vi "Text control 2 v6.2_pump-specific.vi"() -> ()   [LabVIEW 2016]
panel:
  in  "Tab Control":enum32{"Main", "Other parameters"}(tab)
  out "Line running":i32
  out "Total lines":i32
  out "Path":path=path "C:/users/rlp38/09Apr2009LTtesting/test2.txt"
  out "I vs Vg":cluster{"Y data in":dbl[], "X data in":dbl[]}[](graph)
  out "Is max":dbl format="%.2e"
  out "Id max":dbl format="%.2e"
  out "Ig max":dbl format="%.2e"
  out "Imax vs time":cluster{"Y data in":dbl[], "X data in":dbl[]}[](graph)
  out "Imin vs time":cluster{"Y data in":dbl[], "X data in":dbl[]}[](graph)
  out "I vs Vd":cluster{"Y data in":dbl[], "X data in":dbl[]}[](graph)
  in  "Script":string="#-------------------------------------------------------\n# SPM pump cleaning script\n#\n# Version 0.5\n# Author: Dimitrios Simatos\n# Last updated: 2018-01-05\n#-------------------------------------------------------\n# Description\n#\n# This script is designed to run the cleaning sequence of the SPM OEM pump.\n# This script needs to be run 4 times!\n#-------------------------------------------------------\n# Changes\n#\n# Placed initialization and hard stop commands in the beginning.\n#-------------------------------------------------------\n# Important points\n#\n# Never leave any liquid in the pump to dry after the experiments. If they dry, the residue may block the valve.\n# Always run the cleaning cycle after the experiments.\n# Use clockwise rotation when going up in valve port numbers and vice versa.\n#-------------------------------------------------------\n# Things to do before running the script\n#\n# Set time units to minutes.\n# Set filenames.\n# Replace the tubing, if necessary.\n#-------------------------------------------------------\n# Port connections\n#\n# Port 1: Waste\n# Port 2: Waste\n# Port 3: Various cleaning liquids\n# Port 4: Waste\n# Port 5: Waste\n# Port 6: Waste\n#\n# Between each of the 4 runs, the settings of Port 3 will change, according to the cleaning protocol.\n# The settings for Port 3 are:\n# 1st run: 1% v/v solution of sodium hypochlorite in ultrapure water\n# 2nd run: 0.1% w/v solution of sodium dodecyl sulfate in ultrapure water\n# 3rd run: Ultrapure water\n# 4th run: Waste (in air, not immersed in liquid)\n#-------------------------------------------------------\n# Cleaning protocol for the SPM OEM pump (from the manual)\n#\n# A cleaning procedure should be performed at the end of each day or in between two different experiments.\n# An effective cleaning can be performed in the following manner:\n# • Bleach solution to kill microorganisms\n# 1. Prepare a solution of 1% chlorine bleach and deionized water\n#    NOTE: Prepare a 1% v/v solution of sodium hypochlorite in deionized water\n# 2. Prepare a reservoir and place 1 tubing in the bleach solution and 5 tubings in a waste recipient\n# 3. Pick up the bleach solution through 1 port to entirely fill the syringe\n# 4. Sequentially output the syringe content through the remaining ports and throw it to the waste\n# 5. Repeat operation at least 2 times\n# • Detergent solution to remove debris\n# 1. Prepare a solution of 0.1% detergent and deionized water\n#    NOTE: Prepare a 0.1% w/v solution of sodium dodecyl sulfate in deionized water\n# 2. Move the tubing from the bleach solution reservoir and place it into a reservoir of detergent solution\n# 3. Pick up the detergent solution through 1 port to entirely fill the syringe\n# 4. Sequentially output the detergent solution through the remaining ports into the waste recipient\n# 5. Repeat operation at least 2 times\n# • Rinsing water to prepare the pump for your next experiment\n# 1. Move the tubing from the detergent solution reservoir and place it into a reservoir of deionized water\n# 2. Pick up the rinsing solution through 1 port to entirely fill the syringe\n# 3. Sequentially output the rinse water through the remaining ports into the waste recipient\n# 4. Repeat operation at least 2 times\n# • Replace the tubing, if necessary\n#-------------------------------------------------------\n# Pumping cycles and execution time\n#\n# Execution time for a single cycle: 6 x (1 min + 10 sec) = 7 minutes\n# Total execution time: 4 x 7 = 28 minutes\n# Since the script has to run 4 times, the cleaning lasts for: 4 x 28 = 112 minutes\n# Air must be the last to be pumped through the valve, to remove all liquids.\n# There are 4 pumping cycles. Each one draws a different liquid through port 3 and pumps it sequentially through ports 1,2,4,5,6.\n# During the sequential pumping, each port receives 200 ml of liquid (20% of the total syringe volume = 600 \"plunger units\")\n# The device must be disconnected from the port during the cleaning procedure.\n# All cycles are similar, except cycle 1 has the initialization command uncommented and the first report valve command commented.\n#-------------------------------------------------------\n# Volume of liquid needed\n#\n# Volume of liquid needed per cycle: 1 ml\n# Total volume of liquid needed per script run: 4 x 1 = 4 ml\n# Since the script has to run 4 times, the first 3 with different liquids, I need:\n# 4 ml of 1% v/v solution of sodium hypochlorite in ultrapure water\n# 4 ml of 0.1% w/v solution of sodium dodecyl sulfate in ultrapure water\n# 4 ml of ultrapure water\n#-------------------------------------------------------\n# Parameters\n#\n# Syringe size: 1 ml\n# Step resolution N = 0.01 mm\n# Drawing flow V = 300 pulses/second (6000 ul/min)\n# Pumping flow V = 300 pulses/second (6000 ul/min)\n#-------------------------------------------------------\n# Pump initialization\npump /1T #hard stop pump\npump /1ZR #initialize pump\n#-------------------------------------------------------\n# Cycle 1\n# Fill the syringe\npump /1Q #query pump\npump /1? #report absolute plunger position\n#pump /1?6 #report valve position\nwait-min 1 #wait 1 minute\npump /1N0R #set step resolution: 0.01 mm\npump /1Q #query pump\npump /1? #report absolute plunger position (the plunger should be at 0)\npump /1?6 #report valve position\nwait 1000 #wait 1 second\npump /1V300R #choose speed: 300 steps/s (6000 ul/min)\npump /1Q #query pump\nwait 1000 #wait 1 second\npump /1I3R #go to port 3, clockwise rotation\npump /1Q #query pump\npump /1?6 #report valve position\nwait 1000 #wait 1 second\npump /1A3000R #go to absolute position 3000 (= draw 1 ml)\nwait 30000 #wait 30 seconds\npump /1Q #query pump\npump /1? #report absolute plunger position (the plunger should have finished moving)\n#pump /1?6 #report valve position\n# The sequential pumping begins\n# Port 1\npump /1O1R #switch to port 1, counterclockwise rotation\npump /1Q #query pump\npump /1?6 #report valve position\npump /1A2400R #go to absolute position 2400 (= pump 200 ul)\npump /1Q #query pump\npump /1? #report absolute plunger position (the plunger should be moving to 0)\nwait-min 1 #wait 1 minute\npump /1? #report absolute plunger position (the plunger should have finished moving)\n# Port 2\npump /1I2R #switch to port 2, clockwise rotation\npump /1Q #query pump\npump /1?6 #report valve position\npump /1A1800R #go to absolute position 1800 (= pump 200 ul)\npump /1Q #query pump\npump /1? #report absolute plunger position (the plunger should be moving to 0)\nwait-min 1 #wait 1 minute\npump /1? #report absolute plunger position (the plunger should have finished moving)\n# Port 4\npump /1I4R #switch to port 4, clockwise rotation\npump /1Q #query pump\npump /1?6 #report valve position\npump /1A1200R #go to absolute position 1200 (= pump 200 ul)\npump /1Q #query pump\npump /1? #report absolute plunger position (the plunger should be moving to 0)\nwait-min 1 #wait 1 minute\npump /1? #report absolute plunger position (the plunger should have finished moving)\n# Port 5\npump /1I5R #switch to port 5, clockwise rotation\npump /1Q #query pump\npump /1?6 #report valve position\npump /1A600R #go to absolute position 600 (= pump 200 ul)\npump /1Q #query pump\npump /1? #report absolute plunger position (the plunger should be moving to 0)\nwait-min 1 #wait 1 minute\npump /1? #report absolute plunger position (the plunger should have finished moving)\n# Port 6\npump /1I6R #switch to port 6, clockwise rotation\npump /1Q #query pump\npump /1?6 #report valve position\npump /1A0R #go to absolute position 0 (= pump 200 ul)\npump /1Q #query pump\npump /1? #report absolute plunger position (the plunger should be moving to 0)\nwait-min 1 #wait 1 minute\npump /1? #report absolute plunger position (the plunger should have finished moving)\n#-------------------------------------------------------\n# Cycle 2\n# Fill the syringe\n#pump /1ZR #initialize pump\npump /1Q #query pump\npump /1? #report absolute plunger position\npump /1?6 #report valve position\nwait-min 1 #wait 1 minute\npump /1N0R #set step resolution: 0.01 mm\npump /1Q #query pump\npump /1? #report absolute plunger position (the plunger should be at 0)\npump /1?6 #report valve position\nwait 1000 #wait 1 second\npump /1V300R #choose speed: 300 steps/s (6000 ul/min)\npump /1Q #query pump\nwait 1000 #wait 1 second\npump /1O3R #go to port 3, counterclockwise rotation\npump /1Q #query pump\npump /1?6 #report valve position\nwait 1000 #wait 1 second\npump /1A3000R #go to absolute position 3000 (= draw 1 ml)\nwait 30000 #wait 30 seconds\npump /1Q #query pump\npump /1? #report absolute plunger position (the plunger should have finished moving)\n#pump /1?6 #report valve position\n# The sequential pumping begins\n# Port 1\npump /1O1R #switch to port 1, counterclockwise rotation\npump /1Q #query pump\npump /1?6 #report valve position\npump /1A2400R #go to absolute position 2400 (= pump 200 ul)\npump /1Q #query pump\npump /1? #report absolute plunger position (the plunger should be moving to 0)\nwait-min 1 #wait 1 minute\npump /1? #report absolute plunger position (the plunger should have finished moving)\n# Port 2\npump /1I2R #switch to port 2, clockwise rotation\npump /1Q #query pump\npump /1?6 #report valve position\npump /1A1800R #go to absolute position 1800 (= pump 200 ul)\npump /1Q #query pump\npump /1? #report absolute plunger position (the plunger should be moving to 0)\nwait-min 1 #wait 1 minute\npump /1? #report absolute plunger position (the plunger should have finished moving)\n# Port 4\npump /1I4R #switch to port 4, clockwise rotation\npump /1Q #query pump\npump /1?6 #report valve position\npump /1A1200R #go to absolute position 1200 (= pump 200 ul)\npump /1Q #query pump\npump /1? #report absolute plunger position (the plunger should be moving to 0)\nwait-min 1 #wait 1 minute\npump /1? #report absolute plunger position (the plunger should have finished moving)\n# Port 5\npump /1I5R #switch to port 5, clockwise rotation\npump /1Q #query pump\npump /1?6 #report valve position\npump /1A600R #go to absolute position 600 (= pump 200 ul)\npump /1Q #query pump\npump /1? #report absolute plunger position (the plunger should be moving to 0)\nwait-min 1 #wait 1 minute\npump /1? #report absolute plunger position (the plunger should have finished moving)\n# Port 6\npump /1I6R #switch to port 6, clockwise rotation\npump /1Q #query pump\npump /1?6 #report valve position\npump /1A0R #go to absolute position 0 (= pump 200 ul)\npump /1Q #query pump\npump /1? #report absolute plunger position (the plunger should be moving to 0)\nwait-min 1 #wait 1 minute\npump /1? #report absolute plunger position (the plunger should have finished moving)\n#-------------------------------------------------------\n# Cycle 3\n# Fill the syringe\n#pump /1ZR #initialize pump\npump /1Q #query pump\npump /1? #report absolute plunger position\npump /1?6 #report valve position\nwait-min 1 #wait 1 minute\npump /1N0R #set step resolution: 0.01 mm\npump /1Q #query pump\npump /1? #report absolute plunger position (the plunger should be at 0)\npump /1?6 #report valve position\nwait 1000 #wait 1 second\npump /1V300R #choose speed: 300 steps/s (6000 ul/min)\npump /1Q #query pump\nwait 1000 #wait 1 second\npump /1O3R #go to port 3, counterclockwise rotation\npump /1Q #query pump\npump /1?6 #report valve position\nwait 1000 #wait 1 second\npump /1A3000R #go to absolute position 3000 (= draw 1 ml)\nwait 30000 #wait 30 seconds\npump /1Q #query pump\npump /1? #report absolute plunger position (the plunger should have finished moving)\n#pump /1?6 #report valve position\n# The sequential pumping begins\n# Port 1\npump /1O1R #switch to port 1, counterclockwise rotation\npump /1Q #query pump\npump /1?6 #report valve position\npump /1A2400R #go to absolute position 2400 (= pump 200 ul)\npump /1Q #query pump\npump /1? #report absolute plunger position (the plunger should be moving to 0)\nwait-min 1 #wait 1 minute\npump /1? #report absolute plunger position (the plunger should have finished moving)\n# Port 2\npump /1I2R #switch to port 2, clockwise rotation\npump /1Q #query pump\npump /1?6 #report valve position\npump /1A1800R #go to absolute position 1800 (= pump 200 ul)\npump /1Q #query pump\npump /1? #report absolute plunger position (the plunger should be moving to 0)\nwait-min 1 #wait 1 minute\npump /1? #report absolute plunger position (the plunger should have finished moving)\n# Port 4\npump /1I4R #switch to port 4, clockwise rotation\npump /1Q #query pump\npump /1?6 #report valve position\npump /1A1200R #go to absolute position 1200 (= pump 200 ul)\npump /1Q #query pump\npump /1? #report absolute plunger position (the plunger should be moving to 0)\nwait-min 1 #wait 1 minute\npump /1? #report absolute plunger position (the plunger should have finished moving)\n# Port 5\npump /1I5R #switch to port 5, clockwise rotation\npump /1Q #query pump\npump /1?6 #report valve position\npump /1A600R #go to absolute position 600 (= pump 200 ul)\npump /1Q #query pump\npump /1? #report absolute plunger position (the plunger should be moving to 0)\nwait-min 1 #wait 1 minute\npump /1? #report absolute plunger position (the plunger should have finished moving)\n# Port 6\npump /1I6R #switch to port 6, clockwise rotation\npump /1Q #query pump\npump /1?6 #report valve position\npump /1A0R #go to absolute position 0 (= pump 200 ul)\npump /1Q #query pump\npump /1? #report absolute plunger position (the plunger should be moving to 0)\nwait-min 1 #wait 1 minute\npump /1? #report absolute plunger position (the plunger should have finished moving)\n#-------------------------------------------------------\n# Cycle 4\n# Fill the syringe\n#pump /1ZR #initialize pump\npump /1Q #query pump\npump /1? #report absolute plunger position\npump /1?6 #report valve position\nwait-min 1 #wait 1 minute\npump /1N0R #set step resolution: 0.01 mm\npump /1Q #query pump\npump /1? #report absolute plunger position (the plunger should be at 0)\npump /1?6 #report valve position\nwait 1000 #wait 1 second\npump /1V300R #choose speed: 300 steps/s (6000 ul/min)\npump /1Q #query pump\nwait 1000 #wait 1 second\npump /1O3R #go to port 3, counterclockwise rotation\npump /1Q #query pump\npump /1?6 #report valve position\nwait 1000 #wait 1 second\npump /1A3000R #go to absolute position 3000 (= draw 1 ml)\nwait 30000 #wait 30 seconds\npump /1Q #query pump\npump /1? #report absolute plunger position (the plunger should have finished moving)\n#pump /1?6 #report valve position\n# The sequential pumping begins\n# Port 1\npump /1O1R #switch to port 1, counterclockwise rotation\npump /1Q #query pump\npump /1?6 #report valve position\npump /1A2400R #go to absolute position 2400 (= pump 200 ul)\npump /1Q #query pump\npump /1? #report absolute plunger position (the plunger should be moving to 0)\nwait-min 1 #wait 1 minute\npump /1? #report absolute plunger position (the plunger should have finished moving)\n# Port 2\npump /1I2R #switch to port 2, clockwise rotation\npump /1Q #query pump\npump /1?6 #report valve position\npump /1A1800R #go to absolute position 1800 (= pump 200 ul)\npump /1Q #query pump\npump /1? #report absolute plunger position (the plunger should be moving to 0)\nwait-min 1 #wait 1 minute\npump /1? #report absolute plunger position (the plunger should have finished moving)\n# Port 4\npump /1I4R #switch to port 4, clockwise rotation\npump /1Q #query pump\npump /1?6 #report valve position\npump /1A1200R #go to absolute position 1200 (= pump 200 ul)\npump /1Q #query pump\npump /1? #report absolute plunger position (the plunger should be moving to 0)\nwait-min 1 #wait 1 minute\npump /1? #report absolute plunger position (the plunger should have finished moving)\n# Port 5\npump /1I5R #switch to port 5, clockwise rotation\npump /1Q #query pump\npump /1?6 #report valve position\npump /1A600R #go to absolute position 600 (= pump 200 ul)\npump /1Q #query pump\npump /1? #report absolute plunger position (the plunger should be moving to 0)\nwait-min 1 #wait 1 minute\npump /1? #report absolute plunger position (the plunger should have finished moving)\n# Port 6\npump /1I6R #switch to port 6, clockwise rotation\npump /1Q #query pump\npump /1?6 #report valve position\npump /1A0R #go to absolute position 0 (= pump 200 ul)\npump /1Q #query pump\npump /1? #report absolute plunger position (the plunger should be moving to 0)\nwait-min 1 #wait 1 minute\npump /1? #report absolute plunger position (the plunger should have finished moving)\n#-------------------------------------------------------"
  out "Command running:":string
  out "Serial port data":string
  out "Elapsed Time":dbl caption="Elapsed Time (s)"
  in  "Time Units":u16(ring)=1 items=["Seconds", "Minutes", "Hours"]
  in  "Time Offset":dbl caption="Set Start Time (s)"
  in  "Reset":bool
  in  "Auto Reset":bool
  in  "integration time":u32(slide) max=2 step=1 scale=0.0..2.0
  in  "Interrupt scan":bool
  out "Absolute plunger position vs time":cluster{"Y data in":dbl[], "X data in":dbl[]}[](graph)
  out "Valve position vs time":cluster{"Y data in":dbl[], "X data in":dbl[]}[](graph)
  out "Is on":dbl format="%.2e"
  out "Id on":dbl format="%.2e"
  out "Ig on":dbl format="%.2e"
  out "Ion vs time":cluster{"Y data in":dbl[], "X data in":dbl[]}[](graph)
  out "Ioff vs time":cluster{"Y data in":dbl[], "X data in":dbl[]}[](graph)
  out "Ig min":dbl format="%.2e"
  out "Id min":dbl format="%.2e"
  out "Is min":dbl format="%.2e"
  out "Is off":dbl format="%.2e"
  out "Id off":dbl format="%.2e"
  out "Ig off":dbl format="%.2e"
  in  "Integration time (long)":dbl=0.32 min=0.04 max=2.0 step=0.02 format="%.2f"
  in  "Integration time (short)":dbl=0.0019 min=8e-05 max=0.0019 step=8e-05 format="%^.0e"
  in  "Gate: Compliance":dbl=0.001 format="%.8f"
  in  "Drain: Compliance":dbl=0.001 format="%.8f"
  in  "Hard stop pump":bool
  in  "Halt pump":bool
  in  "Interrupt program":bool
  in  "Gate Range\nmode":u16(ring) items=["Auto", "Limited", "Fixed"]
  in  "Gate Range":u8(slide)=6 max=11 scale=0.0..11.0
  in  "Source/Drain\nRange mode":u16(ring) items=["Auto", "Limited", "Fixed"]
  in  "Source/Drain Range":u8(slide)=6 max=11 scale=0.0..11.0
  in  "Panel Controls":T1={"Emergency Stop"=refnum, "TransGraph Max"=1e-05, "Text/Graph (text=false)"=TRUE} {"TransGraph Max" format="%.2e"}
  in  "Panel Controls 2":T2={"Emergency Stop"=refnum, "TransGraph Max"=1e-05, "Text/Graph (text=false)"=TRUE, "TransGraph Min"=1e-11} {"TransGraph Min" format="%.2e"; "TransGraph Max" format="%.2e"}
  in  "SMU4":cluster{"on/off":bool, "Voltage":dbl} {"Voltage" min=-100.0 max=100.0 format="%.2f"}
  in  "Full Reset":bool
  in  "Standby":T3
  out "error out":errorcluster
  in  "Delay before read (ms)":u32=1000
  in  "byte count":u32=64
  in  "Serial End Mode for Reads":u16(ring)=2 items=["None", "LastBit", "TermChar"]
  in  "Timeout (ms)":u32=10000
  in  "Enable Termination\nChar (T)":bool=TRUE
  in  "Termination char\n(0xA = '\\n' = LF)\n(0xD = '\\r' = CR)":u8=13 format="%.0x"
  in  "flow control":u16(ring) items=["None"=0, "XON/XOFF"=1, "RTS/CTS"=2, "DTR/DSR"=4]
  in  "stop bits":u16(ring)=10 items=["1.0"=10, "1.5"=15, "2.0"=20]
  in  "parity":u16(ring) items=["None", "Odd", "Even", "Mark", "Space"]
  in  "data bits":u16=8 min=5 max=8 step=1
  in  "VISA resource name":refnum<visa-resource-name>="COM6"
  in  "baud rate":u32=9600
  in  "Filename (variable part)":string="step_1_up-H2O_initial_"
  in  "Suffix (script)":string="step_1_up-H2O_initial_script.txt"
  out "Timings Indicator":T4
  in  "Timings (overwritten by the Front Panel)":T5={"integration time"=0, "Short/Long integration time"=0.00064, "hold time (sec)"=0.0, "delay time (sec)"=0.0, "Step Time (0 disables)"=0.0, "sweep method"=0, "Pulse period"=0.005, "Base voltage"=0.0, "Pulse width"=0.0005} {"Pulse width" min=0.0005 max=0.1 step=0.0001 format="%.4f"; "Base voltage" format="%^.4e"; "Pulse period" min=0.005 max=1.0 step=0.0001 format="%.4f"; "sweep method" items=["Continuous", "Pulsed"]; "Step Time (0 disables)" format="%.2f"; "delay time (sec)" format="%.4f"; "hold time (sec)" format="%.4f"; "Short/Long integration time" format="%^.0e"; "integration time" scale=0.0..2.0}
  in  "Gate":T6={"Gate Start"=0.0, "Gate Stop"=2.0, "Gate Step (linear only)"=1.0, "Gate Compliance"=0.0001, "Gate PComp"=0.0, "Range mode"=0, "Range"=6} {"Range" max=11 scale=0.0..11.0; "Range mode" items=["Auto", "Limited", "Fixed"]; "Gate PComp" format="%^.2e"; "Gate Compliance" format="%^.2e"; "Gate Step (linear only)" format="%^.4e"; "Gate Stop" format="%^.4e"; "Gate Start" format="%^.4e"}
  in  "Drain 2":T7={"Drain Start"=0.0, "Drain Stop"=2.0, "Drain Compliance"=0.0001, "Drain Step"=1.0, "Drain PComp"=0.0, "Range mode"=0, "Range"=6} {"Range" max=11 scale=0.0..11.0; "Range mode" items=["Auto", "Limited", "Fixed"]; "Drain PComp" format="%^.2e"; "Drain Step" format="%^.4e"; "Drain Compliance" format="%^.2e"; "Drain Stop" format="%^.4e"; "Drain Start" format="%^.4e"}
  # "Syntax:\nitime [s|m|l] time(sec): [s|m|l] determines the integration time setting (small|medium|long) and time sets the value.\nNOTE: The value of the integration time has to be within the range allowed by its category (s|m|l), otherwise, the closest value will be used. (e.g. if the category is set to short but the time value is very long, the actual value used will be the maximum short integration time.\nIntegration times:\n    Short: Default: 640 us. Range: 8E-5 - 1.92E-3 seconds.\n    Medium: Fixed at 1 NPL cycle (0.02 seconds).\n    Long: Default: 16 NPL cycles (0.32 seconds). Range: 2-100 NPL cycles (0.04 seconds - 2 seconds).\ngaterangemode [a|l|f]\ndrainrangemode [a|l|f]\npulsed [on|off] PulsePeriod(sec) PulseBaseVoltage PulseONWidth(sec)\nstandby [on l off]\nwait NumMilliseconds\nwait-min NumMinutes\n# texthere = comment\ntransfer [s|d] VgStart VgStop VgStep VdStart VdStop VdStep\noutput [s|d] VgStart VgStop VgStep VdStart VdStop VdStep\nsample Vg Vd NumSamples Time(s) SampleInterval(s)\nsamplei Idg NumSamples Time(s) SampleInterval(s) VDGcompliance\n100 samples is approximately 13 seconds with medium integration\n# if in doubt use SampleInterval(s) = 0.004\nstressV VG VD IGcompliance IDcompliance Duration(sec)\nstressI IDG VDGcompliance Duration(sec)\nvsu2pulse Bias Duration(s)\npulsedstressV [s|d] VEstop VgON VgOFF Period(s) PulseONwidth(s) Vd\nsample-fpp Vg Vd NumSamples Time\nresample-fpp Vg Vd\ntransfer-fpp [s|d] VgStart VgStop VgStep VdStart VdStop VdStep\noutput-fpp [s|d] VgStart VgStop VgStep VdStart VdStop VdStep\nserial SerialPortCommand\npump SerialPortCommand for the SPM pump\n\nSPM Pump Syntax (<x>: pump number, use 1 if only one pump):\nif the command syntax contains [R], then append the letter R to the command\n/<x>Q: query (a query command should follow each command)\n/<x>Z[R] or /<x>Y[R]: initialize pump\n/<x>N<n>[R] (<n>=0,1): <0> (<1>) microstep 0.01 mm (0.00125 mm) resolution\n/<x>I<n> (<n>=0-6): turn to port number n (clockwise)\n/<x>O<n> (<n>=0-6): turn to port number n (counterclockwise)\n/<x>X: Re-execute last command string\n/<x>G<n>[R] (<n>=0-60000): repeat command sequence (default: 0, 0=loop forever)\n/<x>g: Mark the start of a repeat sequence (max = 10)\n/<x>M<n>[R] (<n>=0-86400000): delay command execution by n milliseconds\n/<x>H: Halt; Pause the sequence after finishing the current move\n/<x>T: Hardstop; Interrupt the current move and suppress it from the sequence\n/<x>A<n>[R] (<n>=0-3000 with N=0, 0-24000 with N=1): absolute position\n/<x>P<n>[R] (<n>=0-3000 with N=0, 0-24000 with N=1): relative pickup\n/<x>D<n>[R] (<n>=0-3000 with N=0, 0-24000 with N=1): relative dispense\n/<x>V<n>[R] (<n>=1-1600 default: 150): set peak speed (pulses/sec)\nNOTE: The lowest speed limit is 1 pulse/sec, not 5, as the manual states.\n/<x>S<n>[R] (<n>=10-40 default: 22): set speed (NOT in pulses/sec, look in manual)\nNOTE: When controlled with absolute position, one does not need to pay special attention to the syringe that is mounted on the pump.\nWithdraw from lower stage (ports 3, 5), dispense from higher stage (ports 2, 4, 6).\nConnect Port 1 to waste."
  # "Time"
  # "1\n2\n3\n4\n5\n6\n7\n8\n9\n10\n11\n12\n13\n14\n15\n16\n17\n18\n19\n20"
  # "Serial port settings"
  # "Filename settings"
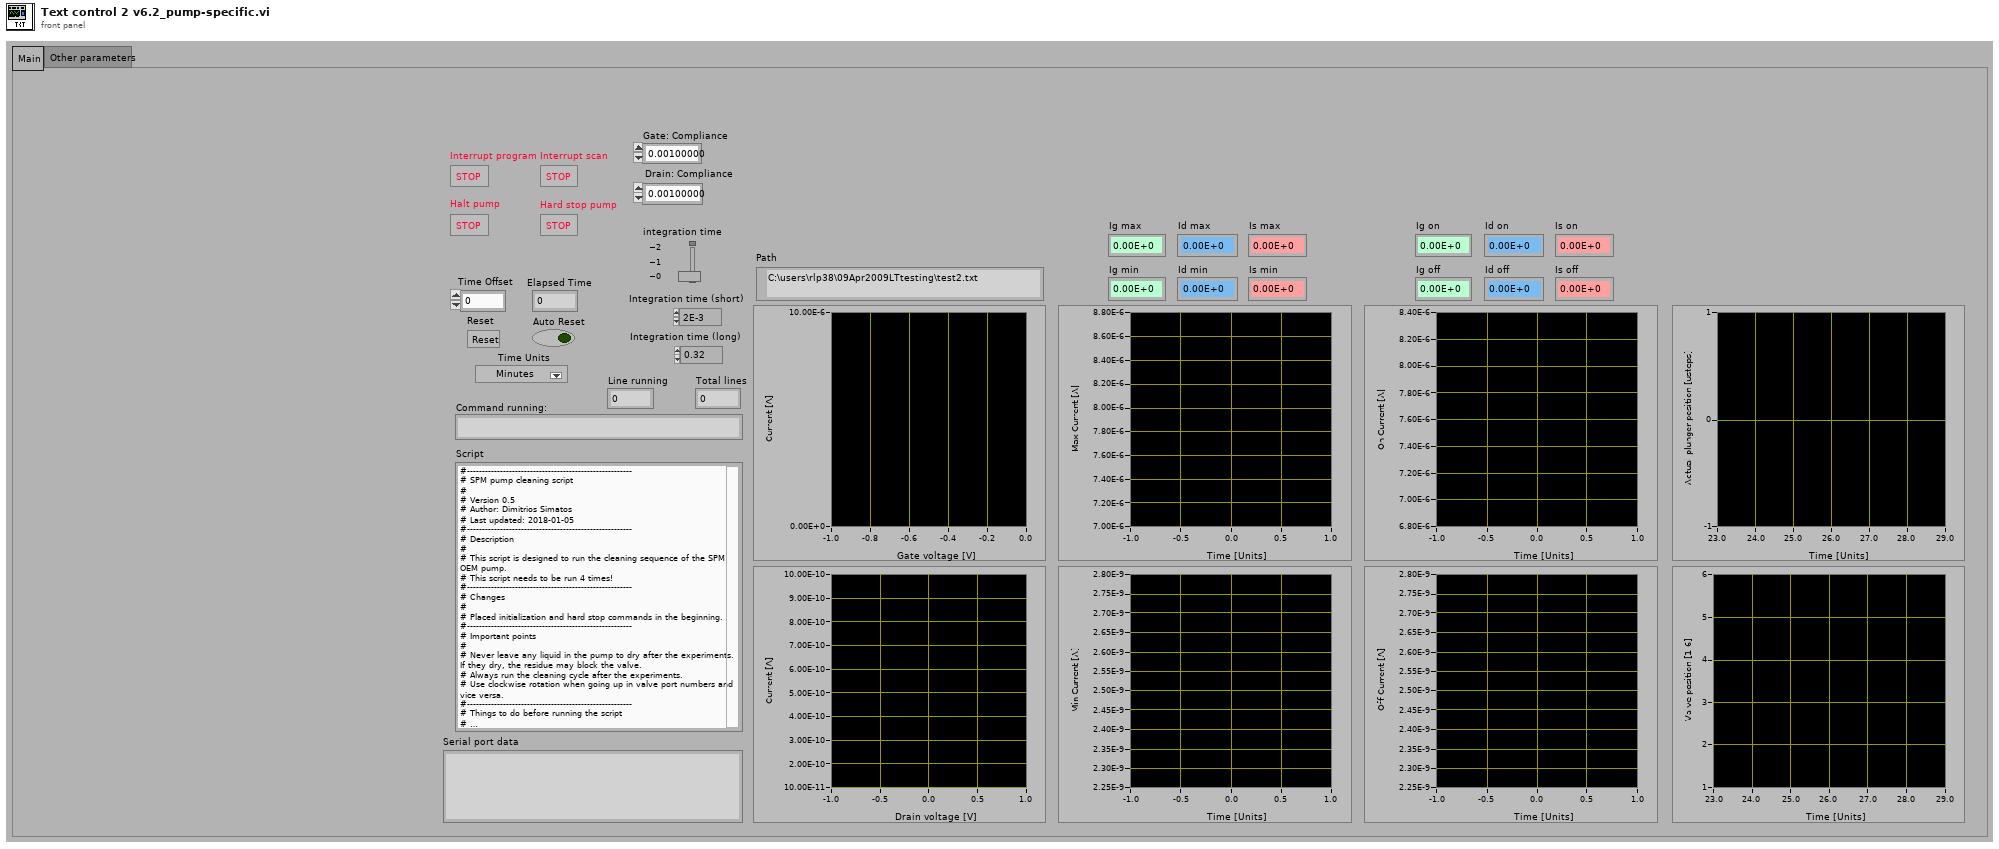
[diagram p1: front panel]
types:
  T1 = cluster{"Emergency Stop":refnum<vi>, "TransGraph Max":dbl, "Text/Graph (text=false)":bool}
  T2 = cluster{"Emergency Stop":refnum<vi>, "TransGraph Max":dbl, "Text/Graph (text=false)":bool, "TransGraph Min":dbl}
  T3 = cluster{"Gate Standby":bool, "Drain Standby":bool}
  T4 = cluster{"integration time (0:s, 1:m, 2:l)":u32, "Short/Long integration time":dbl, "hold time (sec)":dbl, "delay time (sec)":dbl, "Step Time (0 disables)":dbl, "sweep method":u16, "Pulse period":dbl, "Base voltage":dbl, "Pulse width":dbl}
  T5 = cluster{"integration time":u32, "Short/Long integration time":dbl, "hold time (sec)":dbl, "delay time (sec)":dbl, "Step Time (0 disables)":dbl, "sweep method":u16, "Pulse period":dbl, "Base voltage":dbl, "Pulse width":dbl}
  T6 = cluster{"Gate Start":dbl, "Gate Stop":dbl, "Gate Step (linear only)":dbl, "Gate Compliance":dbl, "Gate PComp":dbl, "Range mode":u16, "Range":u8}
  T7 = cluster{"Drain Start":dbl, "Drain Stop":dbl, "Drain Compliance":dbl, "Drain Step":dbl, "Drain PComp":dbl, "Range mode":u16, "Range":u8}
  T8 = enum16{"open", "replace", "create", "open or create", "replace or create", "replace or create with confirmation"}
  T9 = cluster{"V2 Start":dbl, "V2 Step":dbl, "Number of points":i32}
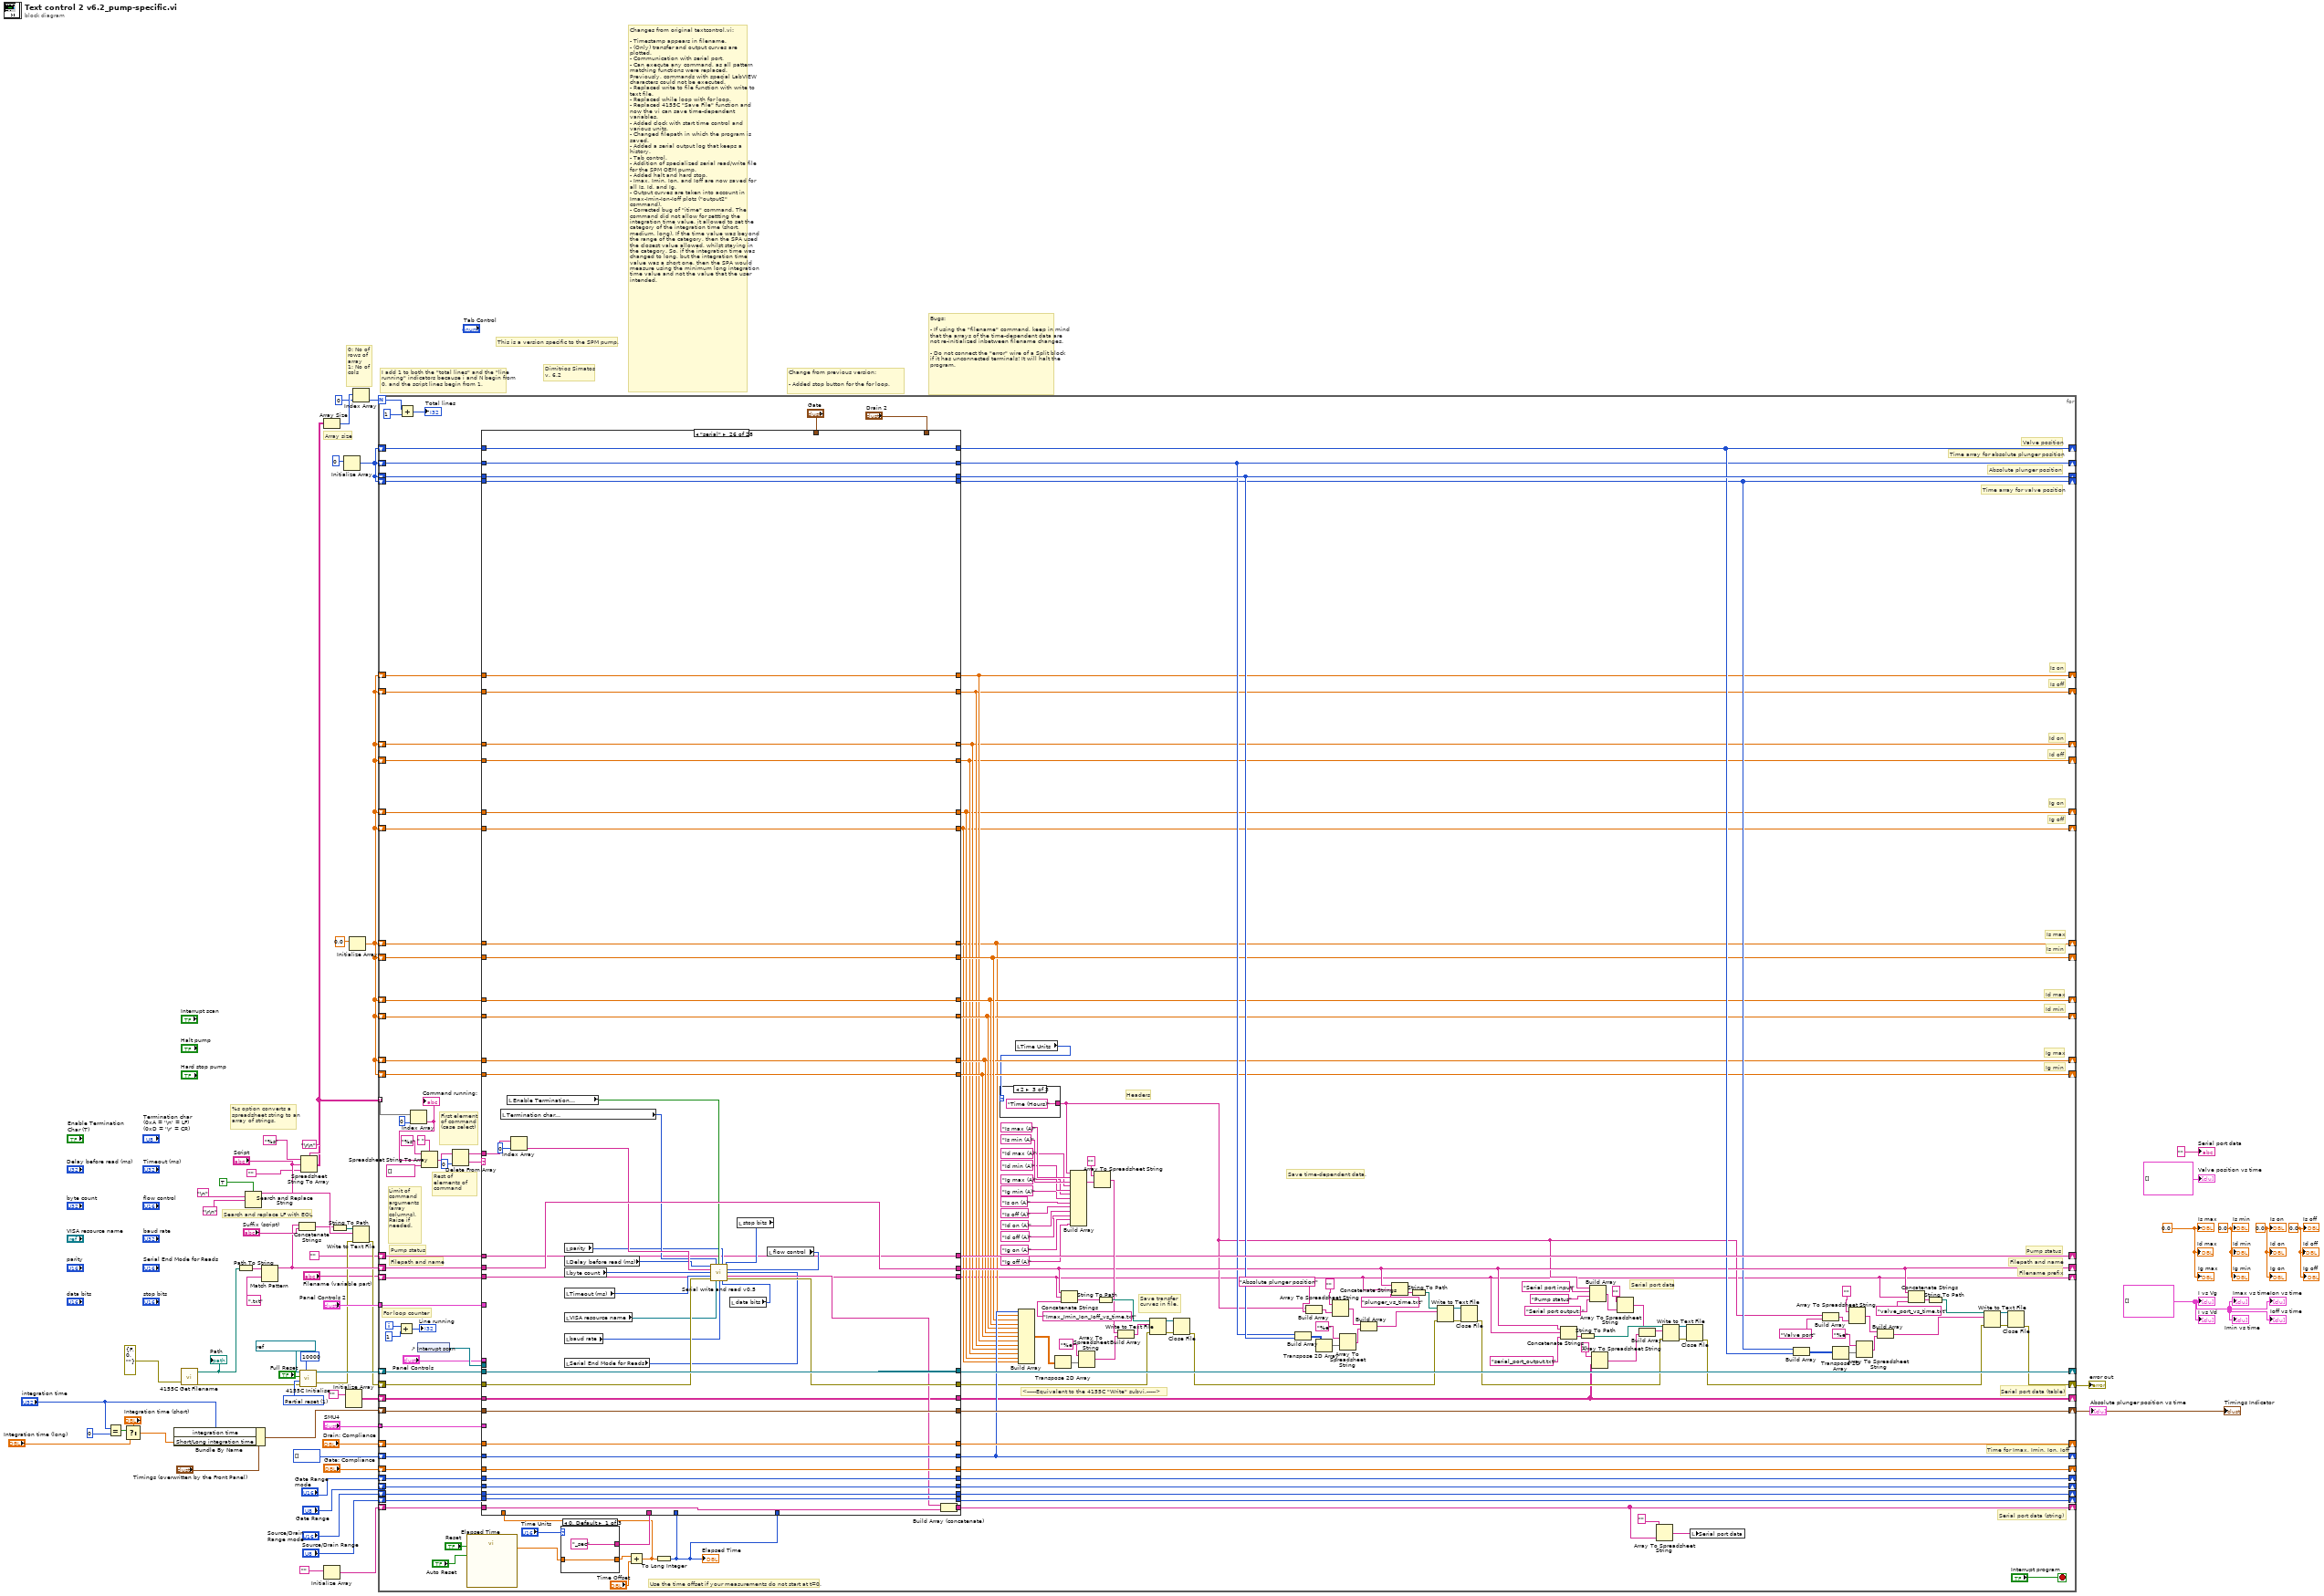
[diagram p0: block diagram]
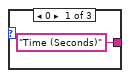
[diagram p2: hidden frame]
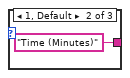
[diagram p3: hidden frame]
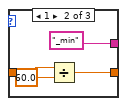
[diagram p4: hidden frame]
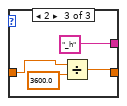
[diagram p5: hidden frame]
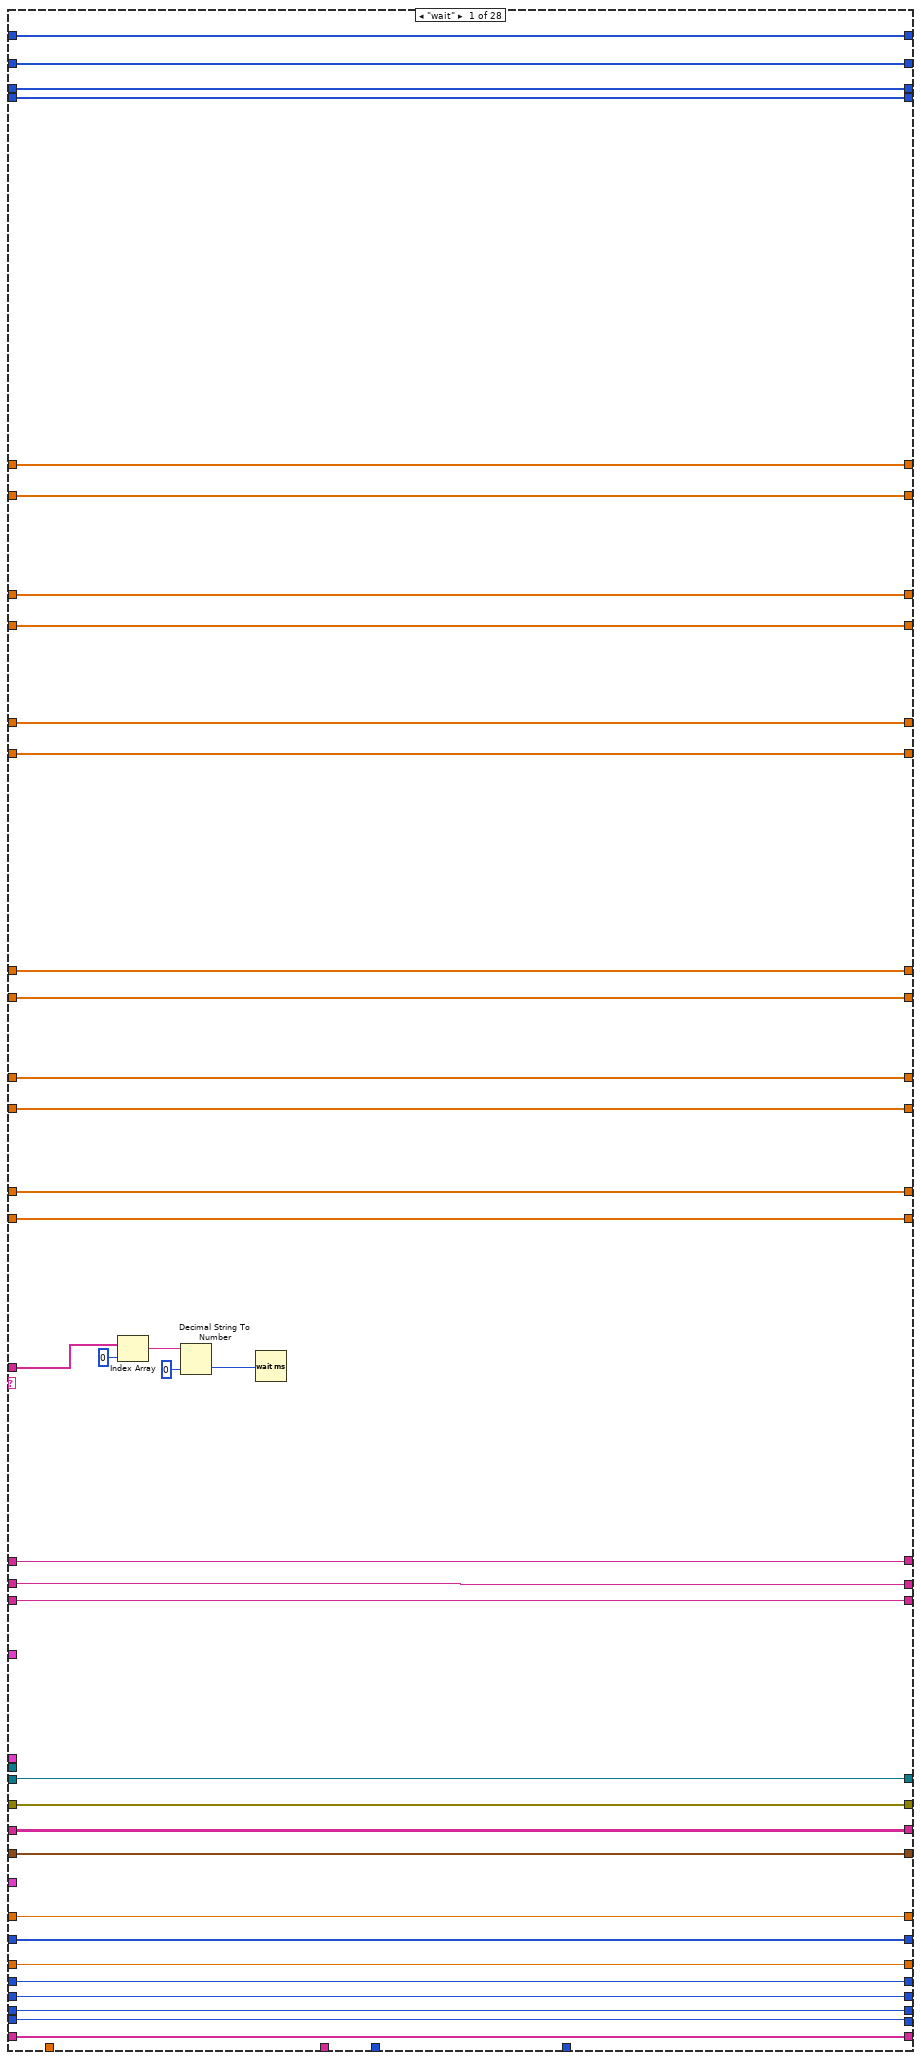
[diagram p6: hidden frame]
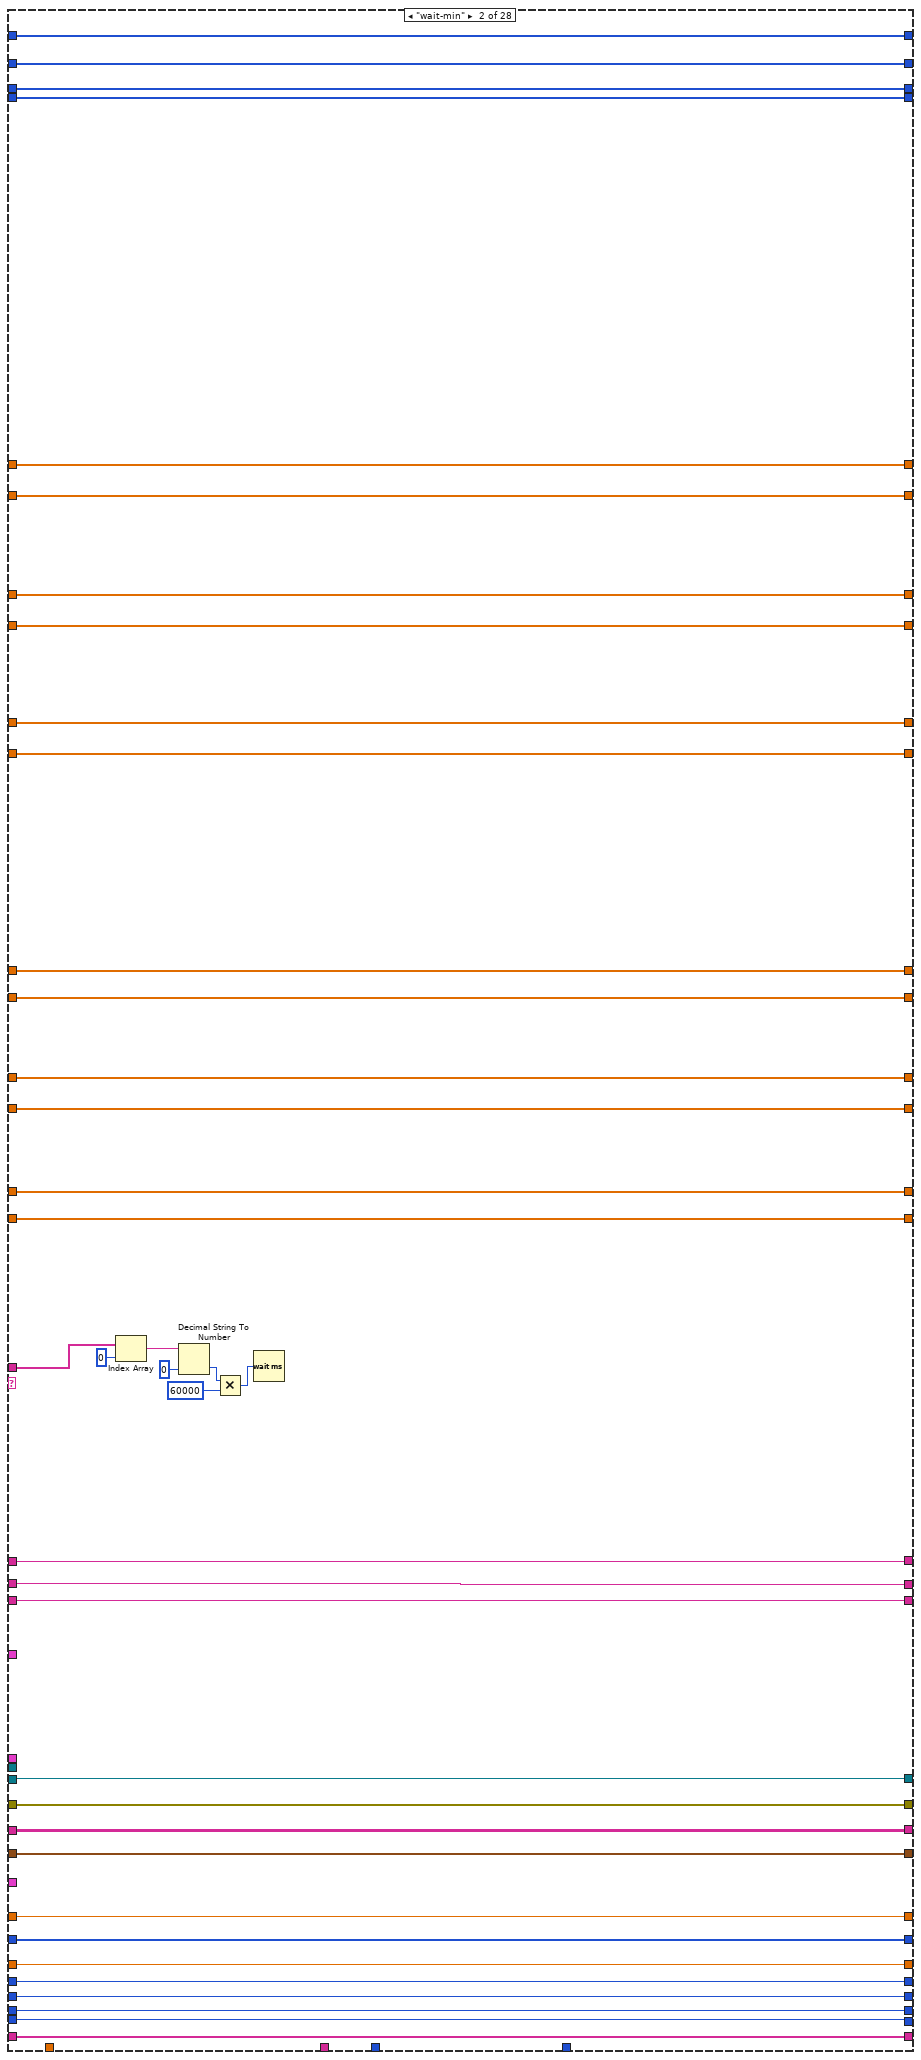
[diagram p7: hidden frame]
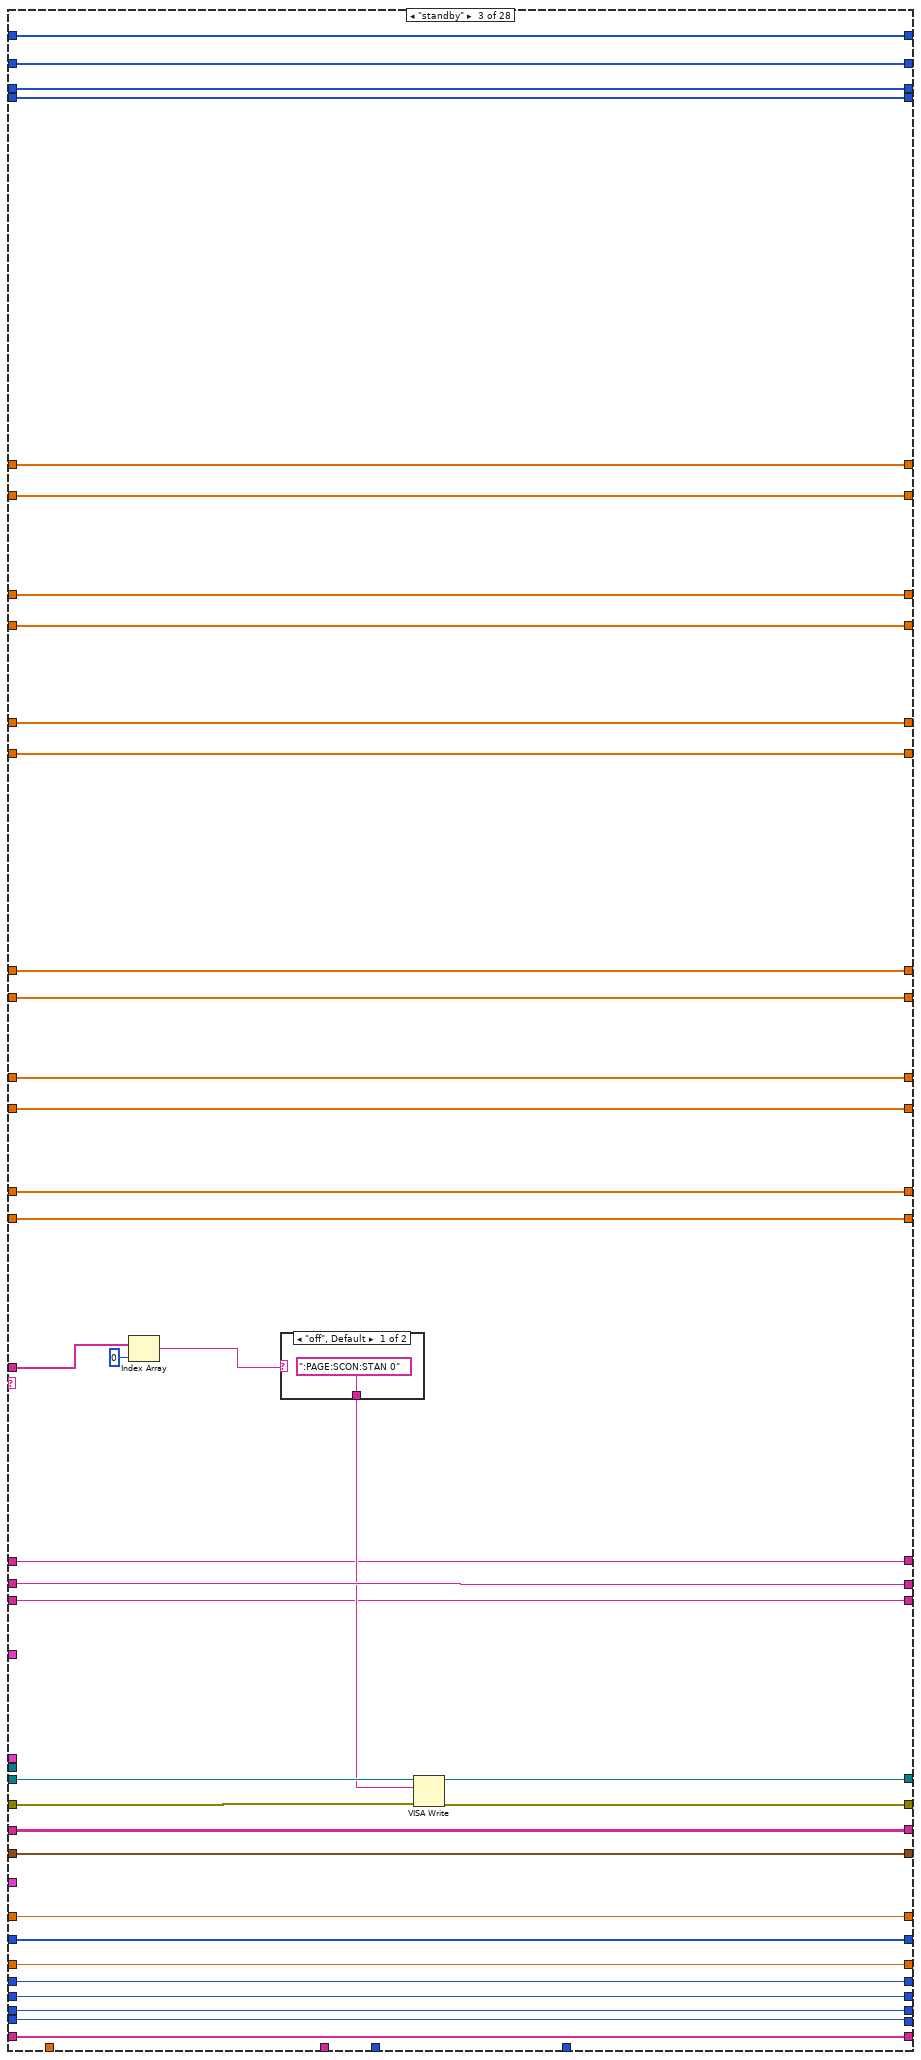
[diagram p8: hidden frame]
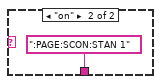
[diagram p9: hidden frame]
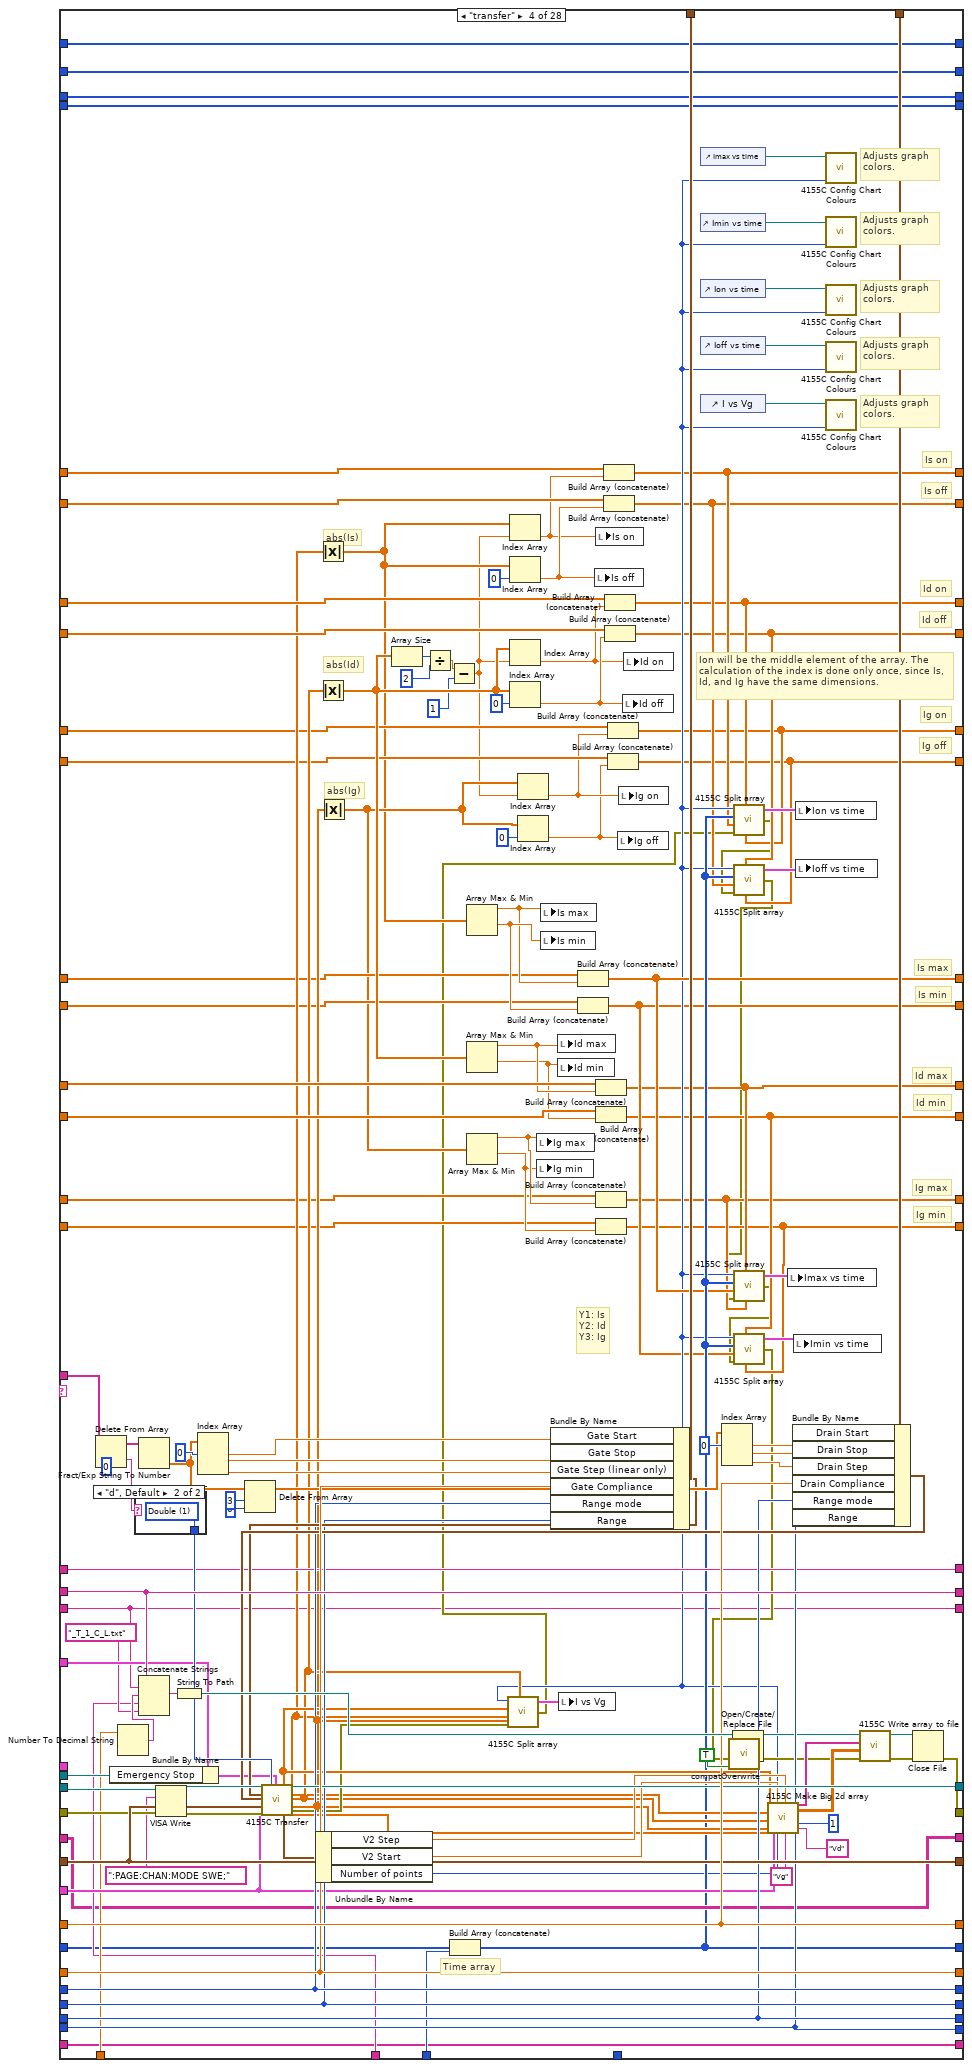
[diagram p10: hidden frame]
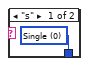
[diagram p11: hidden frame]
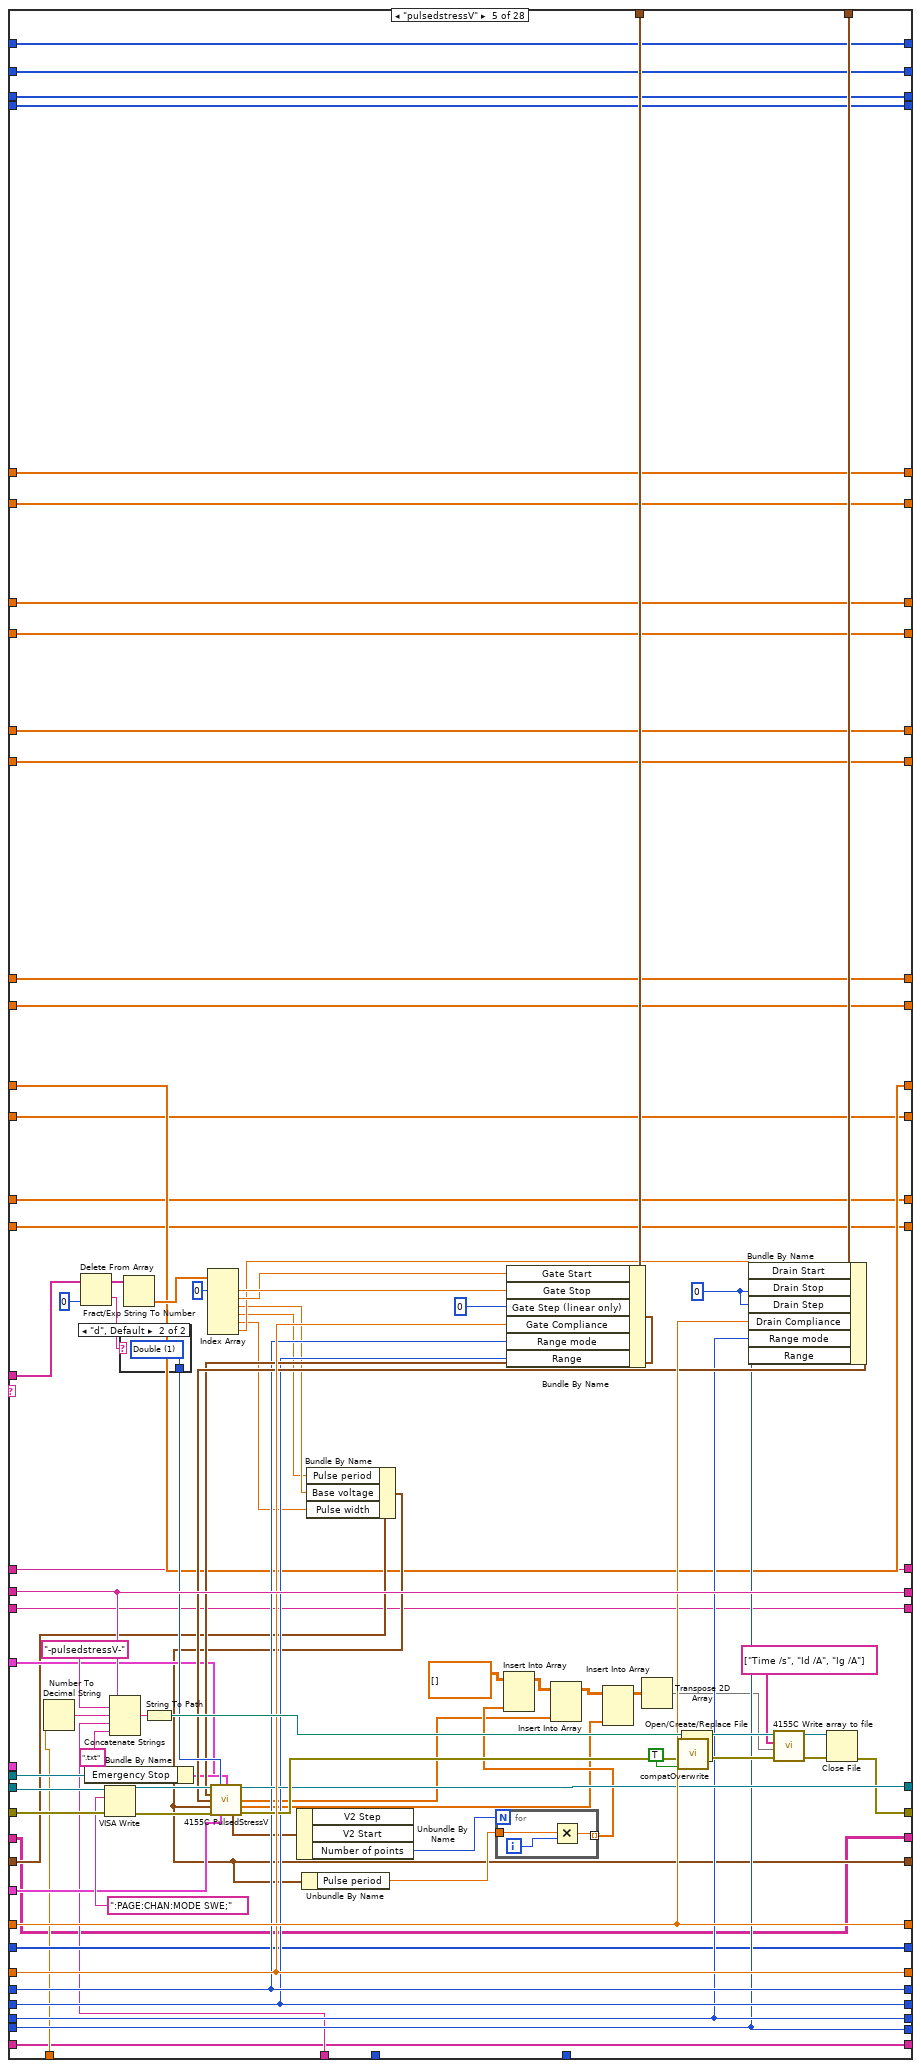
[diagram p12: hidden frame]
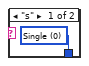
[diagram p13: hidden frame]
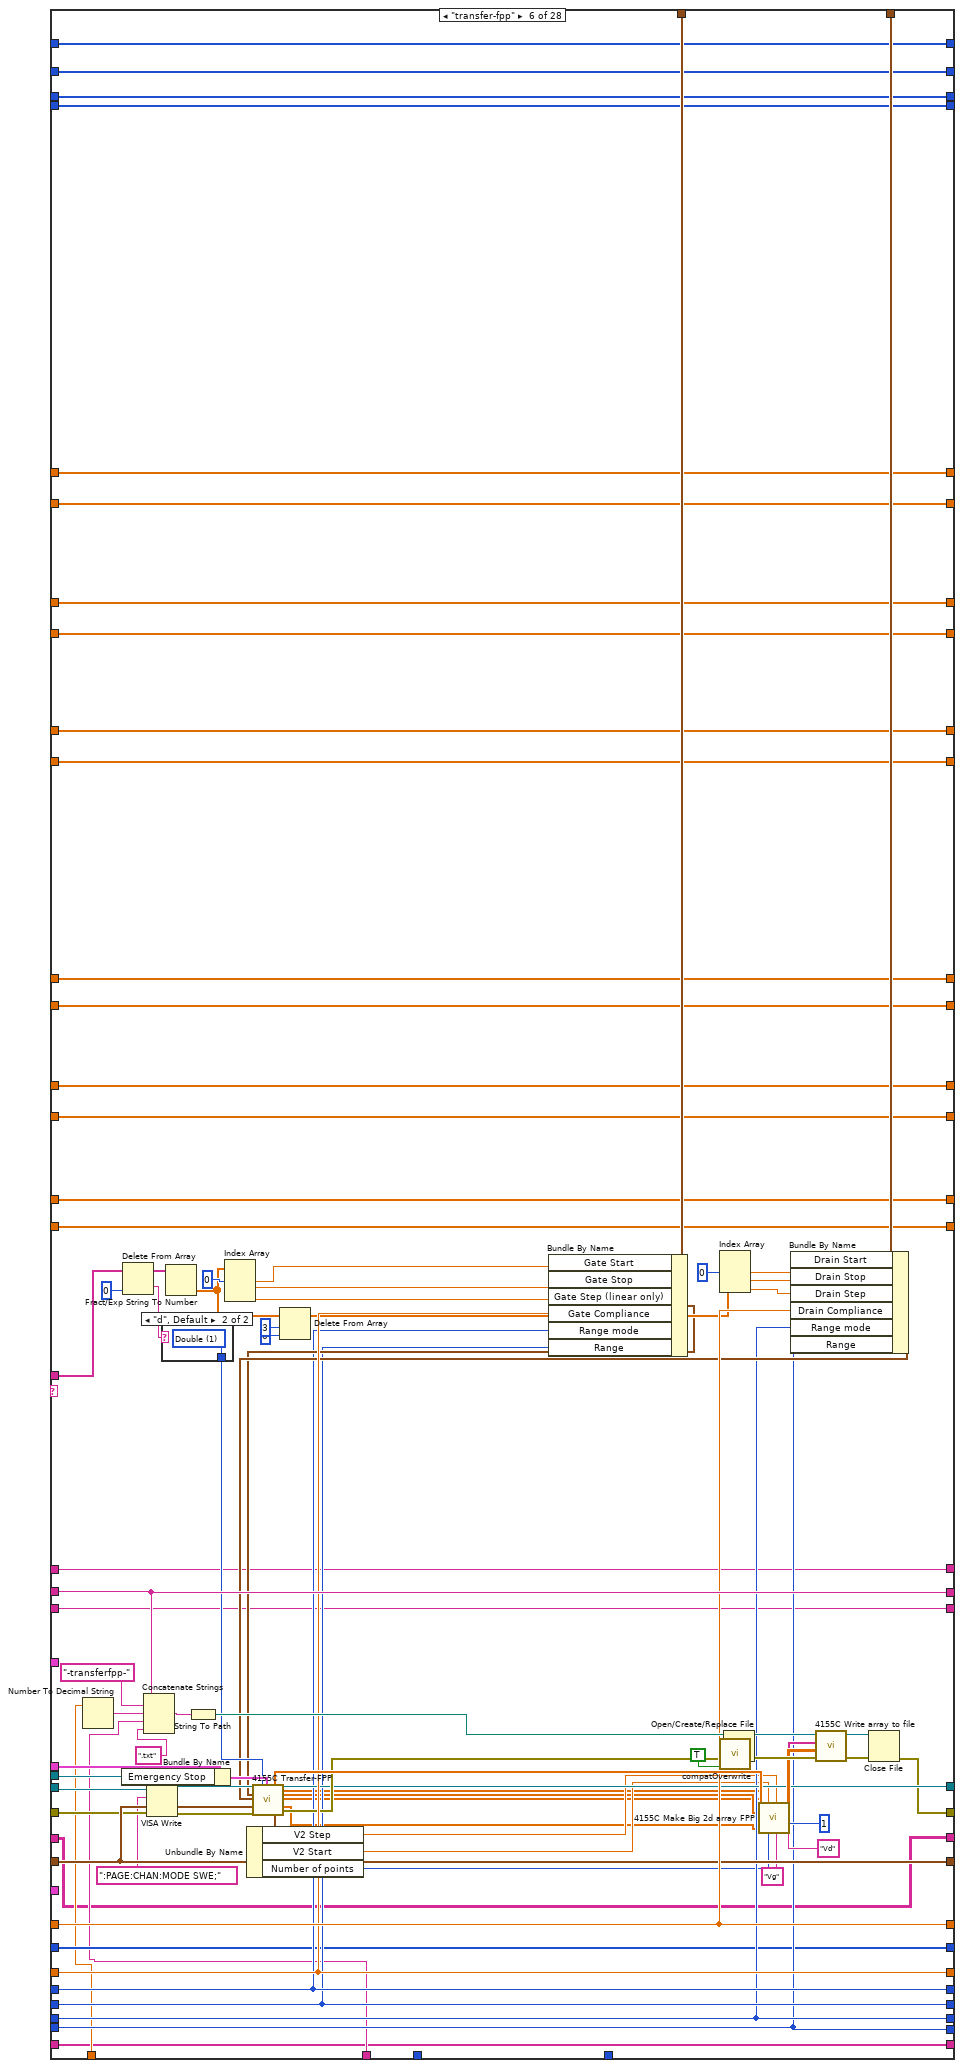
[diagram p14: hidden frame]
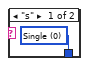
[diagram p15: hidden frame]
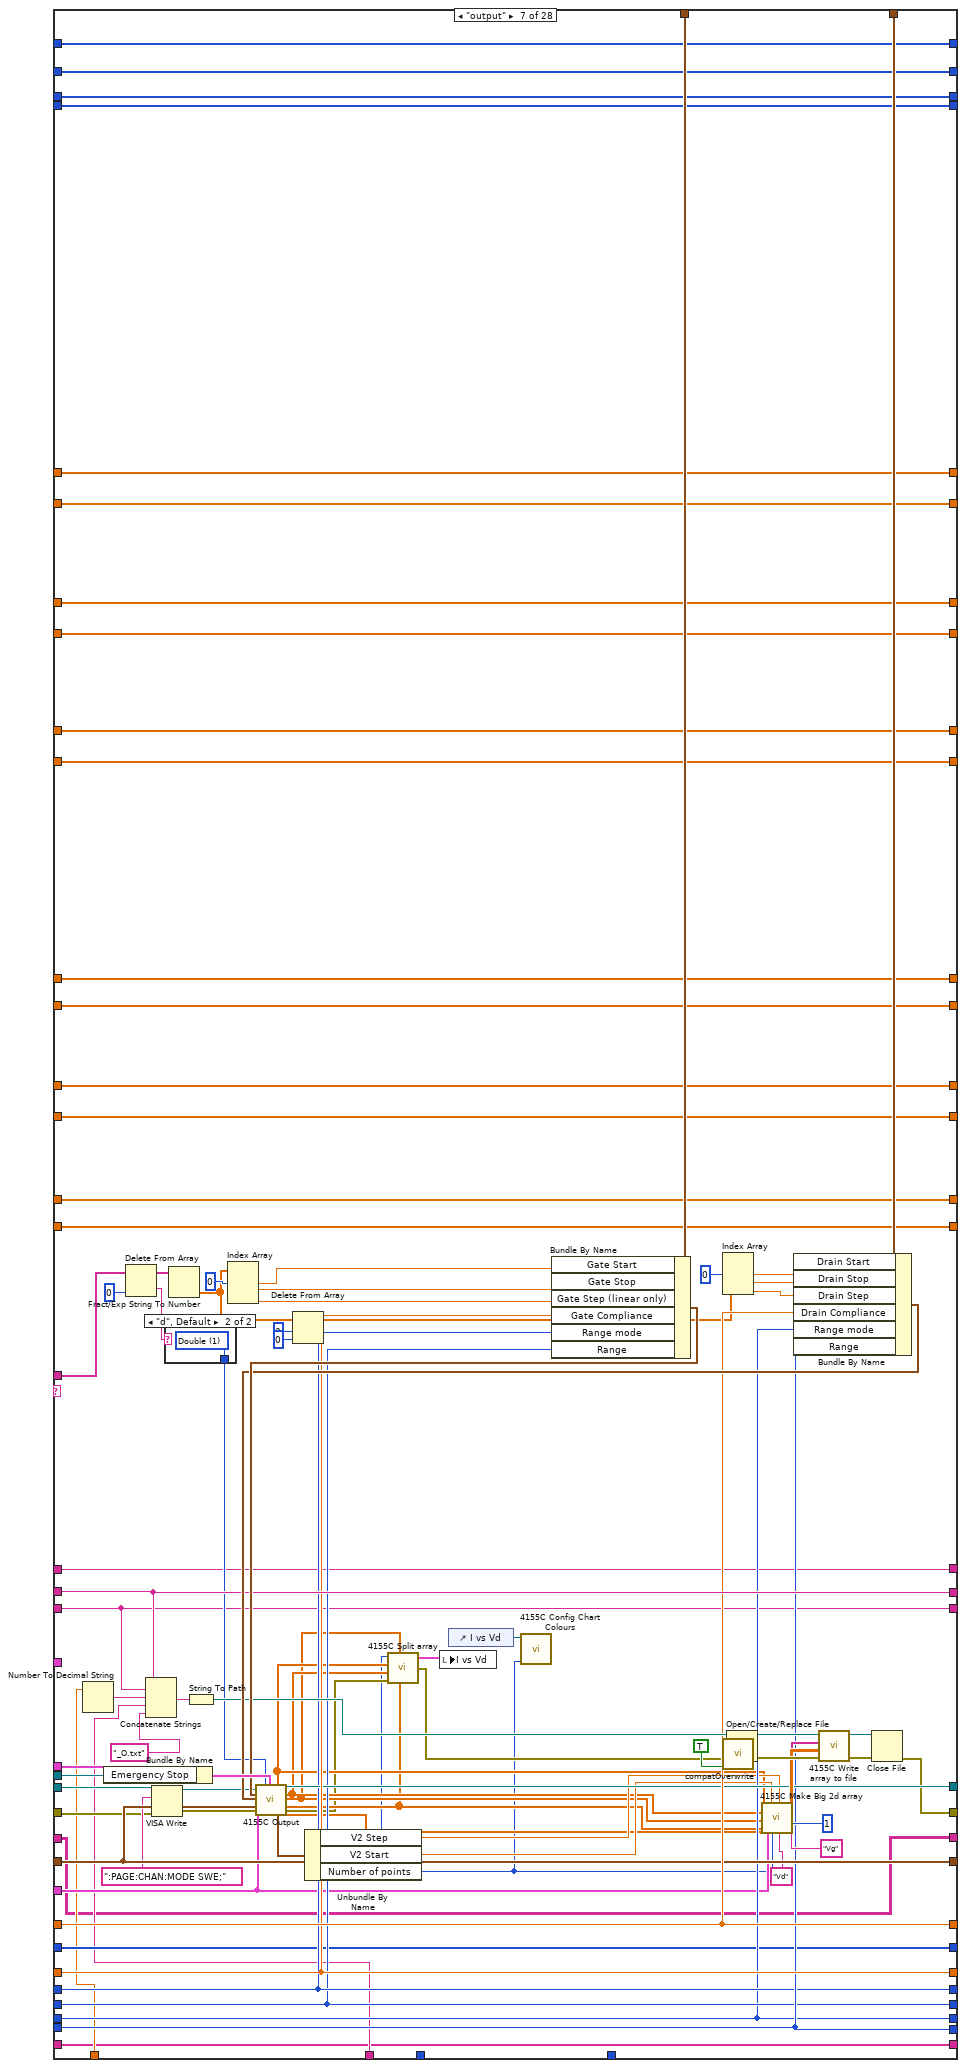
[diagram p16: hidden frame]
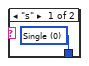
[diagram p17: hidden frame]
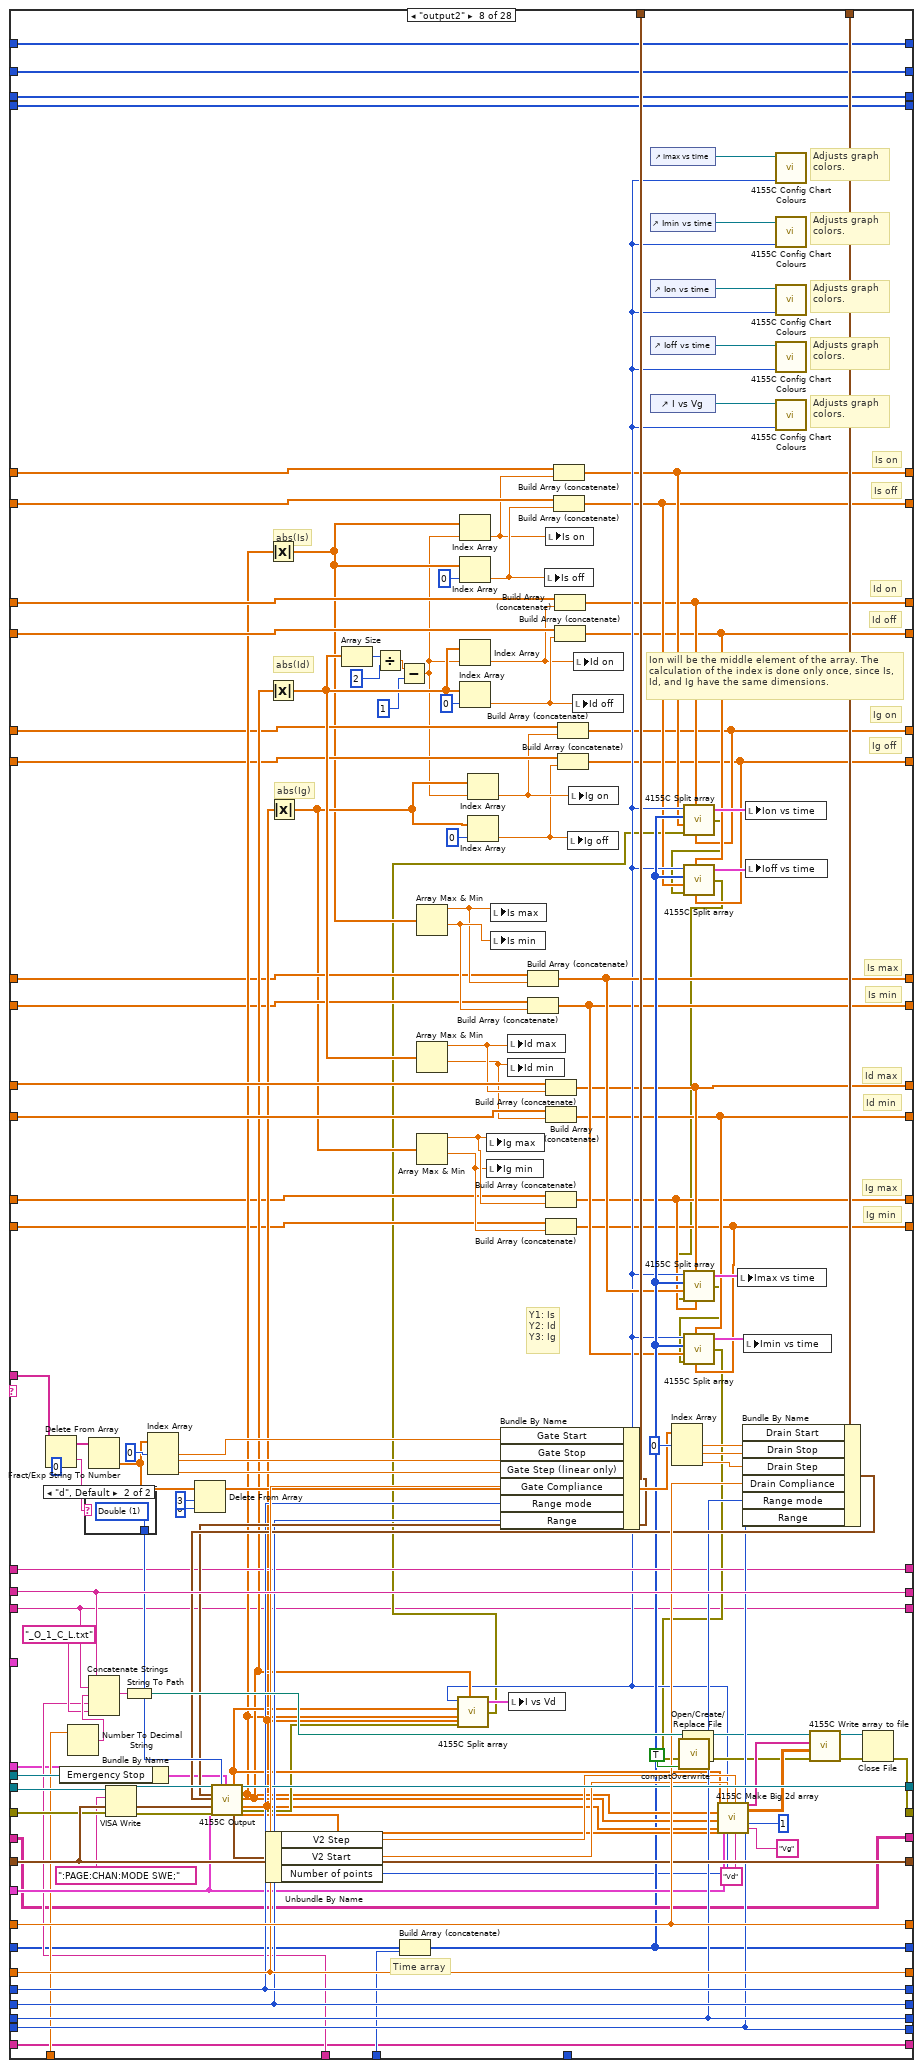
[diagram p18: hidden frame]
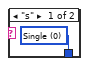
[diagram p19: hidden frame]
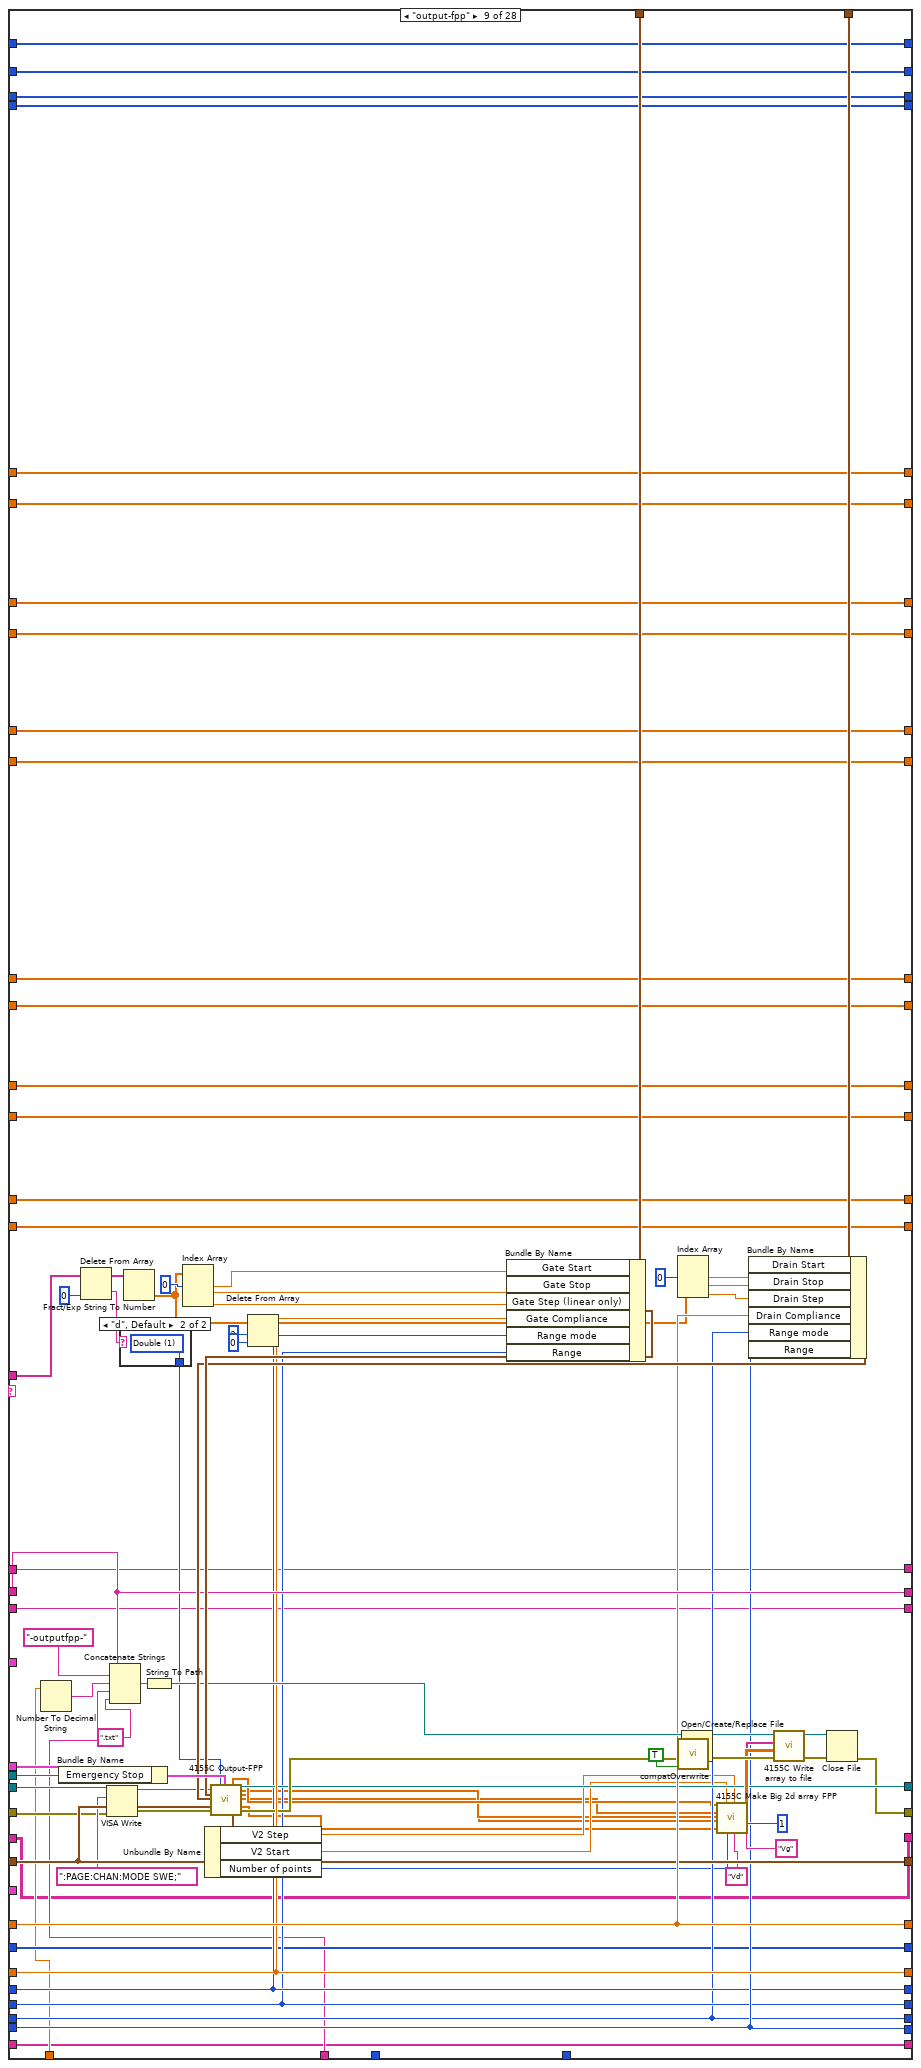
[diagram p20: hidden frame]
diagram:
  w4 = cluster{"Y data in":dbl[], "X data in":dbl[]}[] [] ("I vs Vg")
  w5 = 0.0 ("Is off")
  w6 = 0.0 ("Is on")
  w7 = 0.0 ("Is min")
  w8 = 0.0 ("Is max")
  w59 = u16 1 items=["Reset All", "Partial reset"] ("Type of reset")
  # "Change from previous version:\n\n- Added stop button for the for loop."
  # "This is a version specific to the SPM pump."
  # "I add 1 to both the \"total lines\" and the \"line running\" indicators because i and N begin from 0, and the script lines begin from 1."
  # "Bugs:\n\n- If using the \"filename\" command, keep in mind that the arrays of the time-dependent data are not re-initialized inbetween filename changes. \n\n- Do not connect the \"error\" wire of a Split block if it has unconnected terminals! It will halt the program."
  # "Array size"
  # "%s option converts a spreadsheet string to an array of strings."
  # "0: No of rows of array\n1: No of cols"
  # "Dimitrios Simatos\nv. 6.2"
  # "Changes from original textcontrol.vi:\n\n- Timestamp appears in filename.\n- (Only) transfer and output curves are plotted.\n- Communication with serial port.\n- Can execute any command, as all pattern matching functions were replaced. Previously, commands with special LabVIEW characters could not be executed.\n- Replaced write to file function with write to text file.\n- Replaced while loop with for loop.\n- Replaced 4155C \"Save File\" function and now the vi can save time-dependent variables.\n- Added clock with start time control and various units.\n- Changed filepath in which the program is saved.\n- Added a serial output log that keeps a history.\n- Tab control.\n- Addition of specialized serial read/write file for the SPM OEM pump.\n- Added halt and hard stop.\n- Imax, Imin, Ion, and Ioff are now saved for all Is, Id, and Ig.\n- Output curves are taken into account in Imax-Imin-Ion-Ioff plots (\"output2\" command).\n- Corrected bug of \"itime\" command. The command did not allow for settting the integration time value, it allowed to set the category of the integration time (short, medium, long). If the time value was beyond the range of the category, then the SPA used the closest value allowed, whilst staying in the category. So, if the integration time was changed to long, but the integration time value was a short one, then the SPA would measure using the minimum long integration time value and not the value that the user intended."
  # "Search and replace LF with EOL"
  n1 = Equal?(x="integration time", y=u32 0) -> (x = y?=w60:bool)
  n2 = Select(t="Integration time (short)", s=w60, f="Integration time (long)") -> (s? t:f=w9:dbl)
  n3 = Bundle By Name(cluster="Timings (overwritten by the Front Panel)", "integration time"="integration time", "Short/Long integration time"=w9) -> (w52:T5)
  n4 = call "4155C Get Filename.vi"("error in (no error)"=errorcluster {"status"=FALSE, "code"=0, "source"=""}) -> ("error out"=w54:errorcluster, "path"=w29:path)  [unwired: 2 in, 1 out]
  "Path" <- w29
  n5 = Path To String(path=w29) -> (string=w30:string)
  n6 = Search and Replace String(replace all?=TRUE ("replace all? (F)"), input string="Script", search string="\n", replace string="\r\n") -> (result string=w42:string)  [unwired: 4 in, 3 out]
  n7 = Match Pattern(string=w30, regular expression=".txt") -> (before substring=w25:string)  [unwired: 1 in, 3 out]
  n8 = Concatenate Strings(w25, "Suffix (script)") -> (w24:string)
  n9 = call "4155C Initialise.vi"("VISA resource name in"=refnum<visa-resource-name> "GPIB0::14::INSTR", "Reset"="Full Reset", "Type of reset"=w59, "error in (no error)"=w54, "VISA Timeout Value"=u32 10000) -> ("VISA Resource Name out"=w53:refnum<visa-resource-name>, "error out"=w22:errorcluster)
  n10 = Spreadsheet String To Array(delimiter (Tab)="\r\n", format string="%s", spreadsheet string="Script", array type (2D Dbl)="") -> (array=w33:string[][])
  n11 = Array Size(array=w33) -> (size(s)=w37:i32[])
  n12 = Initialize Array("") -> (w14:string[])  [unwired: 1 in]
  n13 = String To Path(string=w24) -> (path=w23:path)
  n14 = Initialize Array(0 ("element")) -> (w16:i32[])  [unwired: 1 in]
  n15 = Initialize Array("") -> (w12:string[][])  [unwired: 2 in]
  n16 = Initialize Array(0.0 ("element")) -> (w18:dbl[])  [unwired: 1 in]
  n17 = Index Array(array=w37, index=0) -> (element=w35:i32)
  n18 = Write to Text File(file (use dialog)=w23, text=w42, error in=w22) -> (error out=w21:errorcluster)  [unwired: 1 in, 2 out]
  n19 = for {
    N: w35 -> [w175]
    tunnel: "SMU4" -> [w211]
    shift-left: "Source/Drain Range" -> [w216]
    shift-right: [w212] -> _
    shift-left: "Source/Drain\nRange mode" -> [w217]
    shift-right: [w213] -> _
    shift-left: "Gate Range" -> [w218]
    shift-right: [w214] -> _
    shift-left: "Gate Range\nmode" -> [w219]
    shift-right: [w215] -> _
    shift-left: "Gate: Compliance" -> [w228]
    shift-right: [w224] -> _
    shift-left: "Drain: Compliance" -> [w229]
    shift-right: [w225] -> _
    shift-left: w52 -> [w230]
    shift-right: [w226] -> w10
    shift-left: w21 -> [w231]
    shift-right: [w121] -> w28
    shift-left: w53 -> [w232]
    shift-right: [w227] -> _
    shift-left: w25 -> [w233]
    shift-right: [w125] -> _
    tunnel: "Panel Controls 2" -> [w210]
    shift-right: [w83] -> _
    shift-left: w18 -> [w209]
    shift-right: [w145] -> _
    shift-left: i32[] [] -> [w205]
    tunnel: w33 -> [w204] mode=indexing
    shift-right: [w82] -> _
    shift-left: w18 -> [w181]
    shift-right: [w115] -> _
    shift-left: w14 -> [w167]
    shift-right: [w146] -> _
    shift-left: w16 -> [w162]
    shift-right: [w127] -> _
    shift-left: w16 -> [w161]
    shift-right: [w160] -> _
    shift-left: "" -> [w159]
    shift-right: [w120] -> _
    shift-left: w16 -> [w142]
    shift-right: [w119] -> _
    shift-left: w16 -> [w126]
    shift-right: [w116] -> _
    shift-left: w12 -> [w118]
    shift-right: [w76] -> _
    shift-left: w18 -> [w104]
    shift-right: [w77] -> _
    shift-left: w18 -> [w103]
    shift-right: [w81] -> _
    shift-left: w18 -> [w92]
    shift-right: [w80] -> _
    shift-left: w18 -> [w91]
    shift-right: [w74] -> _
    shift-left: w18 -> [w90]
    shift-right: [w84] -> _
    shift-left: w18 -> [w89]
    shift-right: [w75] -> _
    shift-left: w18 -> [w88]
    shift-right: [w73] -> _
    shift-left: w18 -> [w87]
    shift-right: [w79] -> _
    shift-left: w18 -> [w86]
    shift-right: [w78] -> _
    shift-left: w18 -> [w85]
    shift-right: [w68] -> _
    shift-left: "Filename (variable part)" -> [w67]
    i -> [w170]
    stop <- "Interrupt program" stop-if-true
    # "Filename prefix"
    # "Is off"
    # "Is on"
    # "Ig off"
    # "Ig on"
    # "Is min"
    # "Is max"
    # "Ig min"
    # "Ig max"
    # "Id min"
    # "Id max"
    # "Id off"
    # "Id on"
    # "Pump status"
    # "Filepath and name"
    # "Pump status"
    # "Limit of command arguments (array columns). Raise if needed."
    # "Serial port data (string)"
    # "Serial port data (table)"
    # "Time array for valve position"
    # "Time array for absolute plunger position"
    # "Valve position"
    # "Absolute plunger position"
    # "Serial port data"
    # "For loop counter"
    # "<-----Equivalent to the 4155C \"Write\" subvi.----->"
    # "Headers"
    # "Save transfer curves in file."
    # "Filepath and name"
    # "Save time-dependent data."
    # "Use the time offset if your measurements do not start at t=0."
    # "Time for Imax, Imin, Ion, Ioff"
    # "Rest of elements of command"
    # "First element of command\n(case select)"
    n20 = Add(x=w170, y=1) -> (x+y=→"Line running":i32)
    n21 = Add(x=w175, y=1) -> (x+y=→"Total lines":i32)
    n22 = Index Array(array=w204, index=0 ("line index")) -> (element=w199:string)
    "Command running:" <- w199
    n23 = control-ref of="Interrupt scan"() -> (w223:refnum<vi>)
    n24 = Spreadsheet String To Array(delimiter (Tab)=" ", format string="%s", spreadsheet string=w199, array type (2D Dbl)=string[] []) -> (array=w197:string[])
    n25 = Delete From Array(array=w197, index=0) -> (deleted portion=w105:string, array with subset deleted=w196:string[])  [unwired: 1 in]
    n26 = call "Elapsed Time"("Reset"="Reset", "Auto Reset"="Auto Reset") -> ("Elapsed Time (s)"=w206:dbl)  [unwired: 10 in, 7 out]
    n27 = case shown="0, Default" "Time Units" {
      tunnel: ["_sec" "_min" "_h"] -> w207
      tunnel: [w237 w241 w244] -> w177
      tunnel: w206 -> [w237 w240 w245]
      frame 0, Default {
      }
      frame 1 {
        n28 = Divide(x=w240, y=60.0) -> (x/y=w241:dbl)
      }
      frame 2 {
        n29 = Divide(x=w245, y=3600.0) -> (x/y=w244:dbl)
      }
    }
    n30 = Add(x=w177, y="Time Offset") -> (x+y=w176:dbl)
    n31 = To Long Integer(number=w176) -> (32bit integer=w143:i32)
    "Elapsed Time" <- w143
    n32 = case shown="\"serial\"" w105 {
      tunnel: w196 -> [w282 w320 w357 w489 w513 w659 w753 w905 w983 w1010 w1090 w1136 w1180 w1220 w1253 _ _ w1414 w1494 _ w1597 w1660 w1721 w1810 w1891 w1930 w2000 w2054]
      tunnel: w233 -> [w277 w316 w355 w496 w578 w667 w760 w912 w991 w1033 w1079 w1128 w1173 w1214 w1246 w1284 w1345 w1392 w1476 w1526 w1584 w1647 w1709 w1804 w1887 w1932 w2002 w2056]
      tunnel: w232 -> [w276 w315 w346 w467 w563 w636 w729 w883 w959 w1034 w1080 w1129 w1174 w1215 w1247 w1289 w1347 w1420 w1500 w1530 w1603 w1666 w1727 w1816 w1845 w1936 w2006 w2058]
      tunnel: w231 -> [w275 w314 w345 w466 w562 w635 w726 w882 w956 w1035 w1081 w1130 w1175 w1216 w1248 w1288 w1318 w1419 w1499 w1529 w1602 w1665 w1726 w1815 w1844 w1935 w2005 w2059]
      tunnel: w230 -> [w274 w313 w354 w492 w538 w663 w756 w908 w987 w1043 w1089 w1127 w1172 w1213 w1245 w1287 w1342 w1383 w1468 w1535 w1577 w1640 w1702 w1803 w1886 w1937 w2007 w2061]
      tunnel: w229 -> [w273 w312 w353 w494 w576 w665 w758 w910 w989 w1042 w1088 w1135 w1179 w1219 w1252 w1286 w1327 w1418 w1498 w1538 w1601 w1664 w1725 w1814 w1895 w1938 w2008 w2062]
      tunnel: w228 -> [w272 w311 w352 w493 w575 w664 w757 w909 w988 w1041 w1087 w1134 w1178 w1218 w1251 w1285 w1328 w1393 w1477 w1537 w1585 w1648 w1710 w1805 w1888 w1940 w2009 w2064]
      tunnel: [w276 w315 w344 w491 w573 w661 w755 w907 w985 w1034 w1080 w1129 w1174 w1215 w1247 w1289 w1347 w1384 w1450 w1528 w1578 w1641 w1703 w1756 w1847 w1936 w2006 w2058] -> w227
      tunnel: [w275 w314 w343 w490 w572 w660 w754 w906 w984 w1035 w1081 w1130 w1175 w1216 w1248 w1288 w1317 w1394 w1451 w1527 w1586 w1649 w1711 w1755 w1846 w1934 w2004 w2059] -> w141
      tunnel: [w274 w313 w354 w492 w534 w663 w756 w908 w987 w1036 w1082 w1127 w1172 w1213 w1245 w1287 w1342 w1383 w1468 w1535 w1577 w1640 w1702 w1803 w1886 w1937 w2007 w2061] -> w226
      tunnel: [w273 w312 w353 w494 w576 w665 w758 w910 w989 w1042 w1088 w1135 w1179 w1219 w1252 w1286 w1327 w1418 w1498 w1538 w1601 w1664 w1725 w1814 w1895 w1938 w2008 w2062] -> w225
      tunnel: [w272 w311 w352 w493 w575 w664 w757 w909 w988 w1041 w1087 w1134 w1178 w1218 w1251 w1285 w1328 w1393 w1477 w1537 w1585 w1648 w1710 w1805 w1888 w1940 w2009 w2064] -> w224
      tunnel: [w277 w316 w355 w496 w578 w667 w760 w912 w991 w1033 w1079 w1128 w1173 w1214 w1246 w1284 w1345 w1392 w1476 w1526 w1584 w1647 w1709 w1804 w1887 w1932 w2002 w2056] -> w125
      tunnel: w223 -> [_ _ _ w498 w582 w672 w763 w914 w995 _ _ _ _ _ _ _ _ w1389 w1473 _ w1583 w1646 w1708 w1776 w1863 _ _ _]
      tunnel: "Gate" -> [_ _ _ w476 w566 w646 w740 w892 w970 _ _ _ _ _ _ _ _ _ _ _ _ _ _ _ _ _ _ _]
      tunnel: "Drain 2" -> [_ _ _ w475 w565 w645 w739 w891 w969 _ _ _ _ _ _ _ _ _ _ _ _ _ _ _ _ _ _ _]
      tunnel: "Panel Controls" -> [_ _ _ _ _ w644 w738 w776 w968 _ _ _ _ _ _ _ _ _ _ _ _ _ _ _ _ _ _ _]
      tunnel: w219 -> [w271 w310 w351 w460 w556 w629 w724 w876 w954 w1040 w1086 _ w1171 w1212 w1244 w1283 w1329 w1379 w1464 w1531 w1573 w1636 w1698 w1799 w1882 w1941 w2010 w2065]
      tunnel: w218 -> [w270 w309 w350 w459 w555 w628 w723 w875 w953 w1039 w1085 w1133 _ w1203 w1250 w1282 w1330 w1380 w1465 w1532 w1574 w1637 w1699 w1800 w1883 w1942 w2011 w2066]
      tunnel: w217 -> [w269 w308 w349 w458 w554 w627 w722 w874 w952 w1038 w1084 w1132 w1177 w1217 _ w1281 w1331 w1381 w1466 w1533 w1575 w1638 w1700 w1801 w1884 w1943 w2012 w2067]
      tunnel: w216 -> [w268 w307 w348 w457 w553 w626 w725 w873 w955 w1037 w1083 w1131 w1176 _ w1249 w1280 w1332 w1382 w1467 w1534 w1576 w1639 w1701 w1802 w1885 w1944 w2013 w2068]
      tunnel: [w271 w310 w351 w460 w556 w629 w724 w876 w954 w1040 w1086 w1126 w1171 w1212 w1244 w1283 w1329 w1379 w1464 w1531 w1573 w1636 w1698 w1799 w1882 w1941 w2010 w2065] -> w215
      tunnel: [w270 w309 w350 w459 w555 w628 w723 w875 w953 w1039 w1085 w1133 w1163 w1203 w1250 w1282 w1330 w1380 w1465 w1532 w1574 w1637 w1699 w1800 w1883 w1942 w2011 w2066] -> w214
      tunnel: [w269 w308 w349 w458 w554 w627 w722 w874 w952 w1038 w1084 w1132 w1177 w1217 w1243 w1281 w1331 w1381 w1466 w1533 w1575 w1638 w1700 w1801 w1884 w1943 w2012 w2067] -> w213
      tunnel: [w268 w307 w348 w457 w553 w626 w725 w873 w955 w1037 w1083 w1131 w1176 w1204 w1249 w1280 w1332 w1382 w1467 w1534 w1576 w1639 w1701 w1802 w1885 w1944 w2013 w2068] -> w212
      tunnel: w211 -> [_ _ _ w452 w550 _ w718 w868 _ _ _ _ _ _ _ _ _ _ _ _ _ _ _ _ _ _ _ _]
      tunnel: w210 -> [_ _ _ w450 w549 _ _ _ _ _ _ _ _ _ _ _ _ _ _ _ _ _ _ _ _ _ _ _]
      tunnel: [w267 w303 w341 w378 w526 w616 w715 w795 w941 w1032 w1077 w1125 w1162 w1202 w1242 w1279 w1313 w1371 w1429 w1525 w1562 w1629 w1692 w1753 w1840 w1933 w2003 w2073] -> w83
      tunnel: w209 -> [w267 w303 w341 w447 w526 w616 w715 w864 w941 w1032 w1077 w1125 w1162 w1202 w1242 w1279 w1313 w1371 w1429 w1525 w1562 w1629 w1692 w1753 w1840 w1933 w2003 w2073]
      tunnel: w176 -> [_ _ _ w444 w523 w614 w712 w861 w938 _ _ _ _ _ _ _ w1311 w1369 w1446 _ w1559 w1626 w1689 w1750 w1836 _ _ _]
      tunnel: w207 -> [_ _ _ w441 w522 w612 w711 w858 w937 _ _ _ _ _ _ _ w1309 w1367 w1445 _ w1558 w1625 w1688 w1749 w1837 _ w1971 _]
      tunnel: w143 -> [_ _ _ w436 _ _ _ w853 _ _ _ _ _ _ _ _ _ _ _ _ _ _ _ _ _ _ w1974 _]
      tunnel: [w266 w302 w340 w386 w525 w615 w714 w803 w940 w1031 w1076 w1124 w1161 w1201 w1241 w1278 w1312 w1370 w1448 w1524 w1561 w1628 w1691 w1752 w1839 w1939 w1983 w2063] -> w145
      tunnel: w205 -> [w266 w302 w340 w440 w525 w615 w714 w857 w940 w1031 w1076 w1124 w1161 w1201 w1241 w1278 w1312 w1370 w1448 w1524 w1561 w1628 w1691 w1752 w1839 w1939 w1983 w2063]
      tunnel: [w265 w301 w339 w377 w521 w611 w710 w794 w936 w1030 w1075 w1123 w1160 w1200 w1240 w1277 w1308 w1366 w1428 w1523 w1557 w1624 w1687 w1748 w1835 w1928 w1999 w2072] -> w82
      tunnel: w181 -> [w265 w301 w339 w434 w521 w611 w710 w851 w936 w1030 w1075 w1123 w1160 w1200 w1240 w1277 w1308 w1366 w1428 w1523 w1557 w1624 w1687 w1748 w1835 w1928 w1999 w2072]
      tunnel: [w264 w300 w338 w427 w520 w610 w700 w844 w935 w1029 w1074 w1122 w1159 w1199 w1239 w1276 w1307 w1365 w1444 w1522 w1556 w1623 w1686 w1747 w1834 w1927 w1998 w2069] -> w115
      tunnel: w167 -> [w264 w300 w338 w427 w520 w610 w700 w844 w935 w1029 w1074 w1122 w1159 w1199 w1239 w1276 w1307 w1365 w1444 w1522 w1556 w1623 w1686 w1747 w1834 w1926 w1972 w2069]
      tunnel: [w263 w299 w337 w426 w519 w609 w699 w843 w934 w1028 w1073 w1121 w1158 w1198 w1238 w1275 w1306 w1364 w1443 w1521 w1555 w1622 w1685 w1746 w1833 w1912 w1985 w2083] -> w146
      tunnel: w162 -> [w263 w299 w337 w426 w519 w609 w699 w843 w934 w1028 w1073 w1121 w1158 w1198 w1238 w1275 w1306 w1364 w1443 w1521 w1555 w1622 w1685 w1746 w1833 w1912 w1984 w2083]
      tunnel: [w262 w298 w336 w425 w518 w608 w698 w842 w933 w1027 w1072 w1120 w1157 w1197 w1237 w1274 w1305 w1363 w1442 w1520 w1554 w1621 w1684 w1745 w1832 w1911 w1967 w2085] -> w127
      tunnel: w161 -> [w262 w298 w336 w425 w518 w608 w698 w842 w933 w1027 w1072 w1120 w1157 w1197 w1237 w1274 w1305 w1363 w1442 w1520 w1554 w1621 w1684 w1745 w1832 w1911 w1965 w2085]
      tunnel: [w261 w297 w335 w424 w517 w607 w697 w841 w932 w1026 w1071 w1119 w1156 w1196 w1236 w1273 w1304 w1362 w1441 w1519 w1553 w1620 w1683 w1744 w1831 w1910 w1964 w2057] -> w160
      tunnel: w159 -> [w261 w297 w335 w424 w517 w607 w697 w841 w932 w1026 w1071 w1119 w1156 w1196 w1236 w1273 w1304 w1362 w1441 w1519 w1553 w1620 w1683 w1744 w1831 w1910 w1975 w2057]
      tunnel: w143 -> [_ _ _ _ _ _ _ _ _ _ _ _ _ _ _ _ _ _ _ _ _ _ _ _ _ _ w1963 _]
      tunnel: w142 -> [w260 w296 w334 w423 w516 w606 w696 w840 w931 w1025 w1070 w1118 w1155 w1195 w1235 w1272 w1303 w1361 w1440 w1518 w1552 w1619 w1682 w1743 w1830 w1909 w1962 w2084]
      tunnel: [w260 w296 w334 w423 w516 w606 w696 w840 w931 w1025 w1070 w1118 w1155 w1195 w1235 w1272 w1303 w1361 w1440 w1518 w1552 w1619 w1682 w1743 w1830 w1909 w1961 w2084] -> w120
      tunnel: [w259 w295 w333 w422 w515 w605 w695 w839 w930 w1024 w1069 w1117 w1154 w1194 w1234 w1271 w1302 w1360 w1439 w1517 w1551 w1618 w1681 w1742 w1829 w1908 w1960 w2082] -> w119
      tunnel: w126 -> [w259 w295 w333 w422 w515 w605 w695 w839 w930 w1024 w1069 w1117 w1154 w1194 w1234 w1271 w1302 w1360 w1439 w1517 w1551 w1618 w1681 w1742 w1829 w1908 w1959 w2082]
      tunnel: [w258 w294 w332 w421 w514 w604 w694 w838 w929 w1023 w1068 w1116 w1153 w1193 w1233 w1270 w1301 w1359 w1438 w1516 w1550 w1617 w1680 w1741 w1828 w1907 w1957 w2060] -> w116
      tunnel: w118 -> [w258 w294 w332 w421 w514 w604 w694 w838 w929 w1023 w1068 w1116 w1153 w1193 w1233 w1270 w1301 w1359 w1438 w1516 w1550 w1617 w1680 w1741 w1828 w1907 w1956 w2060]
      tunnel: [w256 w292 w330 w371 w511 w602 w692 w788 w927 w1021 w1067 w1115 w1151 w1191 w1231 w1268 w1299 w1358 w1437 w1515 w1549 w1616 w1678 w1740 w1827 w1906 w1955 w2078] -> w76
      tunnel: w104 -> [w256 w292 w330 w417 w511 w602 w692 w834 w927 w1021 w1067 w1115 w1151 w1191 w1231 w1268 w1299 w1358 w1437 w1515 w1549 w1616 w1678 w1740 w1827 w1906 w1955 w2078]
      tunnel: [w257 w293 w331 w372 w512 w603 w693 w789 w928 w1022 w1066 w1114 w1152 w1192 w1232 w1269 w1300 w1357 w1436 w1514 w1548 w1615 w1679 w1739 w1826 w1905 w1954 w2079] -> w77
      tunnel: w103 -> [w257 w293 w331 w416 w512 w603 w693 w833 w928 w1022 w1066 w1114 w1152 w1192 w1232 w1269 w1300 w1357 w1436 w1514 w1548 w1615 w1679 w1739 w1826 w1905 w1954 w2079]
      tunnel: [w249 w285 w323 w376 w508 w600 w690 w793 w925 w1014 w1064 w1112 w1149 w1189 w1229 w1266 w1292 w1350 w1427 w1513 w1541 w1608 w1671 w1732 w1821 w1898 w1953 w2071] -> w81
      tunnel: w92 -> [w249 w285 w323 w406 w508 w600 w690 w823 w925 w1014 w1064 w1112 w1149 w1189 w1229 w1266 w1292 w1350 w1427 w1513 w1541 w1608 w1671 w1732 w1821 w1898 w1953 w2071]
      tunnel: [w248 w284 w322 w375 w509 w601 w691 w792 w926 w1013 w1065 w1113 w1150 w1190 w1230 w1267 w1291 w1349 w1426 w1512 w1540 w1607 w1670 w1731 w1820 w1897 w1952 w2070] -> w80
      tunnel: w91 -> [w248 w284 w322 w405 w509 w601 w691 w822 w926 w1013 w1065 w1113 w1150 w1190 w1230 w1267 w1291 w1349 w1426 w1512 w1540 w1607 w1670 w1731 w1820 w1897 w1952 w2070]
      tunnel: [w251 w287 w325 w381 w507 w598 w688 w798 w923 w1019 w1062 w1110 w1147 w1187 w1227 w1264 w1294 w1352 w1431 w1507 w1543 w1610 w1673 w1734 w1819 w1902 w1950 w2075] -> w74
      tunnel: w90 -> [w251 w287 w325 w402 w507 w598 w688 w819 w923 w1019 w1062 w1110 w1147 w1187 w1227 w1264 w1294 w1352 w1431 w1507 w1543 w1610 w1673 w1734 w1819 w1902 w1950 w2075]
      tunnel: [w250 w286 w324 w379 w510 w599 w689 w796 w924 w1020 w1063 w1111 w1148 w1188 w1228 w1265 w1293 w1351 w1430 w1506 w1542 w1609 w1672 w1733 w1818 w1901 w1951 w2074] -> w84
      tunnel: w89 -> [w250 w286 w324 w401 w510 w599 w689 w818 w924 w1020 w1063 w1111 w1148 w1188 w1228 w1265 w1293 w1351 w1430 w1506 w1542 w1609 w1672 w1733 w1818 w1901 w1951 w2074]
      tunnel: [w253 w289 w327 w370 w506 w596 w686 w787 w921 w1017 w1060 w1108 w1145 w1185 w1225 w1262 w1296 w1354 w1433 w1509 w1545 w1612 w1675 w1736 w1823 w1904 w1948 w2077] -> w75
      tunnel: w88 -> [w253 w289 w327 w398 w506 w596 w686 w815 w921 w1017 w1060 w1108 w1145 w1185 w1225 w1262 w1296 w1354 w1433 w1509 w1545 w1612 w1675 w1736 w1823 w1904 w1948 w2077]
      tunnel: [w252 w288 w326 w369 w505 w597 w687 w786 w922 w1018 w1061 w1109 w1146 w1186 w1226 w1263 w1295 w1353 w1432 w1508 w1544 w1611 w1674 w1735 w1822 w1903 w1949 w2076] -> w73
      tunnel: w87 -> [w252 w288 w326 w397 w505 w597 w687 w814 w922 w1018 w1061 w1109 w1146 w1186 w1226 w1263 w1295 w1353 w1432 w1508 w1544 w1611 w1674 w1735 w1822 w1903 w1949 w2076]
      tunnel: [w255 w291 w329 w374 w504 w594 w684 w791 w919 w1015 w1058 w1106 w1143 w1183 w1223 w1260 w1298 w1356 w1435 w1511 w1547 w1614 w1677 w1738 w1825 w1900 w1946 w2081] -> w79
      tunnel: w86 -> [w255 w291 w329 w394 w504 w594 w684 w811 w919 w1015 w1058 w1106 w1143 w1183 w1223 w1260 w1298 w1356 w1435 w1511 w1547 w1614 w1677 w1738 w1825 w1900 w1946 w2081]
      tunnel: [w254 w290 w328 w373 w503 w595 w685 w790 w920 w1016 w1059 w1107 w1144 w1184 w1224 w1261 w1297 w1355 w1434 w1510 w1546 w1613 w1676 w1737 w1824 w1899 w1947 w2080] -> w78
      tunnel: w85 -> [w254 w290 w328 w393 w503 w595 w685 w810 w920 w1016 w1059 w1107 w1144 w1184 w1224 w1261 w1297 w1355 w1434 w1510 w1546 w1613 w1676 w1737 w1824 w1899 w1947 w2080]
      tunnel: w67 -> [w247 w283 w321 w360 w502 w593 w683 w777 w918 w1012 w1057 w1105 w1142 w1182 w1222 w1259 w1290 w1348 w1425 w1505 w1539 w1606 w1669 w1730 w1817 w1896 w1945 _]
      tunnel: [w247 w283 w321 w360 w502 w593 w683 w777 w918 w1012 w1057 w1105 w1142 w1182 w1222 w1259 w1290 w1348 w1425 w1505 w1539 w1606 w1669 w1730 w1817 w1896 w1945 w2053] -> w68
      frame "wait" {
        n33 = Index Array(array=w282, index=0 ("Index")) -> (element=w280:string)
        n34 = Decimal String To Number(string=w280, default (0L)=u32 0) -> (number=w279:u32)  [unwired: 1 in, 1 out]
        n35 = Wait (ms)(milliseconds to wait=w279) -> ()  [unwired: 1 out]
      }
      frame "wait-min" {
        n36 = Index Array(array=w320, index=0 ("Index")) -> (element=w318:string)
        n37 = Decimal String To Number(string=w318, default (0L)=u32 0) -> (number=w306:u32)  [unwired: 1 in, 1 out]
        n38 = Multiply(x=w306, y=u32 60000) -> (x*y=w305:u32)
        n39 = Wait (ms)(milliseconds to wait=w305) -> ()  [unwired: 1 out]
      }
      frame "standby" {
        n40 = Index Array(array=w357, index=0 ("Index")) -> (element=w347:string)
        n41 = case shown="\"off\", Default" w347 {
          tunnel: [":PAGE:SCON:STAN 0" ":PAGE:SCON:STAN 1"] -> w342
          frame "off", Default {
          }
          frame "on" {
          }
        }
        n42 = VISA Write(VISA resource name=w346, write buffer=w342, error in (no error)=w345) -> (VISA resource name out=w344:refnum<visa-resource-name>, error out=w343:errorcluster)  [unwired: 1 out]
      }
      frame "transfer" {
        # "Adjusts graph colors."
        # "Adjusts graph colors."
        # "Is off"
        # "Is on"
        # "Ion will be the middle element of the array. The calculation of the index is done only once, since Is, Id, and Ig have the same dimensions."
        # "Ig off"
        # "Ig on"
        # "Is min"
        # "Is max"
        # "Ig min"
        # "Ig max"
        # "abs(Ig)"
        # "abs(Is)"
        # "Id min"
        # "Id max"
        # "Y1: Is\nY2: Id\nY3: Ig"
        # "abs(Id)"
        # "Adjusts graph colors."
        # "Adjusts graph colors."
        # "Id off"
        # "Id on"
        # "Adjusts graph colors."
        # "Time array"
        n43 = Delete From Array(array=w489, index=0 ("Index")) -> (deleted portion=w487:string, array with subset deleted=w486:string[])  [unwired: 1 in]
        n44 = Bundle By Name(cluster=w450, "Emergency Stop"=w498) -> (w451:T2)
        n45 = Number To Decimal String(number=w444) -> (decimal integer string=w443:string)  [unwired: 1 in]
        n46 = case shown="\"d\", Default" w487 {
          tunnel: [w500 w501] -> w485
          frame "s" {
            w500 = u16 0 items=["Single", "Double"] ("sweep mode")
          }
          frame "d", Default {
            w501 = u16 1 items=["Single", "Double"] ("sweep mode")
          }
        }
        n47 = Fract/Exp String To Number(string=w486) -> (number=w471:dbl[])  [unwired: 3 in, 1 out]
        n48 = Concatenate Strings(w496, w360, w443, w441, "_T_1_C_L.txt" ("Suffix (transfer)")) -> (w497:string)
        n49 = VISA Write(VISA resource name=w467, write buffer=":PAGE:CHAN:MODE SWE;" ("write buffer (\"\")"), error in (no error)=w466) -> (VISA resource name out=w464:refnum<visa-resource-name>, error out=w465:errorcluster)  [unwired: 1 out]
        n50 = String To Path(string=w497) -> (path=w495:path)
        n51 = Index Array(array=w471, index #1=0 ("Index")) -> (element #1=w484:dbl, element #2=w483:dbl, element #3=w482:dbl)  [unwired: 2 in]
        n52 = Delete From Array(array=w471, length=3 ("Length"), index=0 ("Index")) -> (array with subset deleted=w469:dbl[])  [unwired: 1 out]
        n53 = Build Array (concatenate)(w440, w436) -> (w386:i32[])
        n54 = Bundle By Name(cluster=w476, "Gate Start"=w484, "Gate Stop"=w483, "Gate Step (linear only)"=w482, "Gate Compliance"=w493, "Range mode"=w460, "Range"=w459) -> (w461:T6)
        n55 = control-ref of="Imax vs time"() -> (w415:refnum<vi>)
        n56 = control-ref of="Imin vs time"() -> (w414:refnum<vi>)
        n57 = control-ref of="Ion vs time"() -> (w383:refnum<vi>)
        n58 = control-ref of="Ioff vs time"() -> (w382:refnum<vi>)
        n59 = control-ref of="I vs Vg"() -> (w445:refnum<vi>)
        n60 = Index Array(array=w469, index #1=0 ("Index")) -> (element #1=w479:dbl, element #2=w478:dbl, element #3=w477:dbl)  [unwired: 2 in]
        n61 = call <vilib>:"compatOverwrite.vi"("overwrite (F)"=TRUE) -> ("overwrite?"=w449:T8)
        n62 = Bundle By Name(cluster=w475, "Drain Start"=w479, "Drain Stop"=w478, "Drain Step"=w477, "Drain Compliance"=w494, "Range mode"=w458, "Range"=w457) -> (w462:T7)
        n63 = call "4155C Transfer.vi"("VISA resource name in"=w464, "Gate"=w461, "Drain"=w462, "Timings"=w492, "error in (no error)"=w465, "SMU4"=w452, "sweep mode"=w485, "Panel Controls"=w451) -> ("VG"=w448:dbl[], "Outparams"=w456:T9, "VISA Resource Name out"=w491:refnum<visa-resource-name>, "IS"=w411:dbl[], "ID"=w413:dbl[], "IG"=w410:dbl[], "error out"=w437:errorcluster, "SMU4"=w453:dbl[])  [unwired: 12 in]
        n64 = Unbundle By Name(w456) -> ("V2 Step"=w455:dbl, "V2 Start"=w454:dbl, "Number of points"=w380:i32)
        n65 = Absolute Value(x=w411) -> (abs(x)=w396:dbl[])
        n66 = Absolute Value(x=w413) -> (abs(x)=w412:dbl[])
        n67 = Absolute Value(x=w410) -> (abs(x)=w399:dbl[])
        n68 = Array Size(array=w412) -> (size(s)=w420:i32)
        n69 = Divide(x=w420, y=2) -> (x/y=w363:dbl)
        n70 = Subtract(x=w363, y=1) -> (x-y=w362:dbl)
        n71 = Array Max & Min(array=w396) -> (max value=w403:dbl, min value=w404:dbl)  [unwired: 2 out]
        n72 = Array Max & Min(array=w412) -> (max value=w446:dbl, min value=w409:dbl)  [unwired: 2 out]
        n73 = Array Max & Min(array=w399) -> (max value=w408:dbl, min value=w407:dbl)  [unwired: 2 out]
        n74 = call "4155C Split array.vi"("Number of VAR2 steps"=w380, "Y2 data in"=w413, "X data in"=w448, "Y1 data in"=w411, "Y3 data in"=w410, "error in (no error)"=w437) -> ("Array of clusters"=w439:cluster{"Y data in":dbl[], "X data in":dbl[]}[], "error out"=w368:errorcluster)  [unwired: 1 in]
        n75 = Index Array(array=w396, index=w362) -> (element=w387:dbl)
        n76 = Index Array(array=w396, index=0) -> (element=w388:dbl)
        n77 = Index Array(array=w412, index=w362) -> (element=w389:dbl)
        n78 = Index Array(array=w412, index=0) -> (element=w390:dbl)
        n79 = Index Array(array=w399, index=w362) -> (element=w392:dbl)
        n80 = Index Array(array=w399, index=0) -> (element=w391:dbl)
        n81 = local write "Ig max"(w408) -> ()
        n82 = local write "Ig min"(w407) -> ()
        n83 = local write "Is max"(w403) -> ()
        n84 = local write "Is min"(w404) -> ()
        n85 = local write "Id max"(w446) -> ()
        n86 = local write "Id min"(w409) -> ()
        n87 = local write "I vs Vg"(w439) -> ()
        n88 = Build Array (concatenate)(w402, w403) -> (w381:dbl[])
        n89 = Build Array (concatenate)(w401, w404) -> (w379:dbl[])
        n90 = local write "Is off"(w388) -> ()
        n91 = local write "Is on"(w387) -> ()
        n92 = Build Array (concatenate)(w447, w446) -> (w378:dbl[])
        n93 = Build Array (concatenate)(w434, w409) -> (w377:dbl[])
        n94 = Build Array (concatenate)(w406, w408) -> (w376:dbl[])
        n95 = Build Array (concatenate)(w405, w407) -> (w375:dbl[])
        n96 = Build Array (concatenate)(w394, w387) -> (w374:dbl[])
        n97 = Build Array (concatenate)(w393, w388) -> (w373:dbl[])
        n98 = Build Array (concatenate)(w416, w389) -> (w372:dbl[])
        n99 = Build Array (concatenate)(w417, w390) -> (w371:dbl[])
        n100 = Build Array (concatenate)(w398, w392) -> (w370:dbl[])
        n101 = Build Array (concatenate)(w397, w391) -> (w369:dbl[])
        n102 = local write "Ig off"(w391) -> ()
        n103 = local write "Ig on"(w392) -> ()
        n104 = local write "Id off"(w390) -> ()
        n105 = local write "Id on"(w389) -> ()
        n106 = call "4155C Split array.vi"("Number of VAR2 steps"=w380, "Y2 data in"=w372, "X data in"=w386, "Y1 data in"=w374, "Y3 data in"=w370, "error in (no error)"=w368) -> ("Array of clusters"=w384:cluster{"Y data in":dbl[], "X data in":dbl[]}[], "error out"=w367:errorcluster)  [unwired: 1 in]
        n107 = call "4155C Split array.vi"("Number of VAR2 steps"=w380, "Y2 data in"=w371, "X data in"=w386, "Y1 data in"=w373, "Y3 data in"=w369, "error in (no error)"=w367) -> ("Array of clusters"=w385:cluster{"Y data in":dbl[], "X data in":dbl[]}[], "error out"=w366:errorcluster)  [unwired: 1 in]
        n108 = call "4155C Split array.vi"("Number of VAR2 steps"=w380, "Y2 data in"=w378, "X data in"=w386, "Y1 data in"=w381, "Y3 data in"=w376, "error in (no error)"=w366) -> ("Array of clusters"=w438:cluster{"Y data in":dbl[], "X data in":dbl[]}[], "error out"=w365:errorcluster)  [unwired: 1 in]
        n109 = call "4155C Split array.vi"("Number of VAR2 steps"=w380, "Y2 data in"=w377, "X data in"=w386, "Y1 data in"=w379, "Y3 data in"=w375, "error in (no error)"=w365) -> ("Array of clusters"=w435:cluster{"Y data in":dbl[], "X data in":dbl[]}[], "error out"=w364:errorcluster)  [unwired: 1 in]
        n110 = Open/Create/Replace File(file path (use dialog)=w495, error in=w364, operation (0:open)=w449) -> (refnum out=w432:refnum<file>, error out=w430:errorcluster)  [unwired: 3 in, 1 out]
        n111 = call "4155C Make Big 2d array.vi"("1D Var1"=w448, "1d IS"=w411, "1d ID"=w413, "1d IG"=w410, "1d SMU4"=w453, "SMU4"=w452, "VAR2 START"=w454, "Number of VAR2 steps"=w380, "VAR2 STEP"=w455, "VAR1 Name"="Vg", "Decimal places in header"=i8 1, "VAR2 Name"="Vd") -> ("Header array"=w433:string[], "Data array"=w431:dbl[][])  [unwired: 14 in]
        n112 = local write "Imax vs time"(w438) -> ()
        n113 = local write "Imin vs time"(w435) -> ()
        n114 = local write "Ion vs time"(w384) -> ()
        n115 = local write "Ioff vs time"(w385) -> ()
        n116 = call "4155C Config Chart Colours.vi"("Numeric"=w380, "XY Graph 2"=w415) -> ()  [unwired: 6 in]
        n117 = call "4155C Config Chart Colours.vi"("Numeric"=w380, "XY Graph 2"=w414) -> ()  [unwired: 6 in]
        n118 = call "4155C Config Chart Colours.vi"("Numeric"=w380, "XY Graph 2"=w383) -> ()  [unwired: 6 in]
        n119 = call "4155C Config Chart Colours.vi"("Numeric"=w380, "XY Graph 2"=w382) -> ()  [unwired: 6 in]
        n120 = call "4155C Config Chart Colours.vi"("Numeric"=w380, "XY Graph 2"=w445) -> ()  [unwired: 6 in]
        n121 = call "4155C Write array to file.vi"("Byte Stream File Refnum"=w432, "Header"=w433, "Data Array"=w431, "error in (no error)"=w430) -> ("dup refnum"=w429:refnum<file>, "error out"=w428:errorcluster)  [unwired: 1 in]
        n122 = Close File(refnum=w429, error in=w428) -> (error out=w490:errorcluster)  [unwired: 1 out]
      }
      frame "pulsedstressV" {
        w532 = 0
        n123 = Number To Decimal String(number=w523) -> (decimal integer string=w579:string)  [unwired: 1 in]
        n124 = Delete From Array(array=w513, index=0 ("Index")) -> (deleted portion=w570:string, array with subset deleted=w569:string[])  [unwired: 1 in]
        n125 = Bundle By Name(cluster=w549, "Emergency Stop"=w582) -> (w551:T2)
        n126 = VISA Write(VISA resource name=w563, write buffer=":PAGE:CHAN:MODE SWE;" ("write buffer (\"\")"), error in (no error)=w562) -> (VISA resource name out=w560:refnum<visa-resource-name>, error out=w561:errorcluster)  [unwired: 1 out]
        n127 = Concatenate Strings(w578, "-pulsedstressV-" ("Substring"), w579, w522, ".txt" ("Substring")) -> (w581:string)
        n128 = case shown="\"d\", Default" w570 {
          tunnel: [w591 w592] -> w568
          frame "s" {
            w591 = u16 0 items=["Single", "Double"] ("sweep mode")
          }
          frame "d", Default {
            w592 = u16 1 items=["Single", "Double"] ("sweep mode")
          }
        }
        n129 = Fract/Exp String To Number(string=w569) -> (number=w564:dbl[])  [unwired: 3 in, 1 out]
        n130 = String To Path(string=w581) -> (path=w577:path)
        n131 = Index Array(array=w564, index #1=0 ("Index")) -> (element #1=w541:dbl, element #2=w540:dbl, element #3=w537:dbl, element #4=w536:dbl, element #5=w535:dbl, element #6=w539:dbl)  [unwired: 5 in]
        n132 = Bundle By Name(cluster=w538, "Pulse period"=w536, "Base voltage"=w537, "Pulse width"=w535) -> (w534:T5)
        n133 = Unbundle By Name(w534) -> ("Pulse period"=w542:dbl)
        n134 = Bundle By Name(cluster=w566, "Gate Start"=w540, "Gate Stop"=w541, "Gate Step (linear only)"=0, "Gate Compliance"=w575, "Range mode"=w556, "Range"=w555) -> (w557:T6)
        n135 = call <vilib>:"compatOverwrite.vi"("overwrite (F)"=TRUE) -> ("overwrite?"=w527:T8)
        n136 = Bundle By Name(cluster=w565, "Drain Start"=w539, "Drain Stop"=w532, "Drain Step"=w532, "Drain Compliance"=w576, "Range mode"=w554, "Range"=w553) -> (w558:T7)
        n137 = call "4155C PulsedStressV.vi"("VISA resource name in"=w560, "sweep mode"=w568, "Panel Controls"=w551, "Gate"=w557, "Drain"=w558, "Timings"=w534, "error in (no error)"=w561, "SMU4"=w550) -> ("VISA Resource Name out"=w573:refnum<visa-resource-name>, "ID"=w530:dbl[], "IG"=w528:dbl[], "Outparams"=w552:T9, "error out"=w574:errorcluster)  [unwired: 3 in]
        n138 = Unbundle By Name(w552) -> ("Number of points"=w529:i32)  [unwired: 2 out]
        n139 = for {
          N: w529 -> [_]
          tunnel: [w588] -> w531 mode=indexing
          tunnel: w542 -> [w590]
          i -> [w589]
          n140 = Multiply(x=w590, y=w589) -> (x*y=w588:dbl)
        }
        n141 = Insert Into Array(array=dbl[][] [] ("Input Array"), new element=w531) -> (w543:dbl[][])  [unwired: 2 in]
        n142 = Insert Into Array(array=w543, new element=w530) -> (w548:dbl[][])  [unwired: 2 in]
        n143 = Insert Into Array(array=w548, new element=w528) -> (w547:dbl[][])  [unwired: 2 in]
        n144 = Transpose 2D Array(2D array=w547) -> (transposed array=w546:dbl[][])
        n145 = Open/Create/Replace File(file path (use dialog)=w577, error in=w574, operation (0:open)=w527) -> (refnum out=w585:refnum<file>, error out=w586:errorcluster)  [unwired: 3 in, 1 out]
        n146 = call "4155C Write array to file.vi"("Byte Stream File Refnum"=w585, "Header"=string[] ["Time /s", "Id /A", "Ig /A"], "Data Array"=w546, "error in (no error)"=w586) -> ("dup refnum"=w583:refnum<file>, "error out"=w584:errorcluster)  [unwired: 1 in]
        n147 = Close File(refnum=w583, error in=w584) -> (error out=w572:errorcluster)  [unwired: 1 out]
      }
      frame "transfer-fpp" {
        n148 = Number To Decimal String(number=w614) -> (decimal integer string=w668:string)  [unwired: 1 in]
        n149 = Bundle By Name(cluster=w644, "Emergency Stop"=w672) -> (w680:T1)
        n150 = Delete From Array(array=w659, index=0 ("Index")) -> (deleted portion=w657:string, array with subset deleted=w656:string[])  [unwired: 1 in]
        n151 = Concatenate Strings(w667, "-transferfpp-" ("Substring"), w668, w612, ".txt" ("Substring")) -> (w670:string)
        n152 = VISA Write(VISA resource name=w636, write buffer=":PAGE:CHAN:MODE SWE;" ("write buffer (\"\")"), error in (no error)=w635) -> (VISA resource name out=w633:refnum<visa-resource-name>, error out=w634:errorcluster)  [unwired: 1 out]
        n153 = case shown="\"d\", Default" w657 {
          tunnel: [w681 w682] -> w655
          frame "s" {
            w681 = u16 0 items=["Single", "Double"] ("sweep mode")
          }
          frame "d", Default {
            w682 = u16 1 items=["Single", "Double"] ("sweep mode")
          }
        }
        n154 = Fract/Exp String To Number(string=w656) -> (number=w640:dbl[])  [unwired: 3 in, 1 out]
        n155 = String To Path(string=w670) -> (path=w666:path)
        n156 = Index Array(array=w640, index #1=0 ("Index")) -> (element #1=w654:dbl, element #2=w653:dbl, element #3=w652:dbl)  [unwired: 2 in]
        n157 = Delete From Array(array=w640, length=3 ("Length"), index=0 ("Index")) -> (array with subset deleted=w638:dbl[])  [unwired: 1 out]
        n158 = Bundle By Name(cluster=w646, "Gate Start"=w654, "Gate Stop"=w653, "Gate Step (linear only)"=w652, "Gate Compliance"=w664, "Range mode"=w629, "Range"=w628) -> (w630:T6)
        n159 = Index Array(array=w638, index #1=0 ("Index")) -> (element #1=w649:dbl, element #2=w648:dbl, element #3=w647:dbl)  [unwired: 2 in]
        n160 = call <vilib>:"compatOverwrite.vi"("overwrite (F)"=TRUE) -> ("overwrite?"=w617:T8)
        n161 = Bundle By Name(cluster=w645, "Drain Start"=w649, "Drain Stop"=w648, "Drain Step"=w647, "Drain Compliance"=w665, "Range mode"=w627, "Range"=w626) -> (w631:T7)
        n162 = call "4155C Transfer-FPP.vi"("VISA resource name in"=w633, "Gate"=w630, "Drain"=w631, "Timings"=w663, "error in (no error)"=w634, "sweep mode"=w655, "Panel Controls"=w680) -> ("VG"=w671:dbl[], "Outparams"=w625:T9, "VISA Resource Name out"=w661:refnum<visa-resource-name>, "Vprobe2"=w621:dbl[], "ID"=w620:dbl[], "IG"=w619:dbl[], "Vprobe1"=w618:dbl[], "error out"=w662:errorcluster)  [unwired: 13 in]
        n163 = Unbundle By Name(w625) -> ("V2 Step"=w624:dbl, "V2 Start"=w623:dbl, "Number of points"=w622:i32)
        n164 = Open/Create/Replace File(file path (use dialog)=w666, error in=w662, operation (0:open)=w617) -> (refnum out=w677:refnum<file>, error out=w678:errorcluster)  [unwired: 3 in, 1 out]
        n165 = call "4155C Make Big 2d array FPP.vi"("1D Var1"=w671, "1d ID"=w620, "1d Vp2"=w621, "1d IG"=w619, "1d Vp1"=w618, "VAR2 START"=w623, "Number of VAR2 steps"=w622, "VAR2 STEP"=w624, "VAR1 Name"="Vg", "Decimal places in header"=i8 1, "VAR2 Name"="Vd") -> ("Header array"=w673:string[], "Data array"=w674:dbl[][])  [unwired: 15 in]
        n166 = call "4155C Write array to file.vi"("Byte Stream File Refnum"=w677, "Header"=w673, "Data Array"=w674, "error in (no error)"=w678) -> ("dup refnum"=w675:refnum<file>, "error out"=w676:errorcluster)  [unwired: 1 in]
        n167 = Close File(refnum=w675, error in=w676) -> (error out=w660:errorcluster)  [unwired: 1 out]
      }
      frame "output" {
        n168 = Number To Decimal String(number=w712) -> (decimal integer string=w761:string)  [unwired: 1 in]
        n169 = Bundle By Name(cluster=w738, "Emergency Stop"=w763) -> (w773:T1)
        n170 = Delete From Array(array=w753, index=0 ("Index")) -> (deleted portion=w751:string, array with subset deleted=w750:string[])  [unwired: 1 in]
        n171 = Concatenate Strings(w760, w683, w761, w711, "_O.txt" ("Suffix (output)")) -> (w762:string)
        n172 = VISA Write(VISA resource name=w729, write buffer=":PAGE:CHAN:MODE SWE;" ("write buffer (\"\")"), error in (no error)=w726) -> (VISA resource name out=w728:refnum<visa-resource-name>, error out=w727:errorcluster)  [unwired: 1 out]
        n173 = case shown="\"d\", Default" w751 {
          tunnel: [w774 w775] -> w749
          frame "s" {
            w774 = u16 0 items=["Single", "Double"] ("sweep mode")
          }
          frame "d", Default {
            w775 = u16 1 items=["Single", "Double"] ("sweep mode")
          }
        }
        n174 = Fract/Exp String To Number(string=w750) -> (number=w732:dbl[])  [unwired: 3 in, 1 out]
        n175 = String To Path(string=w762) -> (path=w759:path)
        n176 = Index Array(array=w732, index #1=0 ("Index")) -> (element #1=w748:dbl, element #2=w747:dbl, element #3=w746:dbl)  [unwired: 2 in]
        n177 = Delete From Array(array=w732, length=3 ("Length"), index=0 ("Index")) -> (array with subset deleted=w731:dbl[])  [unwired: 1 out]
        n178 = control-ref of="I vs Vd"() -> (w702:refnum<vi>)
        n179 = Bundle By Name(cluster=w740, "Gate Start"=w748, "Gate Stop"=w747, "Gate Step (linear only)"=w746, "Gate Compliance"=w757, "Range mode"=w724, "Range"=w723) -> (w772:T6)
        n180 = Index Array(array=w731, index #1=0 ("Index")) -> (element #1=w743:dbl, element #2=w742:dbl, element #3=w741:dbl)  [unwired: 2 in]
        n181 = call <vilib>:"compatOverwrite.vi"("overwrite (F)"=TRUE) -> ("overwrite?"=w716:T8)
        n182 = Bundle By Name(cluster=w739, "Drain Start"=w743, "Drain Stop"=w742, "Drain Step"=w741, "Drain Compliance"=w758, "Range mode"=w722, "Range"=w725) -> (w771:T7)
        n183 = call "4155C Output.vi"("VISA resource name in"=w728, "Gate"=w772, "Drain"=w771, "Timings"=w756, "error in (no error)"=w727, "SMU4"=w718, "sweep mode"=w749, "Panel controls"=w773) -> ("VD"=w709:dbl[], "Outparams"=w720:T9, "VISA Resource Name out"=w755:refnum<visa-resource-name>, "IS"=w708:dbl[], "ID"=w707:dbl[], "IG"=w706:dbl[], "error out"=w704:errorcluster, "SMU4"=w717:dbl[])  [unwired: 12 in]
        n184 = Unbundle By Name(w720) -> ("V2 Step"=w721:dbl, "V2 Start"=w719:dbl, "Number of points"=w701:i32)
        n185 = call "4155C Split array.vi"("Number of VAR2 steps"=w701, "Y2 data in"=w707, "X data in"=w709, "Y1 data in"=w708, "Y3 data in"=w706, "error in (no error)"=w704) -> ("Array of clusters"=w705:cluster{"Y data in":dbl[], "X data in":dbl[]}[], "error out"=w703:errorcluster)  [unwired: 1 in]
        n186 = local write "I vs Vd"(w705) -> ()
        n187 = call "4155C Config Chart Colours.vi"("Numeric"=w701, "XY Graph 2"=w702) -> ()  [unwired: 6 in]
        n188 = Open/Create/Replace File(file path (use dialog)=w759, error in=w703, operation (0:open)=w716) -> (refnum out=w768:refnum<file>, error out=w769:errorcluster)  [unwired: 3 in, 1 out]
        n189 = call "4155C Make Big 2d array.vi"("1D Var1"=w709, "1d IS"=w708, "1d ID"=w707, "1d IG"=w706, "1d SMU4"=w717, "SMU4"=w718, "VAR2 START"=w719, "Number of VAR2 steps"=w701, "VAR2 STEP"=w721, "VAR1 Name"="Vd", "Decimal places in header"=i8 1, "VAR2 Name"="Vg") -> ("Header array"=w764:string[], "Data array"=w765:dbl[][])  [unwired: 14 in]
        n190 = call "4155C Write array to file.vi"("Byte Stream File Refnum"=w768, "Header"=w764, "Data Array"=w765, "error in (no error)"=w769) -> ("dup refnum"=w766:refnum<file>, "error out"=w767:errorcluster)  [unwired: 1 in]
        n191 = Close File(refnum=w766, error in=w767) -> (error out=w754:errorcluster)  [unwired: 1 out]
      }
      frame "output2" {
        # "Adjusts graph colors."
        # "Adjusts graph colors."
        # "Is off"
        # "Is on"
        # "Ion will be the middle element of the array. The calculation of the index is done only once, since Is, Id, and Ig have the same dimensions."
        # "Ig off"
        # "Ig on"
        # "Is min"
        # "Is max"
        # "Ig min"
        # "Ig max"
        # "abs(Ig)"
        # "abs(Is)"
        # "Id min"
        # "Id max"
        # "Y1: Is\nY2: Id\nY3: Ig"
        # "abs(Id)"
        # "Adjusts graph colors."
        # "Adjusts graph colors."
        # "Id off"
        # "Id on"
        # "Adjusts graph colors."
        # "Time array"
        n192 = Delete From Array(array=w905, index=0 ("Index")) -> (deleted portion=w903:string, array with subset deleted=w902:string[])  [unwired: 1 in]
        n193 = Bundle By Name(cluster=w776, "Emergency Stop"=w914) -> (w867:T1)
        n194 = Number To Decimal String(number=w861) -> (decimal integer string=w860:string)  [unwired: 1 in]
        n195 = case shown="\"d\", Default" w903 {
          tunnel: [w916 w917] -> w901
          frame "s" {
            w916 = u16 0 items=["Single", "Double"] ("sweep mode")
          }
          frame "d", Default {
            w917 = u16 1 items=["Single", "Double"] ("sweep mode")
          }
        }
        n196 = Fract/Exp String To Number(string=w902) -> (number=w887:dbl[])  [unwired: 3 in, 1 out]
        n197 = Concatenate Strings(w912, w777, w860, w858, "_O_1_C_L.txt" ("Suffix (transfer)")) -> (w913:string)
        n198 = VISA Write(VISA resource name=w883, write buffer=":PAGE:CHAN:MODE SWE;" ("write buffer (\"\")"), error in (no error)=w882) -> (VISA resource name out=w880:refnum<visa-resource-name>, error out=w881:errorcluster)  [unwired: 1 out]
        n199 = String To Path(string=w913) -> (path=w911:path)
        n200 = Index Array(array=w887, index #1=0 ("Index")) -> (element #1=w900:dbl, element #2=w899:dbl, element #3=w898:dbl)  [unwired: 2 in]
        n201 = Delete From Array(array=w887, length=3 ("Length"), index=0 ("Index")) -> (array with subset deleted=w885:dbl[])  [unwired: 1 out]
        n202 = Build Array (concatenate)(w857, w853) -> (w803:i32[])
        n203 = Bundle By Name(cluster=w892, "Gate Start"=w900, "Gate Stop"=w899, "Gate Step (linear only)"=w898, "Gate Compliance"=w909, "Range mode"=w876, "Range"=w875) -> (w877:T6)
        n204 = control-ref of="Imax vs time"() -> (w832:refnum<vi>)
        n205 = control-ref of="Imin vs time"() -> (w831:refnum<vi>)
        n206 = control-ref of="Ion vs time"() -> (w800:refnum<vi>)
        n207 = control-ref of="Ioff vs time"() -> (w799:refnum<vi>)
        n208 = control-ref of="I vs Vg"() -> (w862:refnum<vi>)
        n209 = Index Array(array=w885, index #1=0 ("Index")) -> (element #1=w895:dbl, element #2=w894:dbl, element #3=w893:dbl)  [unwired: 2 in]
        n210 = call <vilib>:"compatOverwrite.vi"("overwrite (F)"=TRUE) -> ("overwrite?"=w866:T8)
        n211 = Bundle By Name(cluster=w891, "Drain Start"=w895, "Drain Stop"=w894, "Drain Step"=w893, "Drain Compliance"=w910, "Range mode"=w874, "Range"=w873) -> (w878:T7)
        n212 = call "4155C Output.vi"("VISA resource name in"=w880, "Gate"=w877, "Drain"=w878, "Timings"=w908, "error in (no error)"=w881, "SMU4"=w868, "sweep mode"=w901, "Panel controls"=w867) -> ("VD"=w865:dbl[], "Outparams"=w872:T9, "VISA Resource Name out"=w907:refnum<visa-resource-name>, "IS"=w828:dbl[], "ID"=w830:dbl[], "IG"=w827:dbl[], "error out"=w854:errorcluster, "SMU4"=w869:dbl[])  [unwired: 12 in]
        n213 = Unbundle By Name(w872) -> ("V2 Step"=w871:dbl, "V2 Start"=w870:dbl, "Number of points"=w797:i32)
        n214 = Absolute Value(x=w828) -> (abs(x)=w813:dbl[])
        n215 = Absolute Value(x=w830) -> (abs(x)=w829:dbl[])
        n216 = Absolute Value(x=w827) -> (abs(x)=w816:dbl[])
        n217 = Array Size(array=w829) -> (size(s)=w837:i32)
        n218 = Divide(x=w837, y=2) -> (x/y=w780:dbl)
        n219 = Subtract(x=w780, y=1) -> (x-y=w779:dbl)
        n220 = Array Max & Min(array=w813) -> (max value=w820:dbl, min value=w821:dbl)  [unwired: 2 out]
        n221 = Array Max & Min(array=w829) -> (max value=w863:dbl, min value=w826:dbl)  [unwired: 2 out]
        n222 = Array Max & Min(array=w816) -> (max value=w825:dbl, min value=w824:dbl)  [unwired: 2 out]
        n223 = call "4155C Split array.vi"("Number of VAR2 steps"=w797, "Y2 data in"=w830, "X data in"=w865, "Y1 data in"=w828, "Y3 data in"=w827, "error in (no error)"=w854) -> ("Array of clusters"=w856:cluster{"Y data in":dbl[], "X data in":dbl[]}[], "error out"=w785:errorcluster)  [unwired: 1 in]
        n224 = Index Array(array=w813, index=w779) -> (element=w804:dbl)
        n225 = Index Array(array=w813, index=0) -> (element=w805:dbl)
        n226 = Index Array(array=w829, index=w779) -> (element=w806:dbl)
        n227 = Index Array(array=w829, index=0) -> (element=w807:dbl)
        n228 = Index Array(array=w816, index=w779) -> (element=w809:dbl)
        n229 = Index Array(array=w816, index=0) -> (element=w808:dbl)
        n230 = local write "Ig max"(w825) -> ()
        n231 = local write "Ig min"(w824) -> ()
        n232 = local write "Is max"(w820) -> ()
        n233 = local write "Is min"(w821) -> ()
        n234 = local write "Id max"(w863) -> ()
        n235 = local write "Id min"(w826) -> ()
        n236 = local write "I vs Vd"(w856) -> ()
        n237 = Build Array (concatenate)(w819, w820) -> (w798:dbl[])
        n238 = Build Array (concatenate)(w818, w821) -> (w796:dbl[])
        n239 = local write "Is off"(w805) -> ()
        n240 = local write "Is on"(w804) -> ()
        n241 = Build Array (concatenate)(w864, w863) -> (w795:dbl[])
        n242 = Build Array (concatenate)(w851, w826) -> (w794:dbl[])
        n243 = Build Array (concatenate)(w823, w825) -> (w793:dbl[])
        n244 = Build Array (concatenate)(w822, w824) -> (w792:dbl[])
        n245 = Build Array (concatenate)(w811, w804) -> (w791:dbl[])
        n246 = Build Array (concatenate)(w810, w805) -> (w790:dbl[])
        n247 = Build Array (concatenate)(w833, w806) -> (w789:dbl[])
        n248 = Build Array (concatenate)(w834, w807) -> (w788:dbl[])
        n249 = Build Array (concatenate)(w815, w809) -> (w787:dbl[])
        n250 = Build Array (concatenate)(w814, w808) -> (w786:dbl[])
        n251 = local write "Ig off"(w808) -> ()
        n252 = local write "Ig on"(w809) -> ()
        n253 = local write "Id off"(w807) -> ()
        n254 = local write "Id on"(w806) -> ()
        n255 = call "4155C Split array.vi"("Number of VAR2 steps"=w797, "Y2 data in"=w789, "X data in"=w803, "Y1 data in"=w791, "Y3 data in"=w787, "error in (no error)"=w785) -> ("Array of clusters"=w801:cluster{"Y data in":dbl[], "X data in":dbl[]}[], "error out"=w784:errorcluster)  [unwired: 1 in]
        n256 = call "4155C Split array.vi"("Number of VAR2 steps"=w797, "Y2 data in"=w788, "X data in"=w803, "Y1 data in"=w790, "Y3 data in"=w786, "error in (no error)"=w784) -> ("Array of clusters"=w802:cluster{"Y data in":dbl[], "X data in":dbl[]}[], "error out"=w783:errorcluster)  [unwired: 1 in]
        n257 = call "4155C Split array.vi"("Number of VAR2 steps"=w797, "Y2 data in"=w795, "X data in"=w803, "Y1 data in"=w798, "Y3 data in"=w793, "error in (no error)"=w783) -> ("Array of clusters"=w855:cluster{"Y data in":dbl[], "X data in":dbl[]}[], "error out"=w782:errorcluster)  [unwired: 1 in]
        n258 = call "4155C Split array.vi"("Number of VAR2 steps"=w797, "Y2 data in"=w794, "X data in"=w803, "Y1 data in"=w796, "Y3 data in"=w792, "error in (no error)"=w782) -> ("Array of clusters"=w852:cluster{"Y data in":dbl[], "X data in":dbl[]}[], "error out"=w781:errorcluster)  [unwired: 1 in]
        n259 = Open/Create/Replace File(file path (use dialog)=w911, error in=w781, operation (0:open)=w866) -> (refnum out=w849:refnum<file>, error out=w847:errorcluster)  [unwired: 3 in, 1 out]
        n260 = call "4155C Make Big 2d array.vi"("1D Var1"=w865, "1d IS"=w828, "1d ID"=w830, "1d IG"=w827, "1d SMU4"=w869, "SMU4"=w868, "VAR2 START"=w870, "Number of VAR2 steps"=w797, "VAR2 STEP"=w871, "VAR1 Name"="Vd", "Decimal places in header"=i8 1, "VAR2 Name"="Vg") -> ("Header array"=w850:string[], "Data array"=w848:dbl[][])  [unwired: 14 in]
        n261 = local write "Imax vs time"(w855) -> ()
        n262 = local write "Imin vs time"(w852) -> ()
        n263 = local write "Ion vs time"(w801) -> ()
        n264 = local write "Ioff vs time"(w802) -> ()
        n265 = call "4155C Config Chart Colours.vi"("Numeric"=w797, "XY Graph 2"=w832) -> ()  [unwired: 6 in]
        n266 = call "4155C Config Chart Colours.vi"("Numeric"=w797, "XY Graph 2"=w831) -> ()  [unwired: 6 in]
        n267 = call "4155C Config Chart Colours.vi"("Numeric"=w797, "XY Graph 2"=w800) -> ()  [unwired: 6 in]
        n268 = call "4155C Config Chart Colours.vi"("Numeric"=w797, "XY Graph 2"=w799) -> ()  [unwired: 6 in]
        n269 = call "4155C Config Chart Colours.vi"("Numeric"=w797, "XY Graph 2"=w862) -> ()  [unwired: 6 in]
        n270 = call "4155C Write array to file.vi"("Byte Stream File Refnum"=w849, "Header"=w850, "Data Array"=w848, "error in (no error)"=w847) -> ("dup refnum"=w846:refnum<file>, "error out"=w845:errorcluster)  [unwired: 1 in]
        n271 = Close File(refnum=w846, error in=w845) -> (error out=w906:errorcluster)  [unwired: 1 out]
      }
      frame "output-fpp" {
        n272 = Number To Decimal String(number=w938) -> (decimal integer string=w992:string)  [unwired: 1 in]
        n273 = Bundle By Name(cluster=w968, "Emergency Stop"=w995) -> (w1005:T1)
        n274 = Delete From Array(array=w983, index=0 ("Index")) -> (deleted portion=w981:string, array with subset deleted=w980:string[])  [unwired: 1 in]
        n275 = VISA Write(VISA resource name=w959, write buffer=":PAGE:CHAN:MODE SWE;" ("write buffer (\"\")"), error in (no error)=w956) -> (VISA resource name out=w958:refnum<visa-resource-name>, error out=w957:errorcluster)  [unwired: 1 out]
        n276 = Concatenate Strings(w991, "-outputfpp-" ("Substring"), w992, w937, ".txt" ("Substring")) -> (w994:string)
        n277 = case shown="\"d\", Default" w981 {
          tunnel: [w1006 w1007] -> w979
          frame "s" {
            w1006 = u16 0 items=["Single", "Double"] ("sweep mode")
          }
          frame "d", Default {
            w1007 = u16 1 items=["Single", "Double"] ("sweep mode")
          }
        }
        n278 = Fract/Exp String To Number(string=w980) -> (number=w962:dbl[])  [unwired: 3 in, 1 out]
        n279 = String To Path(string=w994) -> (path=w990:path)
        n280 = Index Array(array=w962, index #1=0 ("Index")) -> (element #1=w978:dbl, element #2=w977:dbl, element #3=w976:dbl)  [unwired: 2 in]
        n281 = Delete From Array(array=w962, length=3 ("Length"), index=0 ("Index")) -> (array with subset deleted=w961:dbl[])  [unwired: 1 out]
        n282 = Bundle By Name(cluster=w970, "Gate Start"=w978, "Gate Stop"=w977, "Gate Step (linear only)"=w976, "Gate Compliance"=w988, "Range mode"=w954, "Range"=w953) -> (w1004:T6)
        n283 = Index Array(array=w961, index #1=0 ("Index")) -> (element #1=w973:dbl, element #2=w972:dbl, element #3=w971:dbl)  [unwired: 2 in]
        n284 = call <vilib>:"compatOverwrite.vi"("overwrite (F)"=TRUE) -> ("overwrite?"=w942:T8)
        n285 = Bundle By Name(cluster=w969, "Drain Start"=w973, "Drain Stop"=w972, "Drain Step"=w971, "Drain Compliance"=w989, "Range mode"=w952, "Range"=w955) -> (w1003:T7)
        n286 = call "4155C Output-FPP.vi"("VISA resource name in"=w958, "Gate"=w1004, "Drain"=w1003, "Timings"=w987, "error in (no error)"=w957, "sweep mode"=w979, "Panel controls"=w1005) -> ("VD"=w947:dbl[], "Outparams"=w950:T9, "VISA Resource Name out"=w985:refnum<visa-resource-name>, "Vprobe2"=w946:dbl[], "ID"=w945:dbl[], "IG"=w944:dbl[], "Vprobe1"=w943:dbl[], "error out"=w986:errorcluster)  [unwired: 13 in]
        n287 = Unbundle By Name(w950) -> ("V2 Step"=w951:dbl, "V2 Start"=w949:dbl, "Number of points"=w948:i32)
        n288 = Open/Create/Replace File(file path (use dialog)=w990, error in=w986, operation (0:open)=w942) -> (refnum out=w1000:refnum<file>, error out=w1001:errorcluster)  [unwired: 3 in, 1 out]
        n289 = call "4155C Make Big 2d array FPP.vi"("1D Var1"=w947, "1d ID"=w945, "1d Vp2"=w946, "1d IG"=w944, "1d Vp1"=w943, "VAR2 START"=w949, "Number of VAR2 steps"=w948, "VAR2 STEP"=w951, "VAR1 Name"="Vd", "Decimal places in header"=i8 1, "VAR2 Name"="Vg") -> ("Header array"=w996:string[], "Data array"=w997:dbl[][])  [unwired: 15 in]
        n290 = call "4155C Write array to file.vi"("Byte Stream File Refnum"=w1000, "Header"=w996, "Data Array"=w997, "error in (no error)"=w1001) -> ("dup refnum"=w998:refnum<file>, "error out"=w999:errorcluster)  [unwired: 1 in]
        n291 = Close File(refnum=w998, error in=w999) -> (error out=w984:errorcluster)  [unwired: 1 out]
      }
      frame "itime" {
        n292 = Delete From Array(array=w1010, index=1) -> (deleted portion=w1009:string)  [unwired: 1 in, 1 out]
        n293 = Delete From Array(array=w1010, index=0 ("Index")) -> (deleted portion=w1044:string)  [unwired: 1 in, 1 out]
        n294 = Fract/Exp String To Number(string=w1009) -> (number=w1008:dbl)  [unwired: 3 in, 1 out]
        n295 = case shown="\"l\"" w1044 {
          tunnel: w1043 -> [w1049 w1051 w1055]
          tunnel: [w1048 w1050 w1054] -> w1036
          tunnel: w1008 -> [w1046 _ w1053]
          frame "s" {
            w1047 = u32 0 items=["short  ", "medium  ", "long  "] ("integration time 2")
            n296 = Bundle By Name(cluster=w1049, "integration time"=w1047, "Short/Long integration time"=w1046) -> (w1048:T5)
          }
          frame "m", Default {
            w1052 = u32 1 items=["short  ", "medium  ", "long  "] ("integration time 2")
            n297 = Bundle By Name(cluster=w1051, "integration time"=w1052) -> (w1050:T5)
          }
          frame "l" {
            w1056 = u32 2 items=["short  ", "medium  ", "long  "] ("integration time 2")
            n298 = Bundle By Name(cluster=w1055, "integration time"=w1056, "Short/Long integration time"=w1053) -> (w1054:T5)
          }
        }
      }
      frame "pulsed" {
        n299 = Delete From Array(array=w1090, index=0 ("Index")) -> (deleted portion=w1091:string, array with subset deleted=w1078:string[])  [unwired: 1 in]
        n300 = case shown="\"on\", Default" w1091 {
          tunnel: w1089 -> [w1101 w1104]
          tunnel: [w1100 w1103] -> w1082
          tunnel: w1078 -> [w1098 _]
          frame "on", Default {
            w1099 = u16 1 items=["Continuous", "Pulsed"] ("sweep method")
            n301 = Fract/Exp String To Number(string=w1098) -> (number=w1096:dbl[])  [unwired: 3 in, 1 out]
            n302 = Index Array(array=w1096, index #1=0 ("Index")) -> (element #1=w1095:dbl, element #2=w1094:dbl, element #3=w1093:dbl)  [unwired: 2 in]
            n303 = Bundle By Name(cluster=w1101, "sweep method"=w1099, "Pulse period"=w1095, "Base voltage"=w1094, "Pulse width"=w1093) -> (w1100:T5)
          }
          frame "off" {
            w1102 = u16 0 items=["Continuous", "Pulsed"] ("sweep method")
            n304 = Bundle By Name(cluster=w1104, "sweep method"=w1102) -> (w1103:T5)
          }
        }
      }
      frame "gaterangemode" {
        n305 = Delete From Array(array=w1136, index=0 ("Index")) -> (deleted portion=w1137:string)  [unwired: 1 in, 1 out]
        n306 = case shown="\"f\"" w1137 {
          tunnel: [w1139 w1140 w1141] -> w1126
          frame "a", Default {
            w1139 = u16 0 items=["Auto", "Limited", "Fixed"] ("Gate Range\nmode 2")
          }
          frame "f" {
            w1140 = u16 2 items=["Auto", "Limited", "Fixed"] ("Gate Range\nmode 2")
          }
          frame "l" {
            w1141 = u16 1 items=["Auto", "Limited", "Fixed"] ("Gate Range\nmode 2")
          }
        }
      }
      frame "gaterange" {
        (unwired) u8 11 items=["10fA  ", "100fA  ", "1nA  ", "10nA", "100nA", "1uA", "10uA", "100uA", "1mA", "10mA", "100mA", "1A"] ("Gate Range 2")
        n307 = Delete From Array(array=w1180, index=0 ("Index")) -> (deleted portion=w1170:string)  [unwired: 1 in, 1 out]
        n308 = Scan Value(string=w1170, format string="") -> (value=w1168:dbl)  [unwired: 1 in, 1 out]
        n309 = Logarithm Base 10(1:w1168) -> (0:w1167:dbl)
        n310 = Round To Nearest(number=w1167) -> (nearest integer value=w1166:dbl)
        n311 = Add(x=w1166, y=11.0) -> (x+y=w1164:dbl)
        n312 = To Unsigned Byte Integer(number=w1164) -> (unsigned 8bit integer=w1163:u8)
      }
      frame "drainrange" {
        (unwired) u8 11 items=["10fA  ", "100fA  ", "1nA  ", "10nA", "100nA", "1uA", "10uA", "100uA", "1mA", "10mA", "100mA", "1A"] ("Gate Range 2")
        n313 = Delete From Array(array=w1220, index=0 ("Index")) -> (deleted portion=w1211:string)  [unwired: 1 in, 1 out]
        n314 = Scan Value(string=w1211, format string="") -> (value=w1209:dbl)  [unwired: 1 in, 1 out]
        n315 = Logarithm Base 10(1:w1209) -> (0:w1208:dbl)
        n316 = Round To Nearest(number=w1208) -> (nearest integer value=w1207:dbl)
        n317 = Add(x=w1207, y=11.0) -> (x+y=w1205:dbl)
        n318 = To Unsigned Byte Integer(number=w1205) -> (unsigned 8bit integer=w1204:u8)
      }
      frame "drainrangemode" {
        n319 = Delete From Array(array=w1253, index=0 ("Index")) -> (deleted portion=w1254:string)  [unwired: 1 in, 1 out]
        n320 = case shown="\"f\"" w1254 {
          tunnel: [w1256 w1257 w1258] -> w1243
          frame "a", Default {
            w1256 = u16 0 items=["Auto", "Limited", "Fixed"] ("Gate Range\nmode 2")
          }
          frame "f" {
            w1257 = u16 2 items=["Auto", "Limited", "Fixed"] ("Gate Range\nmode 2")
          }
          frame "l" {
            w1258 = u16 1 items=["Auto", "Limited", "Fixed"] ("Gate Range\nmode 2")
          }
        }
      }
      frame "Error", Default {
      }
      frame "logfile" {
        n321 = Number To Decimal String(number=w1311) -> (decimal integer string=w1346:string)  [unwired: 1 in]
        n322 = Concatenate Strings(w1345, "logfile" ("Substring"), w1346, w1309, ".txt" ("Substring")) -> (w1343:string)
        n323 = String To Path(string=w1343) -> (path=w1316:path)
        n324 = Unbundle(w1342) -> ("integration time"=w1341:u32, "Short/Long integration time"=w1340:dbl, "hold time (sec)"=w1339:dbl, "delay time (sec)"=w1338:dbl, "Step Time (0 disables)"=w1337:dbl, "sweep method"=w1336:u16, "Pulse period"=w1335:dbl, "Base voltage"=w1334:dbl, "Pulse width"=w1333:dbl)
        n325 = Build Array(w1341, w1340, w1339, w1338, w1337, w1336, w1335, w1334, w1333, w1327, w1328, w1329, w1330, w1331, w1332) -> (w1320:dbl[])
        n326 = Insert Into Array(array=dbl[][] [] ("Input Array"), new element=w1320) -> (w1319:dbl[][])  [unwired: 2 in]
        n327 = call <vilib>:"compatOverwrite.vi"("overwrite (F)"=TRUE) -> ("overwrite?"=w1314:T8)
        n328 = Open/Create/Replace File(file path (use dialog)=w1316, error in=w1318, operation (0:open)=w1314) -> (refnum out=w1324:refnum<file>, error out=w1323:errorcluster)  [unwired: 3 in, 1 out]
        n329 = call "4155C Write array to file.vi"("Byte Stream File Refnum"=w1324, "Header"=string[] ["Int Time", "Short/Long Itime", "Hold time", "Delay time", "Step time", "Sweep method", "Pulse period", "Base Voltage", "Pulse width", "Drain compliance", "Gate compliance", "Gate range mode", "Gate range", "S/D range mode", "S/D range"], "Data Array"=w1319, "error in (no error)"=w1323) -> ("dup refnum"=w1326:refnum<file>, "error out"=w1325:errorcluster)  [unwired: 1 in]
        n330 = Close File(refnum=w1326, error in=w1325) -> (error out=w1317:errorcluster)  [unwired: 1 out]
      }
      frame "sample" {
        n331 = Number To Decimal String(number=w1369) -> (decimal integer string=w1417:string)  [unwired: 1 in]
        n332 = Fract/Exp String To Number(string=w1414) -> (number=w1375:dbl[])  [unwired: 3 in, 1 out]
        n333 = Concatenate Strings(w1392, "-sample-" ("Substring"), w1417, w1367, ".txt" ("Substring")) -> (w1415:string)
        n334 = Index Array(array=w1375, index=0 ("Index")) -> (element=w1412:dbl)
        n335 = String To Path(string=w1415) -> (path=w1396:path)
        n336 = Index Array(array=w1375, index=2 ("Index")) -> (element=w1408:dbl)
        n337 = Index Array(array=w1375, index=3 ("Index")) -> (element=w1377:dbl)
        n338 = Index Array(array=w1375, index=4 ("Index")) -> (element=w1374:dbl)
        n339 = call "4155C Config Sampling Measurements.vi"("Sampling interval"=w1374, "Sample time"=w1377, "Display on/off"=TRUE, "Timings"=w1383, "Num Points"=w1408, "error in (no error)"=w1419, "Drain Compliance"=w1418, "Gate Compliance"=w1393, "VISA session"=w1420) -> ("error out"=w1421:errorcluster, "dup VISA resource name"=w1422:refnum<visa-resource-name>)  [unwired: 1 in]
        n340 = Index Array(array=w1375, index=1 ("Index")) -> (element=w1409:dbl)
        n341 = call "4155C Take Sample.vi"("Emergency Stop"=w1389, "error in (no error)"=w1421, "Vd"=w1409, "Vg"=w1412, "VISA resource name in"=w1422) -> ("error out"=w1387:errorcluster, "Id"=w1424:dbl[], "Ig"=w1398:dbl[], "VISA Resource Name out"=w1385:refnum<visa-resource-name>, "Is"=w1423:dbl[], "Time"=w1402:dbl[])  [unwired: 1 in]
        n342 = Insert Into Array(array=dbl[][] [] ("Input Array"), new element=w1402) -> (w1401:dbl[][])  [unwired: 2 in]
        n343 = Insert Into Array(array=w1401, new element=w1398) -> (w1400:dbl[][])  [unwired: 2 in]
        n344 = Insert Into Array(array=w1400, new element=w1424) -> (w1399:dbl[][])  [unwired: 2 in]
        n345 = VISA Write(VISA resource name=w1385, write buffer=":DISP ON" ("write buffer (\"\")"), error in (no error)=w1387) -> (VISA resource name out=w1384:refnum<visa-resource-name>, error out=w1386:errorcluster)  [unwired: 1 out]
        n346 = Insert Into Array(array=w1399, new element=w1423) -> (w1391:dbl[][])  [unwired: 2 in]
        n347 = Transpose 2D Array(2D array=w1391) -> (transposed array=w1390:dbl[][])
        n348 = call <vilib>:"compatOverwrite.vi"("overwrite (F)"=TRUE) -> ("overwrite?"=w1372:T8)
        n349 = Open/Create/Replace File(file path (use dialog)=w1396, error in=w1386, operation (0:open)=w1372) -> (refnum out=w1405:refnum<file>, error out=w1404:errorcluster)  [unwired: 3 in, 1 out]
        n350 = call "4155C Write array to file.vi"("Byte Stream File Refnum"=w1405, "Header"=string[] ["Time /s", "Ig /A", "Id /A", "Is /A"], "Data Array"=w1390, "error in (no error)"=w1404) -> ("dup refnum"=w1407:refnum<file>, "error out"=w1406:errorcluster)  [unwired: 1 in]
        n351 = Close File(refnum=w1407, error in=w1406) -> (error out=w1394:errorcluster)  [unwired: 1 out]
      }
      frame "samplei" {
        n352 = Number To Decimal String(number=w1446) -> (decimal integer string=w1497:string)  [unwired: 1 in]
        n353 = Concatenate Strings(w1476, "-samplei-" ("Substring"), w1497, w1445, ".txt" ("Substring")) -> (w1495:string)
        n354 = Fract/Exp String To Number(string=w1494) -> (number=w1461:dbl[])  [unwired: 3 in, 1 out]
        n355 = String To Path(string=w1495) -> (path=w1479:path)
        n356 = Index Array(array=w1461, index=4 ("Index")) -> (element=w1455:dbl)
        n357 = Index Array(array=w1461, index=3 ("Index")) -> (element=w1456:dbl)
        n358 = Index Array(array=w1461, index=1 ("Index")) -> (element=w1458:dbl)
        n359 = Index Array(array=w1461, index=0 ("Index")) -> (element=w1459:dbl)
        n360 = Index Array(array=w1461, index=2 ("Index")) -> (element=w1457:dbl)
        n361 = call "4155C Config SamplingI Measurements.vi"("Sample time"=w1457, "Display on/off"=TRUE, "Timings"=w1468, "Num Points"=w1458, "error in (no error)"=w1499, "Sampling interval"=w1456, "VISA session"=w1500) -> ("error out"=w1501:errorcluster, "dup VISA resource name"=w1502:refnum<visa-resource-name>)  [unwired: 3 in]
        n362 = call "4155C Take SampleI.vi"("Emergency Stop"=w1473, "error in (no error)"=w1501, "Idg 2"=w1459, "Vdg compliance 2"=w1455, "VISA resource name in"=w1502) -> ("error out"=w1471:errorcluster, "Idg"=w1504:dbl[], "Vdg"=w1481:dbl[], "VISA Resource Name out"=w1469:refnum<visa-resource-name>, "Is"=w1503:dbl[], "Time"=w1485:dbl[])  [unwired: 1 in]
        n363 = Insert Into Array(array=dbl[][] [] ("Input Array"), new element=w1485) -> (w1484:dbl[][])  [unwired: 2 in]
        n364 = Insert Into Array(array=w1484, new element=w1481) -> (w1483:dbl[][])  [unwired: 2 in]
        n365 = Insert Into Array(array=w1483, new element=w1504) -> (w1482:dbl[][])  [unwired: 2 in]
        n366 = VISA Write(VISA resource name=w1469, write buffer=":DISP ON" ("write buffer (\"\")"), error in (no error)=w1471) -> (VISA resource name out=w1454:refnum<visa-resource-name>, error out=w1470:errorcluster)  [unwired: 1 out]
        n367 = Insert Into Array(array=w1482, new element=w1503) -> (w1475:dbl[][])  [unwired: 2 in]
        n368 = call <vilib>:"compatOverwrite.vi"("overwrite (F)"=TRUE) -> ("overwrite?"=w1449:T8)
        n369 = Open/Create/Replace File(file path (use dialog)=w1479, error in=w1470, operation (0:open)=w1449) -> (refnum out=w1488:refnum<file>, error out=w1487:errorcluster)  [unwired: 3 in, 1 out]
        n370 = Transpose 2D Array(2D array=w1475) -> (transposed array=w1474:dbl[][])
        n371 = call "4155C Write array to file.vi"("Byte Stream File Refnum"=w1488, "Header"=string[] ["Time /s", "Vdg /V", "Idg /A", "Is /A"], "Data Array"=w1474, "error in (no error)"=w1487) -> ("dup refnum"=w1490:refnum<file>, "error out"=w1489:errorcluster)  [unwired: 1 in]
        n372 = Close File(refnum=w1490, error in=w1489) -> (error out=w1452:errorcluster)  [unwired: 1 out]
        n373 = VISA Write(VISA resource name=w1454, write buffer=";:PAGE:SCON:STAN OFF;:PAGE:CHAN:VSU2:DIS;" ("write buffer (\"\")"), error in (no error)=w1452) -> (VISA resource name out=w1450:refnum<visa-resource-name>, error out=w1451:errorcluster)  [unwired: 1 out]
      }
      frame "#" {
        n374 = VISA Write(VISA resource name=w1530, write buffer=":DISP ON" ("write buffer (\"\")"), error in (no error)=w1529) -> (VISA resource name out=w1528:refnum<visa-resource-name>, error out=w1527:errorcluster)  [unwired: 1 out]
      }
      frame "stressV" {
        n375 = Number To Decimal String(number=w1559) -> (decimal integer string=w1600:string)  [unwired: 1 in]
        n376 = Concatenate Strings(w1584, "-stressV-" ("Substring"), w1600, w1558, ".txt" ("Substring")) -> (w1598:string)
        n377 = Fract/Exp String To Number(string=w1597) -> (number=w1570:dbl[])  [unwired: 3 in, 1 out]
        n378 = String To Path(string=w1598) -> (path=w1588:path)
        n379 = Index Array(array=w1570, index=3 ("Index")) -> (element=w1567:dbl)
        n380 = Index Array(array=w1570, index=1 ("Index")) -> (element=w1565:dbl)
        n381 = Index Array(array=w1570, index=0 ("Index")) -> (element=w1564:dbl)
        n382 = Index Array(array=w1570, index=4 ("Index")) -> (element=w1569:dbl)
        n383 = Index Array(array=w1570, index=2 ("Index")) -> (element=w1566:dbl)
        n384 = call "4155C Config V Stress.vi"("VISA session"=w1603, "ID compliance"=w1567, "VD"=w1565, "VG"=w1564, "IG compliance"=w1566, "error in (no error)"=w1602, "Display on/off"=TRUE) -> ("dup VISA resource name"=w1605:refnum<visa-resource-name>, "error out"=w1604:errorcluster)
        n385 = call "4155C Apply Stress.vi"("error in (no error)"=w1604, "Duration"=w1569, "Emergency Stop"=w1583, "VISA resource name in"=w1605) -> ("error out"=w1581:errorcluster, "VISA Resource Name out"=w1579:refnum<visa-resource-name>)
        n386 = VISA Write(VISA resource name=w1579, write buffer=":DISP ON" ("write buffer (\"\")"), error in (no error)=w1581) -> (VISA resource name out=w1578:refnum<visa-resource-name>, error out=w1580:errorcluster)  [unwired: 1 out]
        n387 = call <vilib>:"compatOverwrite.vi"("overwrite (F)"=TRUE) -> ("overwrite?"=w1563:T8)
        n388 = Open/Create/Replace File(file path (use dialog)=w1588, error in=w1580, operation (0:open)=w1563) -> (refnum out=w1591:refnum<file>, error out=w1590:errorcluster)  [unwired: 3 in, 1 out]
        n389 = call "4155C Write array to file.vi"("Byte Stream File Refnum"=w1591, "Header"=string[] ["V stress completed successfully", ""], "error in (no error)"=w1590) -> ("dup refnum"=w1593:refnum<file>, "error out"=w1592:errorcluster)  [unwired: 2 in]
        n390 = Close File(refnum=w1593, error in=w1592) -> (error out=w1586:errorcluster)  [unwired: 1 out]
      }
      frame "stressI" {
        n391 = Number To Decimal String(number=w1626) -> (decimal integer string=w1663:string)  [unwired: 1 in]
        n392 = Concatenate Strings(w1647, "-stressI-" ("Substring"), w1663, w1625, ".txt" ("Substring")) -> (w1661:string)
        n393 = Fract/Exp String To Number(string=w1660) -> (number=w1635:dbl[])  [unwired: 3 in, 1 out]
        n394 = Index Array(array=w1635, index=1 ("Index")) -> (element=w1631:dbl)
        n395 = Index Array(array=w1635, index=0 ("Index")) -> (element=w1632:dbl)
        n396 = call "4155C Config I Stress.vi"("VISA session"=w1666, "IDG"=w1632, "VDG compliance"=w1631, "error in (no error)"=w1665, "Display on/off"=TRUE) -> ("dup VISA resource name"=w1668:refnum<visa-resource-name>, "error out"=w1667:errorcluster)
        n397 = Index Array(array=w1635, index=2 ("Index")) -> (element=w1633:dbl)
        n398 = String To Path(string=w1661) -> (path=w1651:path)
        n399 = call "4155C Apply Stress.vi"("error in (no error)"=w1667, "Duration"=w1633, "Emergency Stop"=w1646, "VISA resource name in"=w1668) -> ("error out"=w1644:errorcluster, "VISA Resource Name out"=w1642:refnum<visa-resource-name>)
        n400 = VISA Write(VISA resource name=w1642, write buffer=":DISP ON" ("write buffer (\"\")"), error in (no error)=w1644) -> (VISA resource name out=w1641:refnum<visa-resource-name>, error out=w1643:errorcluster)  [unwired: 1 out]
        n401 = call <vilib>:"compatOverwrite.vi"("overwrite (F)"=TRUE) -> ("overwrite?"=w1630:T8)
        n402 = Open/Create/Replace File(file path (use dialog)=w1651, error in=w1643, operation (0:open)=w1630) -> (refnum out=w1654:refnum<file>, error out=w1653:errorcluster)  [unwired: 3 in, 1 out]
        n403 = call "4155C Write array to file.vi"("Byte Stream File Refnum"=w1654, "Header"=string[] ["I stress completed successfully", ""], "error in (no error)"=w1653) -> ("dup refnum"=w1656:refnum<file>, "error out"=w1655:errorcluster)  [unwired: 2 in]
        n404 = Close File(refnum=w1656, error in=w1655) -> (error out=w1649:errorcluster)  [unwired: 1 out]
      }
      frame "vsu2pulse" {
        n405 = Number To Decimal String(number=w1689) -> (decimal integer string=w1724:string)  [unwired: 1 in]
        n406 = Concatenate Strings(w1709, "-vsu2-" ("Substring"), w1724, w1688, ".txt" ("Substring")) -> (w1722:string)
        n407 = Fract/Exp String To Number(string=w1721) -> (number=w1697:dbl[])  [unwired: 3 in, 1 out]
        n408 = String To Path(string=w1722) -> (path=w1713:path)
        n409 = Index Array(array=w1697, index=1 ("Index")) -> (element=w1696:dbl)
        n410 = Index Array(array=w1697, index=0 ("Index")) -> (element=w1694:dbl)
        n411 = call "4155C Config VSU2 Stress.vi"("error in (no error)"=w1726, "VSU2"=w1694, "Display on/off"=TRUE, "VISA session"=w1727) -> ("error out"=w1728:errorcluster, "dup VISA resource name"=w1729:refnum<visa-resource-name>)
        n412 = call "4155C Apply Stress.vi"("error in (no error)"=w1728, "Duration"=w1696, "Emergency Stop"=w1708, "VISA resource name in"=w1729) -> ("error out"=w1706:errorcluster, "VISA Resource Name out"=w1704:refnum<visa-resource-name>)
        n413 = VISA Write(VISA resource name=w1704, write buffer=":DISP ON" ("write buffer (\"\")"), error in (no error)=w1706) -> (VISA resource name out=w1703:refnum<visa-resource-name>, error out=w1705:errorcluster)  [unwired: 1 out]
        n414 = call <vilib>:"compatOverwrite.vi"("overwrite (F)"=TRUE) -> ("overwrite?"=w1693:T8)
        n415 = Open/Create/Replace File(file path (use dialog)=w1713, error in=w1705, operation (0:open)=w1693) -> (refnum out=w1716:refnum<file>, error out=w1715:errorcluster)  [unwired: 3 in, 1 out]
        n416 = call "4155C Write array to file.vi"("Byte Stream File Refnum"=w1716, "Header"=string[] ["VSU2 pulse completed successfully", ""], "error in (no error)"=w1715) -> ("dup refnum"=w1718:refnum<file>, "error out"=w1717:errorcluster)  [unwired: 2 in]
        n417 = Close File(refnum=w1718, error in=w1717) -> (error out=w1711:errorcluster)  [unwired: 1 out]
      }
      frame "sample-fpp" {
        w1761 = string[] ["Time /s", "Id VgVd /A", "Ig VgVd /A", "Vp1 VgVd /V", "Vp2 VgVd /V"] ("Header")
        w1765 = "%d" ("format string")
        n418 = Number To Decimal String(number=w1750) -> (decimal integer string=w1813:string)  [unwired: 1 in]
        n419 = Fract/Exp String To Number(string=w1810) -> (number=w1798:dbl[])  [unwired: 3 in, 1 out]
        n420 = Concatenate Strings(w1804, "-samplefpp-" ("Substring"), w1813, w1749, ".txt" ("Substring")) -> (w1811:string)
        n421 = String To Path(string=w1811) -> (path=w1773:path)
        n422 = Index Array(array=w1798, index=0 ("Index")) -> (element=w1759:dbl)
        n423 = Index Array(array=w1798, index=1 ("Index")) -> (element=w1758:dbl)
        n424 = Index Array(array=w1798, index=2 ("Index")) -> (element=w1806:dbl)
        n425 = Index Array(array=w1798, index=3 ("Index")) -> (element=w1796:dbl)
        n426 = call "4155C Config Sampling Measurements FPP.vi"("VISA session"=w1816, "Num Points"=w1806, "Vg"=w1759, "Display on/off"=TRUE, "Gate Compliance"=w1805, "Drain Compliance"=w1814, "Standby"="Standby", "error in (no error)"=w1815, "Timings"=w1803, "Vd"=w1758, "Sample time"=w1796) -> ("dup VISA resource name"=w1775:refnum<visa-resource-name>, "error out"=w1774:errorcluster)  [unwired: 3 in]
        n427 = Number To Decimal String(number=w1759) -> (decimal integer string=w1785:string)  [unwired: 1 in]
        n428 = call "4155C Take Sample FPP.vi"("VISA resource name in"=w1775, "error in (no error)"=w1774, "Emergency Stop"=w1776) -> ("Time"=w1780:dbl[], "Vp1"=w1790:dbl[], "VISA Resource Name out"=w1756:refnum<visa-resource-name>, "Ig"=w1778:dbl[], "Id"=w1779:dbl[], "Vp2"=w1788:dbl[], "error out"=w1777:errorcluster)  [unwired: 10 in]
        n429 = Insert Into Array(array=dbl[][] [] ("Input Array"), new element=w1780) -> (w1794:dbl[][])  [unwired: 2 in]
        n430 = Number To Decimal String(number=w1758) -> (decimal integer string=w1783:string)  [unwired: 1 in]
        n431 = Insert Into Array(array=w1794, new element=w1779) -> (w1793:dbl[][])  [unwired: 2 in]
        n432 = Concatenate Strings("(Vg = " ("Substring"), w1785, "V, Vd = " ("Substring"), w1783, "V)" ("Substring")) -> (w1781:string)
        n433 = Insert Into Array(array=w1793, new element=w1778) -> (w1792:dbl[][])  [unwired: 2 in]
        n434 = Insert Into Array(array=w1792, new element=w1790) -> (w1789:dbl[][])  [unwired: 2 in]
        n435 = Insert Into Array(array=w1789, new element=w1788) -> (w1757:dbl[][])  [unwired: 2 in]
        n436 = Transpose 2D Array(2D array=w1757) -> (transposed array=w1787:dbl[][])
        n437 = call <vilib>:"compatOverwrite.vi"("overwrite (F)"=TRUE) -> ("overwrite?"=w1754:T8)
        n438 = Open/Create/Replace File(file path (use dialog)=w1773, error in=w1777, operation (0:open)=w1754) -> (refnum out=w1770:refnum<file>, error out=w1771:errorcluster)  [unwired: 3 in, 1 out]
        n439 = Array To Spreadsheet String(array=w1761, 3:w1765) -> (spreadsheet string=w1767:string)  [unwired: 1 in]
        n440 = Search and Replace String(replace all?=TRUE ("replace all? (F)"), input string=w1767, search string="VgVd", replace string=w1781) -> (result string=w1763:string)  [unwired: 4 in, 3 out]
        n441 = Spreadsheet String To Array(format string=w1765, spreadsheet string=w1763, array type (2D Dbl)=w1761) -> (array=w1762:string[])  [unwired: 1 in]
        n442 = call "4155C Write array to file.vi"("Byte Stream File Refnum"=w1770, "Header"=w1762, "Data Array"=w1787, "error in (no error)"=w1771) -> ("dup refnum"=w1768:refnum<file>, "error out"=w1769:errorcluster)  [unwired: 1 in]
        n443 = Close File(refnum=w1768, error in=w1769) -> (error out=w1755:errorcluster)  [unwired: 1 out]
      }
      frame "resample-fpp" {
        w1850 = string[] ["Time /s", "Id VgVd /A", "Ig VgVd /A", "Vp1 VgVd /V", "Vp2 VgVd /V"] ("Header")
        w1854 = "%d" ("format string")
        n444 = Number To Decimal String(number=w1836) -> (decimal integer string=w1894:string)  [unwired: 1 in]
        n445 = Fract/Exp String To Number(string=w1891) -> (number=w1843:dbl[])  [unwired: 3 in, 1 out]
        n446 = Concatenate Strings(w1887, "-resamplefpp-" ("Substring"), w1894, w1837, ".txt" ("Substring")) -> (w1892:string)
        n447 = String To Path(string=w1892) -> (path=w1862:path)
        n448 = Index Array(array=w1843, index=0 ("Index")) -> (element=w1849:dbl)
        n449 = Index Array(array=w1843, index=1 ("Index")) -> (element=w1848:dbl)
        n450 = Number To Decimal String(number=w1849) -> (decimal integer string=w1872:string)  [unwired: 1 in]
        n451 = call "4155C Take Sample FPP.vi"("VISA resource name in"=w1845, "error in (no error)"=w1844, "Emergency Stop"=w1863) -> ("Time"=w1867:dbl[], "Vp1"=w1877:dbl[], "VISA Resource Name out"=w1847:refnum<visa-resource-name>, "Ig"=w1865:dbl[], "Id"=w1866:dbl[], "Vp2"=w1875:dbl[], "error out"=w1864:errorcluster)  [unwired: 10 in]
        n452 = Insert Into Array(array=dbl[][] [] ("Input Array"), new element=w1867) -> (w1881:dbl[][])  [unwired: 2 in]
        n453 = Number To Decimal String(number=w1848) -> (decimal integer string=w1870:string)  [unwired: 1 in]
        n454 = Insert Into Array(array=w1881, new element=w1866) -> (w1880:dbl[][])  [unwired: 2 in]
        n455 = Concatenate Strings("(Vg = " ("Substring"), w1872, "V, Vd = " ("Substring"), w1870, "V)" ("Substring")) -> (w1868:string)
        n456 = Insert Into Array(array=w1880, new element=w1865) -> (w1879:dbl[][])  [unwired: 2 in]
        n457 = Insert Into Array(array=w1879, new element=w1877) -> (w1876:dbl[][])  [unwired: 2 in]
        n458 = Insert Into Array(array=w1876, new element=w1875) -> (w1842:dbl[][])  [unwired: 2 in]
        n459 = call <vilib>:"compatOverwrite.vi"("overwrite (F)"=TRUE) -> ("overwrite?"=w1841:T8)
        n460 = Open/Create/Replace File(file path (use dialog)=w1862, error in=w1864, operation (0:open)=w1841) -> (refnum out=w1859:refnum<file>, error out=w1860:errorcluster)  [unwired: 3 in, 1 out]
        n461 = Array To Spreadsheet String(array=w1850, 3:w1854) -> (spreadsheet string=w1856:string)  [unwired: 1 in]
        n462 = Transpose 2D Array(2D array=w1842) -> (transposed array=w1874:dbl[][])
        n463 = Search and Replace String(replace all?=TRUE ("replace all? (F)"), input string=w1856, search string="VgVd", replace string=w1868) -> (result string=w1852:string)  [unwired: 4 in, 3 out]
        n464 = Spreadsheet String To Array(format string=w1854, spreadsheet string=w1852, array type (2D Dbl)=w1850) -> (array=w1851:string[])  [unwired: 1 in]
        n465 = call "4155C Write array to file.vi"("Byte Stream File Refnum"=w1859, "Header"=w1851, "Data Array"=w1874, "error in (no error)"=w1860) -> ("dup refnum"=w1857:refnum<file>, "error out"=w1858:errorcluster)  [unwired: 1 in]
        n466 = Close File(refnum=w1857, error in=w1858) -> (error out=w1846:errorcluster)  [unwired: 1 out]
      }
      frame "serial" {
        n467 = local read "Termination char\n(0xA = '\\n' = LF)\n(0xD = '\\r' = CR)"() -> (w1922:u8)
        n468 = local read "Enable Termination\nChar (T)"() -> (w1923:bool)
        n469 = Index Array(array=w1930, index=0 ("Index")) -> (element=w1929:string)
        n470 = local read "parity"() -> (w1913:u16)
        n471 = local read "Delay before read (ms)"() -> (w1924:u32)
        n472 = local read "byte count"() -> (w1921:u32)
        n473 = local read "Timeout (ms)"() -> (w1920:u32)
        n474 = local read "VISA resource name"() -> (w1917:refnum<visa-resource-name>)
        n475 = local read "baud rate"() -> (w1916:u32)
        n476 = local read "Serial End Mode for Reads"() -> (w1915:u16)
        n477 = local read "data bits"() -> (w1914:u16)
        n478 = local read "stop bits"() -> (w1919:u16)
        n479 = local read "flow control"() -> (w1918:u16)
        n480 = call "Serial write and read v0.5.vi"("Delay before read (ms)"=w1924, "Termination char\n(0xA = '\\n' = LF)\n(0xD = '\\r' = CR)"=w1922, "Enable Termination\nChar (T)"=w1923, "parity"=w1913, "stop bits"=w1919, "string to write"=w1929, "flow control"=w1918, "byte count"=w1921, "Serial Settings:Serial End Mode for Reads"=w1915, "Timeout (ms)"=w1920, "error in (no error)"=w1935, "VISA resource name"=w1917, "baud rate"=w1916, "data bits"=w1914) -> ("Serial port output"=w1925:string, "error out"=w1934:errorcluster)
        n481 = Build Array (concatenate)(w1925, w1926) -> (w1927:string[])
      }
      frame "pump" {
        # "Time array for valve position"
        # "Time array for absolute plunger position"
        # "Valve position"
        # "Absolute plunger position"
        # "Remove \"_\""
        # "Check if hard stop is pressed."
        # "Check if halt is pressed."
        # "Check if pump is idle. Else halt."
        n482 = Index Array(array=w2000, index=0 ("Index")) -> (element=w1977:string)
        n483 = case shown="\"No error\", Default" w1975 {
          tunnel: w1977 -> [w2036 _ w2038 w2039 w2040 w2041 _ _ w2044 w2045 _]
          tunnel: [w2036 "/1H" w2038 w2039 w2040 w2041 "/1H" "/1H" w2044 w2045 "/1H"] -> w1976
          frame "No error", Default {
          }
          frame "Initialization" {
          }
          frame "Invalid command" {
          }
          frame "Invalid operand" {
          }
          frame "Device not initialized" {
          }
          frame "Internal failure" {
          }
          frame "Plunger overload" {
          }
          frame "Valve overload" {
          }
          frame "Plunger move not allowed" {
          }
          frame "A/D converter failure" {
          }
          frame "Command overflow" {
          }
        }
        n484 = local read "Hard stop pump"() -> (w1979:bool)
        n485 = local read "Halt pump"() -> (w1982:bool)
        n486 = local read "Serial End Mode for Reads"() -> (w1988:u16)
        n487 = local read "flow control"() -> (w1991:u16)
        n488 = local read "stop bits"() -> (w1992:u16)
        n489 = local read "parity"() -> (w1986:u16)
        n490 = local read "Delay before read (ms)"() -> (w1997:u32)
        n491 = local read "byte count"() -> (w1994:u32)
        n492 = local read "Timeout (ms)"() -> (w1993:u32)
        n493 = local read "VISA resource name"() -> (w1990:refnum<visa-resource-name>)
        n494 = local read "baud rate"() -> (w1989:u32)
        n495 = local read "Enable Termination\nChar (T)"() -> (w1996:bool)
        n496 = local read "Termination char\n(0xA = '\\n' = LF)\n(0xD = '\\r' = CR)"() -> (w1995:u8)
        n497 = case shown="True" w1982 {
          tunnel: [w2050 "/1H"] -> w1981
          tunnel: w1976 -> [w2050 _]
          frame False {
          }
          frame True {
            n498 = local write "Halt pump"(FALSE) -> ()
          }
        }
        n499 = case shown="True" w1979 {
          tunnel: [w2047 "/1T"] -> w1980
          tunnel: w1981 -> [w2047 _]
          frame False {
          }
          frame True {
            n500 = local write "Hard stop pump"(FALSE) -> ()
          }
        }
        n501 = local read "data bits"() -> (w1987:u16)
        n502 = String Subset(string=w1971, offset (0)=1) -> (substring=w1969:string)  [unwired: 1 in]
        n503 = call "SPM Pump v0.6.vi"("Termination char\n(0xA = '\\n' = LF)\n(0xD = '\\r' = CR)"=w1995, "Enable Termination\nChar (T)"=w1996, "Timeout (ms)"=w1993, "Serial Settings:Serial End Mode for Reads"=w1988, "byte count"=w1994, "Delay before read (ms)"=w1997, "Time <input>"=w1974, "error in (no error)"=w2005, "Serial port input"=w1980, "VISA resource name"=w1990, "parity"=w1986, "baud rate"=w1989, "stop bits"=w1992, "data bits"=w1987, "flow control"=w1991, "Time units <input>"=w1969) -> ("Input command"=w1968:string, "Serial port data"=w1958:string[], "Pump status"=w1964:string, "Valve position"=w1966:i32, "Absolute plunger position"=w1978:i32, "Serial port"=w1973:string, "error out"=w2004:errorcluster)  [unwired: 1 in, 4 out]
        n504 = case shown="\"?6\"" w1968 {
          tunnel: [w2017 w2025 w2031] -> w1985
          tunnel: w1984 -> [w2017 w2024 w2031]
          tunnel: w1978 -> [_ w2023 _]
          tunnel: w1965 -> [w2016 w2022 w2032]
          tunnel: [w2016 w2022 w2034] -> w1967
          tunnel: w1966 -> [_ _ w2033]
          tunnel: w1963 -> [_ w2021 w2029]
          tunnel: w1962 -> [w2015 w2020 w2030]
          tunnel: [w2015 w2019 w2030] -> w1961
          tunnel: [w2014 w2018 w2028] -> w1960
          tunnel: w1959 -> [w2014 w2018 w2027]
          frame "Q", Default {
          }
          frame "?" {
            n505 = Build Array (concatenate)(w2024, w2023) -> (w2025:i32[])
            n506 = Build Array (concatenate)(w2020, w2021) -> (w2019:i32[])
            n507 = call "4155C Split array.vi"("X data in"=w2019, "Y1 data in"=w2025) -> ("Array of clusters"=w2026:cluster{"Y data in":dbl[], "X data in":dbl[]}[])  [unwired: 5 in, 1 out]
            n508 = local write "Absolute plunger position vs time"(w2026) -> ()
          }
          frame "?6" {
            n509 = Build Array (concatenate)(w2032, w2033) -> (w2034:i32[])
            n510 = Build Array (concatenate)(w2027, w2029) -> (w2028:i32[])
            n511 = call "4155C Split array.vi"("X data in"=w2028, "Y1 data in"=w2034) -> ("Array of clusters"=w2035:cluster{"Y data in":dbl[], "X data in":dbl[]}[])  [unwired: 5 in, 1 out]
            n512 = local write "Valve position vs time"(w2035) -> ()
          }
        }
        n513 = Build Array (concatenate)(w1956, w1958) -> (w1957:string[][])
        n514 = Build Array (concatenate)(w1972, w1973) -> (w1998:string[])
      }
      frame "filename" {
        n515 = Index Array(array=w2054, index=0 ("Index")) -> (element=w2053:string)
      }
    }
    n516 = local read "Time Units"() -> (w66:u16)
    n517 = case shown="2" w66 {
      tunnel: ["Time (Seconds)" ("element") "Time (Minutes)" ("element") "Time (Hours)" ("element")] -> w106
      frame 0 {
      }
      frame 1, Default {
      }
      frame 2 {
      }
    }
    n518 = Build Array(w145, w74, w84, w83, w82, w81, w80, w79, w78, w77, w76, w75, w73) -> (w184:dbl[][])
    n519 = Transpose 2D Array(2D array=w184) -> (transposed array=w183:dbl[][])
    n520 = Concatenate Strings(w125, w68, "Imax_Imin_Ion_Ioff_vs_time.txt" ("Suffix (Imax,Imin,Ion,Ioff)")) -> (w194:string)
    n521 = Build Array(w106, "Is max (A)" ("VAR2 Name"), "Is min (A)" ("VAR2 Name"), "Id max (A)" ("VAR2 Name"), "Id min (A)" ("VAR2 Name"), "Ig max (A)" ("VAR2 Name"), "Ig min (A)" ("VAR2 Name"), "Is on (A)" ("VAR2 Name"), "Is off (A)" ("VAR2 Name"), "Id on (A)" ("VAR2 Name"), "Id off (A)" ("VAR2 Name"), "Ig on (A)" ("VAR2 Name"), "Ig off (A)" ("VAR2 Name")) -> (w189:string[])
    n522 = Array To Spreadsheet String(array=w183, 3:"%e" ("format string")) -> (spreadsheet string=w187:string)  [unwired: 1 in]
    n523 = Array To Spreadsheet String(array=w189, 3:"" ("format string")) -> (spreadsheet string=w188:string)  [unwired: 1 in]
    n524 = String To Path(string=w194) -> (path=w193:path)
    n525 = Build Array(w188, w187) -> (w186:string[])
    n526 = Write to Text File(file (use dialog)=w193, text=w186, error in=w141) -> (refnum out=w195:refnum<file>, error out=w185:errorcluster)  [unwired: 1 in, 1 out]
    n527 = Close File(refnum=w195, error in=w185) -> (error out=w124:errorcluster)  [unwired: 1 out]
    n528 = Build Array(w120, w146) -> (w151:i32[][])
    n529 = Build Array(w106, "Absolute plunger position" ("VAR2 Name")) -> (w154:string[])
    n530 = Transpose 2D Array(2D array=w151) -> (transposed array=w144:i32[][])
    n531 = Array To Spreadsheet String(array=w154, 3:"" ("format string")) -> (spreadsheet string=w153:string)  [unwired: 1 in]
    n532 = Array To Spreadsheet String(array=w144, 3:"%e" ("format string")) -> (spreadsheet string=w150:string)  [unwired: 1 in]
    n533 = Build Array(w153, w150) -> (w156:string[])
    n534 = Concatenate Strings(w125, w68, "plunger_vs_time.txt" ("Suffix (plunger)")) -> (w148:string)
    n535 = String To Path(string=w148) -> (path=w147:path)
    n536 = Write to Text File(file (use dialog)=w147, text=w156, error in=w124) -> (refnum out=w149:refnum<file>, error out=w158:errorcluster)  [unwired: 1 in, 1 out]
    n537 = Close File(refnum=w149, error in=w158) -> (error out=w123:errorcluster)  [unwired: 1 out]
    n538 = Concatenate Strings(w125, w68, "serial_port_output.txt" ("Suffix (serial port log)")) -> (w164:string)
    n539 = String To Path(string=w164) -> (path=w163:path)
    n540 = Build Array(w106, "Serial port input" ("VAR2 Name"), "Pump status" ("VAR2 Name"), "Serial port output: ") -> (w110:string[])
    n541 = Array To Spreadsheet String(array=w116, 3:"" ("format string")) -> (spreadsheet string=w107:string)  [unwired: 1 in]
    n542 = Array To Spreadsheet String(array=w110, 3:"" ("format string")) -> (spreadsheet string=w108:string)  [unwired: 1 in]
    n543 = Build Array(w108, w107) -> (w109:string[])
    n544 = Array To Spreadsheet String(array=w115, 3:"" ("format string")) -> (spreadsheet string=w169:string)  [unwired: 1 in]
    n545 = Write to Text File(file (use dialog)=w163, text=w109, error in=w123) -> (refnum out=w165:refnum<file>, error out=w166:errorcluster)  [unwired: 1 in, 1 out]
    n546 = Close File(refnum=w165, error in=w166) -> (error out=w122:errorcluster)  [unwired: 1 out]
    n547 = local write "Serial port data"(w169) -> ()
    n548 = Build Array(w119, w127) -> (w133:i32[][])
    n549 = Build Array(w106, "Valve port" ("VAR2 Name")) -> (w136:string[])
    n550 = Transpose 2D Array(2D array=w133) -> (transposed array=w128:i32[][])
    n551 = Array To Spreadsheet String(array=w136, 3:"" ("format string")) -> (spreadsheet string=w135:string)  [unwired: 1 in]
    n552 = Array To Spreadsheet String(array=w128, 3:"%e" ("format string")) -> (spreadsheet string=w132:string)  [unwired: 1 in]
    n553 = Build Array(w135, w132) -> (w138:string[])
    n554 = Concatenate Strings(w125, w68, "valve_port_vs_time.txt" ("Suffix (valve)")) -> (w130:string)
    n555 = String To Path(string=w130) -> (path=w129:path)
    n556 = Write to Text File(file (use dialog)=w129, text=w138, error in=w122) -> (refnum out=w131:refnum<file>, error out=w140:errorcluster)  [unwired: 1 in, 1 out]
    n557 = Close File(refnum=w131, error in=w140) -> (error out=w121:errorcluster)  [unwired: 1 out]
  }
  "error out" <- w28
  "Timings Indicator" <- w10
  "Is max" <- w8
  "Id max" <- w8
  "Ig max" <- w8
  "Imax vs time" <- w4
  "I vs Vg" <- w4
  "Imin vs time" <- w4
  "I vs Vd" <- w4
  "Serial port data" <- "" ("Serial port data")
  "Valve position vs time" <- cluster{"Y data in":dbl[], "X data in":dbl[]}[] [] ("Valve position vs time")
  "Is min" <- w7
  "Id min" <- w7
  "Ig min" <- w7
  "Ion vs time" <- w4
  "Ioff vs time" <- w4
  "Is on" <- w6
  "Id on" <- w6
  "Ig on" <- w6
  "Is off" <- w5
  "Id off" <- w5
  "Ig off" <- w5
